vi "Text control 2 v6.3_pump-specific.vi"() -> ()   [LabVIEW 2016]
panel:
  in  "Tab Control":enum32{"Main", "Other parameters"}(tab)
  out "Line running":i32
  out "Total lines":i32
  out "Path":path=path "C:/users/rlp38/09Apr2009LTtesting/test2.txt"
  out "I vs Vg":cluster{"Y data in":dbl[], "X data in":dbl[]}[](graph)
  out "Is max":dbl format="%.2e"
  out "Id max":dbl format="%.2e"
  out "Ig max":dbl format="%.2e"
  out "Imax vs time":cluster{"Y data in":dbl[], "X data in":dbl[]}[](graph)
  out "Imin vs time":cluster{"Y data in":dbl[], "X data in":dbl[]}[](graph)
  out "I vs Vd":cluster{"Y data in":dbl[], "X data in":dbl[]}[](graph)
  in  "Script":string="#-------------------------------------------------------\n# SPM pump cleaning script\n#\n# Version 0.5\n# Author: Dimitrios Simatos\n# Last updated: 2018-01-05\n#-------------------------------------------------------\n# Description\n#\n# This script is designed to run the cleaning sequence of the SPM OEM pump.\n# This script needs to be run 4 times!\n#-------------------------------------------------------\n# Changes\n#\n# Placed initialization and hard stop commands in the beginning.\n#-------------------------------------------------------\n# Important points\n#\n# Never leave any liquid in the pump to dry after the experiments. If they dry, the residue may block the valve.\n# Always run the cleaning cycle after the experiments.\n# Use clockwise rotation when going up in valve port numbers and vice versa.\n#-------------------------------------------------------\n# Things to do before running the script\n#\n# Set time units to minutes.\n# Set filenames.\n# Replace the tubing, if necessary.\n#-------------------------------------------------------\n# Port connections\n#\n# Port 1: Waste\n# Port 2: Waste\n# Port 3: Various cleaning liquids\n# Port 4: Waste\n# Port 5: Waste\n# Port 6: Waste\n#\n# Between each of the 4 runs, the settings of Port 3 will change, according to the cleaning protocol.\n# The settings for Port 3 are:\n# 1st run: 1% v/v solution of sodium hypochlorite in ultrapure water\n# 2nd run: 0.1% w/v solution of sodium dodecyl sulfate in ultrapure water\n# 3rd run: Ultrapure water\n# 4th run: Waste (in air, not immersed in liquid)\n#-------------------------------------------------------\n# Cleaning protocol for the SPM OEM pump (from the manual)\n#\n# A cleaning procedure should be performed at the end of each day or in between two different experiments.\n# An effective cleaning can be performed in the following manner:\n# • Bleach solution to kill microorganisms\n# 1. Prepare a solution of 1% chlorine bleach and deionized water\n#    NOTE: Prepare a 1% v/v solution of sodium hypochlorite in deionized water\n# 2. Prepare a reservoir and place 1 tubing in the bleach solution and 5 tubings in a waste recipient\n# 3. Pick up the bleach solution through 1 port to entirely fill the syringe\n# 4. Sequentially output the syringe content through the remaining ports and throw it to the waste\n# 5. Repeat operation at least 2 times\n# • Detergent solution to remove debris\n# 1. Prepare a solution of 0.1% detergent and deionized water\n#    NOTE: Prepare a 0.1% w/v solution of sodium dodecyl sulfate in deionized water\n# 2. Move the tubing from the bleach solution reservoir and place it into a reservoir of detergent solution\n# 3. Pick up the detergent solution through 1 port to entirely fill the syringe\n# 4. Sequentially output the detergent solution through the remaining ports into the waste recipient\n# 5. Repeat operation at least 2 times\n# • Rinsing water to prepare the pump for your next experiment\n# 1. Move the tubing from the detergent solution reservoir and place it into a reservoir of deionized water\n# 2. Pick up the rinsing solution through 1 port to entirely fill the syringe\n# 3. Sequentially output the rinse water through the remaining ports into the waste recipient\n# 4. Repeat operation at least 2 times\n# • Replace the tubing, if necessary\n#-------------------------------------------------------\n# Pumping cycles and execution time\n#\n# Execution time for a single cycle: 6 x (1 min + 10 sec) = 7 minutes\n# Total execution time: 4 x 7 = 28 minutes\n# Since the script has to run 4 times, the cleaning lasts for: 4 x 28 = 112 minutes\n# Air must be the last to be pumped through the valve, to remove all liquids.\n# There are 4 pumping cycles. Each one draws a different liquid through port 3 and pumps it sequentially through ports 1,2,4,5,6.\n# During the sequential pumping, each port receives 200 ml of liquid (20% of the total syringe volume = 600 \"plunger units\")\n# The device must be disconnected from the port during the cleaning procedure.\n# All cycles are similar, except cycle 1 has the initialization command uncommented and the first report valve command commented.\n#-------------------------------------------------------\n# Volume of liquid needed\n#\n# Volume of liquid needed per cycle: 1 ml\n# Total volume of liquid needed per script run: 4 x 1 = 4 ml\n# Since the script has to run 4 times, the first 3 with different liquids, I need:\n# 4 ml of 1% v/v solution of sodium hypochlorite in ultrapure water\n# 4 ml of 0.1% w/v solution of sodium dodecyl sulfate in ultrapure water\n# 4 ml of ultrapure water\n#-------------------------------------------------------\n# Parameters\n#\n# Syringe size: 1 ml\n# Step resolution N = 0.01 mm\n# Drawing flow V = 300 pulses/second (6000 ul/min)\n# Pumping flow V = 300 pulses/second (6000 ul/min)\n#-------------------------------------------------------\n# Pump initialization\npump /1T #hard stop pump\npump /1ZR #initialize pump\n#-------------------------------------------------------\n# Cycle 1\n# Fill the syringe\npump /1Q #query pump\npump /1? #report absolute plunger position\n#pump /1?6 #report valve position\nwait-min 1 #wait 1 minute\npump /1N0R #set step resolution: 0.01 mm\npump /1Q #query pump\npump /1? #report absolute plunger position (the plunger should be at 0)\npump /1?6 #report valve position\nwait 1000 #wait 1 second\npump /1V300R #choose speed: 300 steps/s (6000 ul/min)\npump /1Q #query pump\nwait 1000 #wait 1 second\npump /1I3R #go to port 3, clockwise rotation\npump /1Q #query pump\npump /1?6 #report valve position\nwait 1000 #wait 1 second\npump /1A3000R #go to absolute position 3000 (= draw 1 ml)\nwait 30000 #wait 30 seconds\npump /1Q #query pump\npump /1? #report absolute plunger position (the plunger should have finished moving)\n#pump /1?6 #report valve position\n# The sequential pumping begins\n# Port 1\npump /1O1R #switch to port 1, counterclockwise rotation\npump /1Q #query pump\npump /1?6 #report valve position\npump /1A2400R #go to absolute position 2400 (= pump 200 ul)\npump /1Q #query pump\npump /1? #report absolute plunger position (the plunger should be moving to 0)\nwait-min 1 #wait 1 minute\npump /1? #report absolute plunger position (the plunger should have finished moving)\n# Port 2\npump /1I2R #switch to port 2, clockwise rotation\npump /1Q #query pump\npump /1?6 #report valve position\npump /1A1800R #go to absolute position 1800 (= pump 200 ul)\npump /1Q #query pump\npump /1? #report absolute plunger position (the plunger should be moving to 0)\nwait-min 1 #wait 1 minute\npump /1? #report absolute plunger position (the plunger should have finished moving)\n# Port 4\npump /1I4R #switch to port 4, clockwise rotation\npump /1Q #query pump\npump /1?6 #report valve position\npump /1A1200R #go to absolute position 1200 (= pump 200 ul)\npump /1Q #query pump\npump /1? #report absolute plunger position (the plunger should be moving to 0)\nwait-min 1 #wait 1 minute\npump /1? #report absolute plunger position (the plunger should have finished moving)\n# Port 5\npump /1I5R #switch to port 5, clockwise rotation\npump /1Q #query pump\npump /1?6 #report valve position\npump /1A600R #go to absolute position 600 (= pump 200 ul)\npump /1Q #query pump\npump /1? #report absolute plunger position (the plunger should be moving to 0)\nwait-min 1 #wait 1 minute\npump /1? #report absolute plunger position (the plunger should have finished moving)\n# Port 6\npump /1I6R #switch to port 6, clockwise rotation\npump /1Q #query pump\npump /1?6 #report valve position\npump /1A0R #go to absolute position 0 (= pump 200 ul)\npump /1Q #query pump\npump /1? #report absolute plunger position (the plunger should be moving to 0)\nwait-min 1 #wait 1 minute\npump /1? #report absolute plunger position (the plunger should have finished moving)\n#-------------------------------------------------------\n# Cycle 2\n# Fill the syringe\n#pump /1ZR #initialize pump\npump /1Q #query pump\npump /1? #report absolute plunger position\npump /1?6 #report valve position\nwait-min 1 #wait 1 minute\npump /1N0R #set step resolution: 0.01 mm\npump /1Q #query pump\npump /1? #report absolute plunger position (the plunger should be at 0)\npump /1?6 #report valve position\nwait 1000 #wait 1 second\npump /1V300R #choose speed: 300 steps/s (6000 ul/min)\npump /1Q #query pump\nwait 1000 #wait 1 second\npump /1O3R #go to port 3, counterclockwise rotation\npump /1Q #query pump\npump /1?6 #report valve position\nwait 1000 #wait 1 second\npump /1A3000R #go to absolute position 3000 (= draw 1 ml)\nwait 30000 #wait 30 seconds\npump /1Q #query pump\npump /1? #report absolute plunger position (the plunger should have finished moving)\n#pump /1?6 #report valve position\n# The sequential pumping begins\n# Port 1\npump /1O1R #switch to port 1, counterclockwise rotation\npump /1Q #query pump\npump /1?6 #report valve position\npump /1A2400R #go to absolute position 2400 (= pump 200 ul)\npump /1Q #query pump\npump /1? #report absolute plunger position (the plunger should be moving to 0)\nwait-min 1 #wait 1 minute\npump /1? #report absolute plunger position (the plunger should have finished moving)\n# Port 2\npump /1I2R #switch to port 2, clockwise rotation\npump /1Q #query pump\npump /1?6 #report valve position\npump /1A1800R #go to absolute position 1800 (= pump 200 ul)\npump /1Q #query pump\npump /1? #report absolute plunger position (the plunger should be moving to 0)\nwait-min 1 #wait 1 minute\npump /1? #report absolute plunger position (the plunger should have finished moving)\n# Port 4\npump /1I4R #switch to port 4, clockwise rotation\npump /1Q #query pump\npump /1?6 #report valve position\npump /1A1200R #go to absolute position 1200 (= pump 200 ul)\npump /1Q #query pump\npump /1? #report absolute plunger position (the plunger should be moving to 0)\nwait-min 1 #wait 1 minute\npump /1? #report absolute plunger position (the plunger should have finished moving)\n# Port 5\npump /1I5R #switch to port 5, clockwise rotation\npump /1Q #query pump\npump /1?6 #report valve position\npump /1A600R #go to absolute position 600 (= pump 200 ul)\npump /1Q #query pump\npump /1? #report absolute plunger position (the plunger should be moving to 0)\nwait-min 1 #wait 1 minute\npump /1? #report absolute plunger position (the plunger should have finished moving)\n# Port 6\npump /1I6R #switch to port 6, clockwise rotation\npump /1Q #query pump\npump /1?6 #report valve position\npump /1A0R #go to absolute position 0 (= pump 200 ul)\npump /1Q #query pump\npump /1? #report absolute plunger position (the plunger should be moving to 0)\nwait-min 1 #wait 1 minute\npump /1? #report absolute plunger position (the plunger should have finished moving)\n#-------------------------------------------------------\n# Cycle 3\n# Fill the syringe\n#pump /1ZR #initialize pump\npump /1Q #query pump\npump /1? #report absolute plunger position\npump /1?6 #report valve position\nwait-min 1 #wait 1 minute\npump /1N0R #set step resolution: 0.01 mm\npump /1Q #query pump\npump /1? #report absolute plunger position (the plunger should be at 0)\npump /1?6 #report valve position\nwait 1000 #wait 1 second\npump /1V300R #choose speed: 300 steps/s (6000 ul/min)\npump /1Q #query pump\nwait 1000 #wait 1 second\npump /1O3R #go to port 3, counterclockwise rotation\npump /1Q #query pump\npump /1?6 #report valve position\nwait 1000 #wait 1 second\npump /1A3000R #go to absolute position 3000 (= draw 1 ml)\nwait 30000 #wait 30 seconds\npump /1Q #query pump\npump /1? #report absolute plunger position (the plunger should have finished moving)\n#pump /1?6 #report valve position\n# The sequential pumping begins\n# Port 1\npump /1O1R #switch to port 1, counterclockwise rotation\npump /1Q #query pump\npump /1?6 #report valve position\npump /1A2400R #go to absolute position 2400 (= pump 200 ul)\npump /1Q #query pump\npump /1? #report absolute plunger position (the plunger should be moving to 0)\nwait-min 1 #wait 1 minute\npump /1? #report absolute plunger position (the plunger should have finished moving)\n# Port 2\npump /1I2R #switch to port 2, clockwise rotation\npump /1Q #query pump\npump /1?6 #report valve position\npump /1A1800R #go to absolute position 1800 (= pump 200 ul)\npump /1Q #query pump\npump /1? #report absolute plunger position (the plunger should be moving to 0)\nwait-min 1 #wait 1 minute\npump /1? #report absolute plunger position (the plunger should have finished moving)\n# Port 4\npump /1I4R #switch to port 4, clockwise rotation\npump /1Q #query pump\npump /1?6 #report valve position\npump /1A1200R #go to absolute position 1200 (= pump 200 ul)\npump /1Q #query pump\npump /1? #report absolute plunger position (the plunger should be moving to 0)\nwait-min 1 #wait 1 minute\npump /1? #report absolute plunger position (the plunger should have finished moving)\n# Port 5\npump /1I5R #switch to port 5, clockwise rotation\npump /1Q #query pump\npump /1?6 #report valve position\npump /1A600R #go to absolute position 600 (= pump 200 ul)\npump /1Q #query pump\npump /1? #report absolute plunger position (the plunger should be moving to 0)\nwait-min 1 #wait 1 minute\npump /1? #report absolute plunger position (the plunger should have finished moving)\n# Port 6\npump /1I6R #switch to port 6, clockwise rotation\npump /1Q #query pump\npump /1?6 #report valve position\npump /1A0R #go to absolute position 0 (= pump 200 ul)\npump /1Q #query pump\npump /1? #report absolute plunger position (the plunger should be moving to 0)\nwait-min 1 #wait 1 minute\npump /1? #report absolute plunger position (the plunger should have finished moving)\n#-------------------------------------------------------\n# Cycle 4\n# Fill the syringe\n#pump /1ZR #initialize pump\npump /1Q #query pump\npump /1? #report absolute plunger position\npump /1?6 #report valve position\nwait-min 1 #wait 1 minute\npump /1N0R #set step resolution: 0.01 mm\npump /1Q #query pump\npump /1? #report absolute plunger position (the plunger should be at 0)\npump /1?6 #report valve position\nwait 1000 #wait 1 second\npump /1V300R #choose speed: 300 steps/s (6000 ul/min)\npump /1Q #query pump\nwait 1000 #wait 1 second\npump /1O3R #go to port 3, counterclockwise rotation\npump /1Q #query pump\npump /1?6 #report valve position\nwait 1000 #wait 1 second\npump /1A3000R #go to absolute position 3000 (= draw 1 ml)\nwait 30000 #wait 30 seconds\npump /1Q #query pump\npump /1? #report absolute plunger position (the plunger should have finished moving)\n#pump /1?6 #report valve position\n# The sequential pumping begins\n# Port 1\npump /1O1R #switch to port 1, counterclockwise rotation\npump /1Q #query pump\npump /1?6 #report valve position\npump /1A2400R #go to absolute position 2400 (= pump 200 ul)\npump /1Q #query pump\npump /1? #report absolute plunger position (the plunger should be moving to 0)\nwait-min 1 #wait 1 minute\npump /1? #report absolute plunger position (the plunger should have finished moving)\n# Port 2\npump /1I2R #switch to port 2, clockwise rotation\npump /1Q #query pump\npump /1?6 #report valve position\npump /1A1800R #go to absolute position 1800 (= pump 200 ul)\npump /1Q #query pump\npump /1? #report absolute plunger position (the plunger should be moving to 0)\nwait-min 1 #wait 1 minute\npump /1? #report absolute plunger position (the plunger should have finished moving)\n# Port 4\npump /1I4R #switch to port 4, clockwise rotation\npump /1Q #query pump\npump /1?6 #report valve position\npump /1A1200R #go to absolute position 1200 (= pump 200 ul)\npump /1Q #query pump\npump /1? #report absolute plunger position (the plunger should be moving to 0)\nwait-min 1 #wait 1 minute\npump /1? #report absolute plunger position (the plunger should have finished moving)\n# Port 5\npump /1I5R #switch to port 5, clockwise rotation\npump /1Q #query pump\npump /1?6 #report valve position\npump /1A600R #go to absolute position 600 (= pump 200 ul)\npump /1Q #query pump\npump /1? #report absolute plunger position (the plunger should be moving to 0)\nwait-min 1 #wait 1 minute\npump /1? #report absolute plunger position (the plunger should have finished moving)\n# Port 6\npump /1I6R #switch to port 6, clockwise rotation\npump /1Q #query pump\npump /1?6 #report valve position\npump /1A0R #go to absolute position 0 (= pump 200 ul)\npump /1Q #query pump\npump /1? #report absolute plunger position (the plunger should be moving to 0)\nwait-min 1 #wait 1 minute\npump /1? #report absolute plunger position (the plunger should have finished moving)\n#-------------------------------------------------------"
  out "Command running:":string
  out "Serial port data":string
  out "Elapsed Time":dbl caption="Elapsed Time (s)"
  in  "Time Units":u16(ring)=1 items=["Seconds", "Minutes", "Hours"]
  in  "Time Offset":dbl caption="Set Start Time (s)"
  in  "Reset":bool
  in  "Auto Reset":bool
  in  "integration time":u32(slide) max=2 step=1 scale=0.0..2.0
  in  "Interrupt scan":bool
  out "Absolute plunger position vs time":cluster{"Y data in":dbl[], "X data in":dbl[]}[](graph)
  out "Valve position vs time":cluster{"Y data in":dbl[], "X data in":dbl[]}[](graph)
  out "Is on":dbl format="%.2e"
  out "Id on":dbl format="%.2e"
  out "Ig on":dbl format="%.2e"
  out "Ion vs time":cluster{"Y data in":dbl[], "X data in":dbl[]}[](graph)
  out "Ioff vs time":cluster{"Y data in":dbl[], "X data in":dbl[]}[](graph)
  out "Ig min":dbl format="%.2e"
  out "Id min":dbl format="%.2e"
  out "Is min":dbl format="%.2e"
  out "Is off":dbl format="%.2e"
  out "Id off":dbl format="%.2e"
  out "Ig off":dbl format="%.2e"
  in  "Integration time (long)":dbl=0.32 min=0.04 max=2.0 step=0.02 format="%.2f"
  in  "Integration time (short)":dbl=0.0019 min=8e-05 max=0.0019 step=8e-05 format="%^.0e"
  in  "Gate: Compliance":dbl=0.001 format="%.8f"
  in  "Drain: Compliance":dbl=0.001 format="%.8f"
  in  "Hard stop pump":bool
  in  "Halt pump":bool
  in  "Interrupt program":bool
  in  "Suffix (script)":string="step_1_up-H2O_initial_script.txt"
  in  "Filename (variable part)":string="step_1_up-H2O_initial_"
  in  "Gate Range\nmode":u16(ring) items=["Auto", "Limited", "Fixed"]
  in  "Gate Range":u8(slide)=6 max=11 scale=0.0..11.0
  in  "Source/Drain\nRange mode":u16(ring) items=["Auto", "Limited", "Fixed"]
  in  "Source/Drain Range":u8(slide)=6 max=11 scale=0.0..11.0
  in  "Panel Controls":T1={"Emergency Stop"=refnum, "TransGraph Max"=1e-05, "Text/Graph (text=false)"=TRUE} {"TransGraph Max" format="%.2e"}
  in  "Panel Controls 2":T2={"Emergency Stop"=refnum, "TransGraph Max"=1e-05, "Text/Graph (text=false)"=TRUE, "TransGraph Min"=1e-11} {"TransGraph Min" format="%.2e"; "TransGraph Max" format="%.2e"}
  in  "SMU4":cluster{"on/off":bool, "Voltage":dbl} {"Voltage" min=-100.0 max=100.0 format="%.2f"}
  in  "Full Reset":bool
  in  "Standby":T3
  out "error out":errorcluster
  in  "Delay before read (ms)":u32=1000
  in  "byte count":u32=64
  in  "Serial End Mode for Reads":u16(ring)=2 items=["None", "LastBit", "TermChar"]
  in  "Timeout (ms)":u32=10000
  in  "Enable Termination\nChar (T)":bool=TRUE
  in  "Termination char\n(0xA = '\\n' = LF)\n(0xD = '\\r' = CR)":u8=13 format="%.0x"
  in  "flow control":u16(ring) items=["None"=0, "XON/XOFF"=1, "RTS/CTS"=2, "DTR/DSR"=4]
  in  "stop bits":u16(ring)=10 items=["1.0"=10, "1.5"=15, "2.0"=20]
  in  "parity":u16(ring) items=["None", "Odd", "Even", "Mark", "Space"]
  in  "data bits":u16=8 min=5 max=8 step=1
  in  "VISA resource name":refnum<visa-resource-name>="COM6"
  in  "baud rate":u32=9600
  out "Timings Indicator":T4
  in  "Timings (overwritten by the Front Panel)":T5={"integration time"=0, "Short/Long integration time"=0.00064, "hold time (sec)"=0.0, "delay time (sec)"=0.0, "Step Time (0 disables)"=0.0, "sweep method"=0, "Pulse period"=0.005, "Base voltage"=0.0, "Pulse width"=0.0005} {"Pulse width" min=0.0005 max=0.1 step=0.0001 format="%.4f"; "Base voltage" format="%^.4e"; "Pulse period" min=0.005 max=1.0 step=0.0001 format="%.4f"; "sweep method" items=["Continuous", "Pulsed"]; "Step Time (0 disables)" format="%.2f"; "delay time (sec)" format="%.4f"; "hold time (sec)" format="%.4f"; "Short/Long integration time" format="%^.0e"; "integration time" scale=0.0..2.0}
  in  "Gate":T6={"Gate Start"=0.0, "Gate Stop"=2.0, "Gate Step (linear only)"=1.0, "Gate Compliance"=0.0001, "Gate PComp"=0.0, "Range mode"=0, "Range"=6} {"Range" max=11 scale=0.0..11.0; "Range mode" items=["Auto", "Limited", "Fixed"]; "Gate PComp" format="%^.2e"; "Gate Compliance" format="%^.2e"; "Gate Step (linear only)" format="%^.4e"; "Gate Stop" format="%^.4e"; "Gate Start" format="%^.4e"}
  in  "Drain 2":T7={"Drain Start"=0.0, "Drain Stop"=2.0, "Drain Compliance"=0.0001, "Drain Step"=1.0, "Drain PComp"=0.0, "Range mode"=0, "Range"=6} {"Range" max=11 scale=0.0..11.0; "Range mode" items=["Auto", "Limited", "Fixed"]; "Drain PComp" format="%^.2e"; "Drain Step" format="%^.4e"; "Drain Compliance" format="%^.2e"; "Drain Stop" format="%^.4e"; "Drain Start" format="%^.4e"}
  # "Syntax:\nitime [s|m|l] time(sec): [s|m|l] determines the integration time setting (small|medium|long) and time sets the value.\nNOTE: The value of the integration time has to be within the range allowed by its category (s|m|l), otherwise, the closest value will be used. (e.g. if the category is set to short but the time value is very long, the actual value used will be the maximum short integration time.\nIntegration times:\n    Short: Default: 640 us. Range: 8E-5 - 1.92E-3 seconds.\n    Medium: Fixed at 1 NPL cycle (0.02 seconds).\n    Long: Default: 16 NPL cycles (0.32 seconds). Range: 2-100 NPL cycles (0.04 seconds - 2 seconds).\ngaterangemode [a|l|f]\ndrainrangemode [a|l|f]\npulsed [on|off] PulsePeriod(sec) PulseBaseVoltage PulseONWidth(sec)\nstandby [on l off]\nwait NumMilliseconds\nwait-min NumMinutes\n# texthere = comment\ntransfer [s|d] VgStart VgStop VgStep VdStart VdStop VdStep\noutput [s|d] VgStart VgStop VgStep VdStart VdStop VdStep\nsample Vg Vd NumSamples Time(s) SampleInterval(s)\nsamplei Idg NumSamples Time(s) SampleInterval(s) VDGcompliance\n100 samples is approximately 13 seconds with medium integration\n# if in doubt use SampleInterval(s) = 0.004\nstressV VG VD IGcompliance IDcompliance Duration(sec)\nstressI IDG VDGcompliance Duration(sec)\nvsu2pulse Bias Duration(s)\npulsedstressV [s|d] VEstop VgON VgOFF Period(s) PulseONwidth(s) Vd\nsample-fpp Vg Vd NumSamples Time\nresample-fpp Vg Vd\ntransfer-fpp [s|d] VgStart VgStop VgStep VdStart VdStop VdStep\noutput-fpp [s|d] VgStart VgStop VgStep VdStart VdStop VdStep\nserial SerialPortCommand\npump SerialPortCommand for the SPM pump\n\nSPM Pump Syntax (<x>: pump number, use 1 if only one pump):\nif the command syntax contains [R], then append the letter R to the command\n/<x>Q: query (a query command should follow each command)\n/<x>Z[R] or /<x>Y[R]: initialize pump\n/<x>N<n>[R] (<n>=0,1): <0> (<1>) microstep 0.01 mm (0.00125 mm) resolution\n/<x>I<n> (<n>=0-6): turn to port number n (clockwise)\n/<x>O<n> (<n>=0-6): turn to port number n (counterclockwise)\n/<x>X: Re-execute last command string\n/<x>G<n>[R] (<n>=0-60000): repeat command sequence (default: 0, 0=loop forever)\n/<x>g: Mark the start of a repeat sequence (max = 10)\n/<x>M<n>[R] (<n>=0-86400000): delay command execution by n milliseconds\n/<x>H: Halt; Pause the sequence after finishing the current move\n/<x>T: Hardstop; Interrupt the current move and suppress it from the sequence\n/<x>A<n>[R] (<n>=0-3000 with N=0, 0-24000 with N=1): absolute position\n/<x>P<n>[R] (<n>=0-3000 with N=0, 0-24000 with N=1): relative pickup\n/<x>D<n>[R] (<n>=0-3000 with N=0, 0-24000 with N=1): relative dispense\n/<x>V<n>[R] (<n>=1-1600 default: 150): set peak speed (pulses/sec)\nNOTE: The lowest speed limit is 1 pulse/sec, not 5, as the manual states.\n/<x>S<n>[R] (<n>=10-40 default: 22): set speed (NOT in pulses/sec, look in manual)\nNOTE: When controlled with absolute position, one does not need to pay special attention to the syringe that is mounted on the pump.\nWithdraw from lower stage (ports 3, 5), dispense from higher stage (ports 2, 4, 6).\nConnect Port 1 to waste."
  # "Time"
  # "1\n2\n3\n4\n5\n6\n7\n8\n9\n10\n11\n12\n13\n14\n15\n16\n17\n18\n19\n20"
  # "Serial port settings"
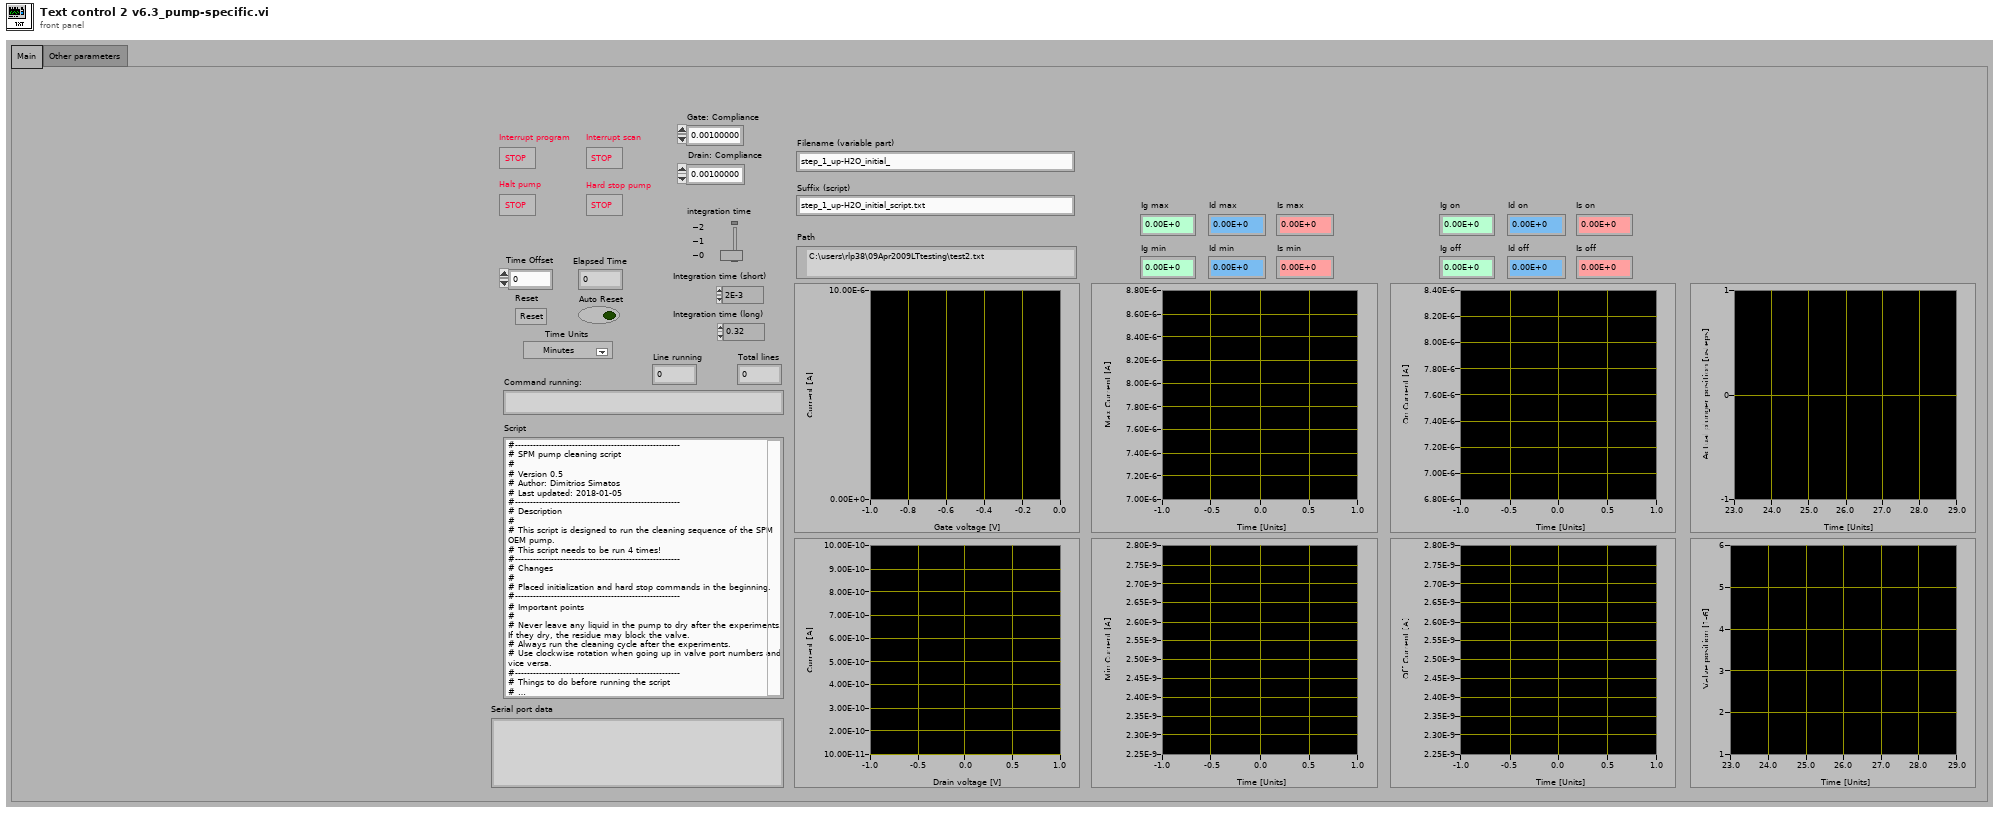
[diagram p1: front panel]
types:
  T1 = cluster{"Emergency Stop":refnum<vi>, "TransGraph Max":dbl, "Text/Graph (text=false)":bool}
  T2 = cluster{"Emergency Stop":refnum<vi>, "TransGraph Max":dbl, "Text/Graph (text=false)":bool, "TransGraph Min":dbl}
  T3 = cluster{"Gate Standby":bool, "Drain Standby":bool}
  T4 = cluster{"integration time (0:s, 1:m, 2:l)":u32, "Short/Long integration time":dbl, "hold time (sec)":dbl, "delay time (sec)":dbl, "Step Time (0 disables)":dbl, "sweep method":u16, "Pulse period":dbl, "Base voltage":dbl, "Pulse width":dbl}
  T5 = cluster{"integration time":u32, "Short/Long integration time":dbl, "hold time (sec)":dbl, "delay time (sec)":dbl, "Step Time (0 disables)":dbl, "sweep method":u16, "Pulse period":dbl, "Base voltage":dbl, "Pulse width":dbl}
  T6 = cluster{"Gate Start":dbl, "Gate Stop":dbl, "Gate Step (linear only)":dbl, "Gate Compliance":dbl, "Gate PComp":dbl, "Range mode":u16, "Range":u8}
  T7 = cluster{"Drain Start":dbl, "Drain Stop":dbl, "Drain Compliance":dbl, "Drain Step":dbl, "Drain PComp":dbl, "Range mode":u16, "Range":u8}
  T8 = enum16{"open", "replace", "create", "open or create", "replace or create", "replace or create with confirmation"}
  T9 = cluster{"V2 Start":dbl, "V2 Step":dbl, "Number of points":i32}
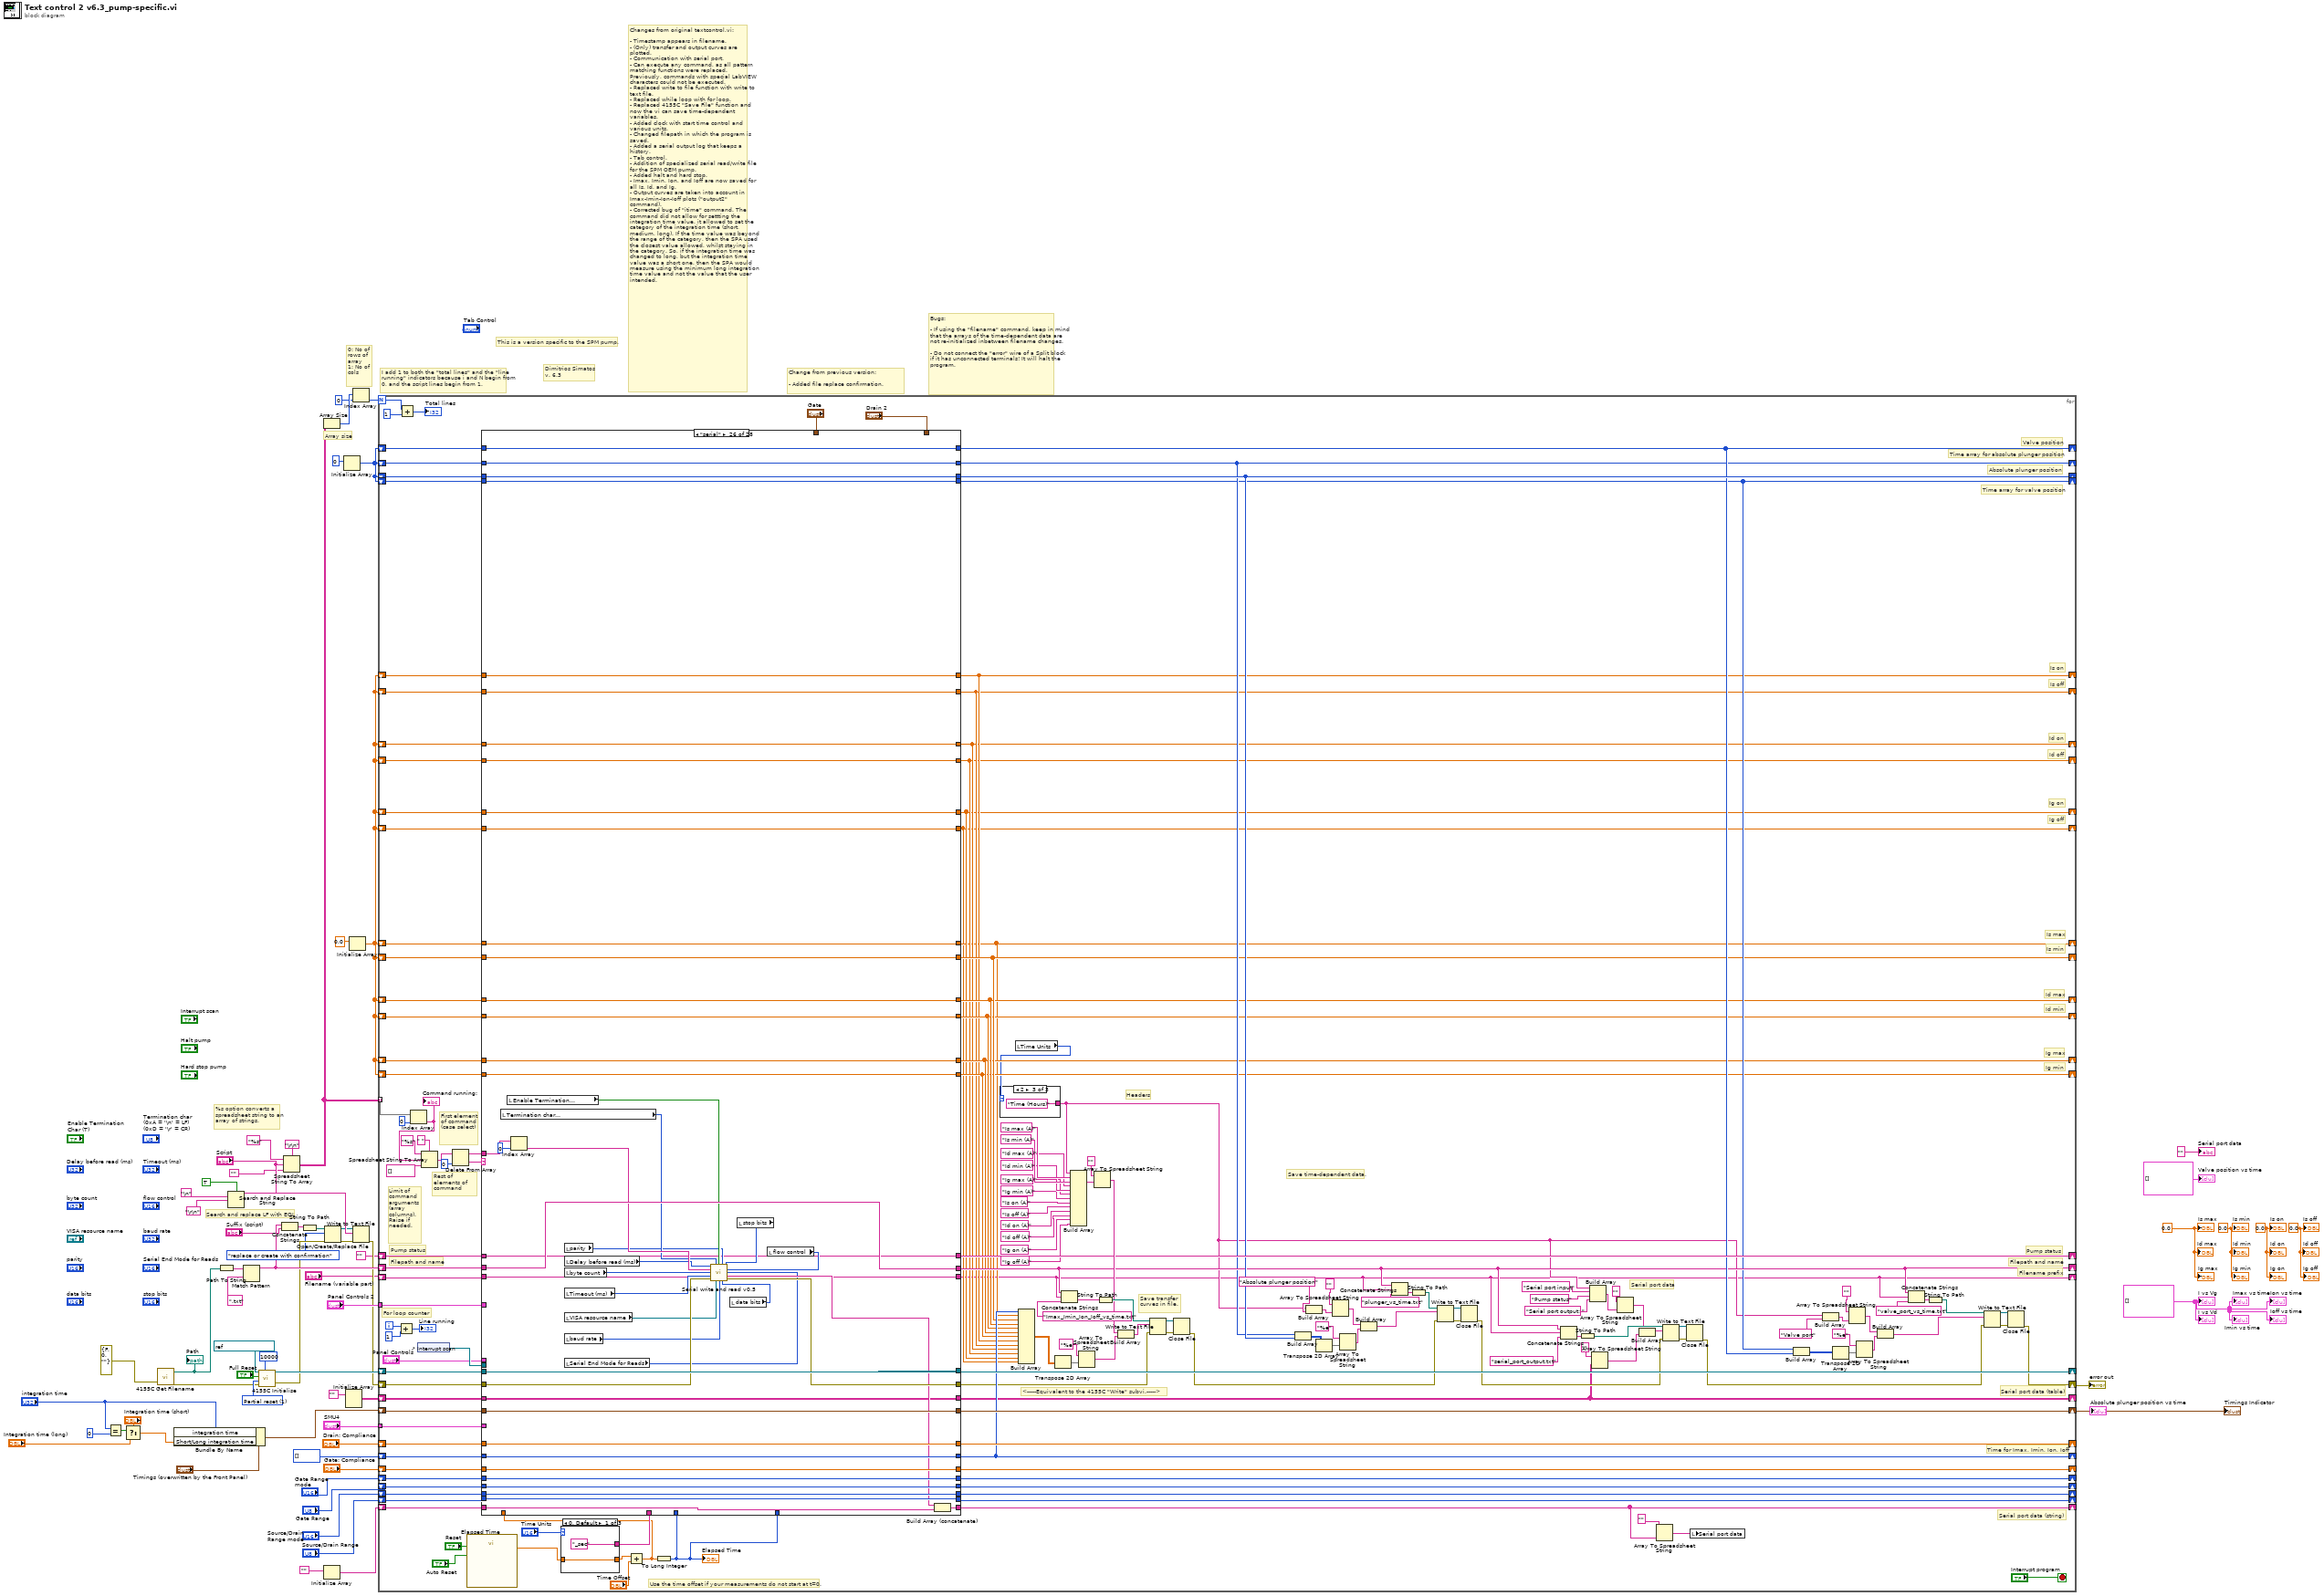
[diagram p0: block diagram]
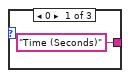
[diagram p2: hidden frame]
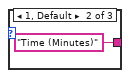
[diagram p3: hidden frame]
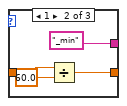
[diagram p4: hidden frame]
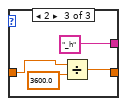
[diagram p5: hidden frame]
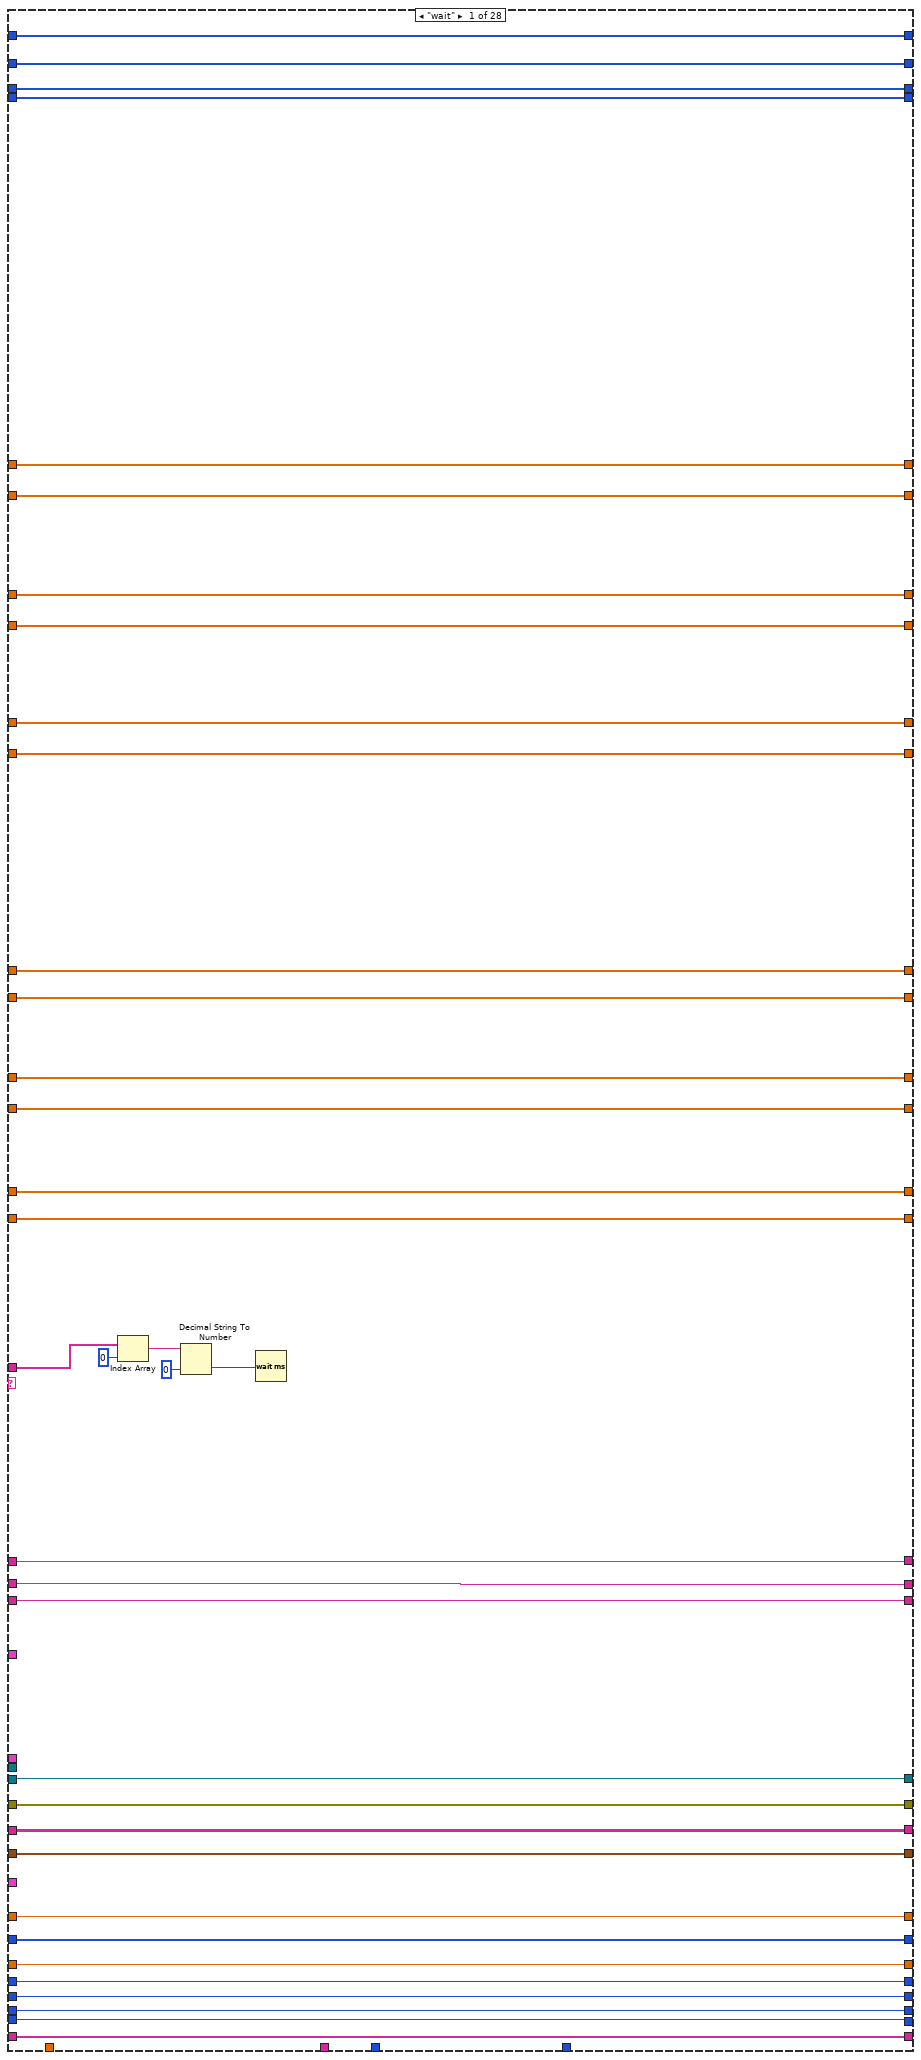
[diagram p6: hidden frame]
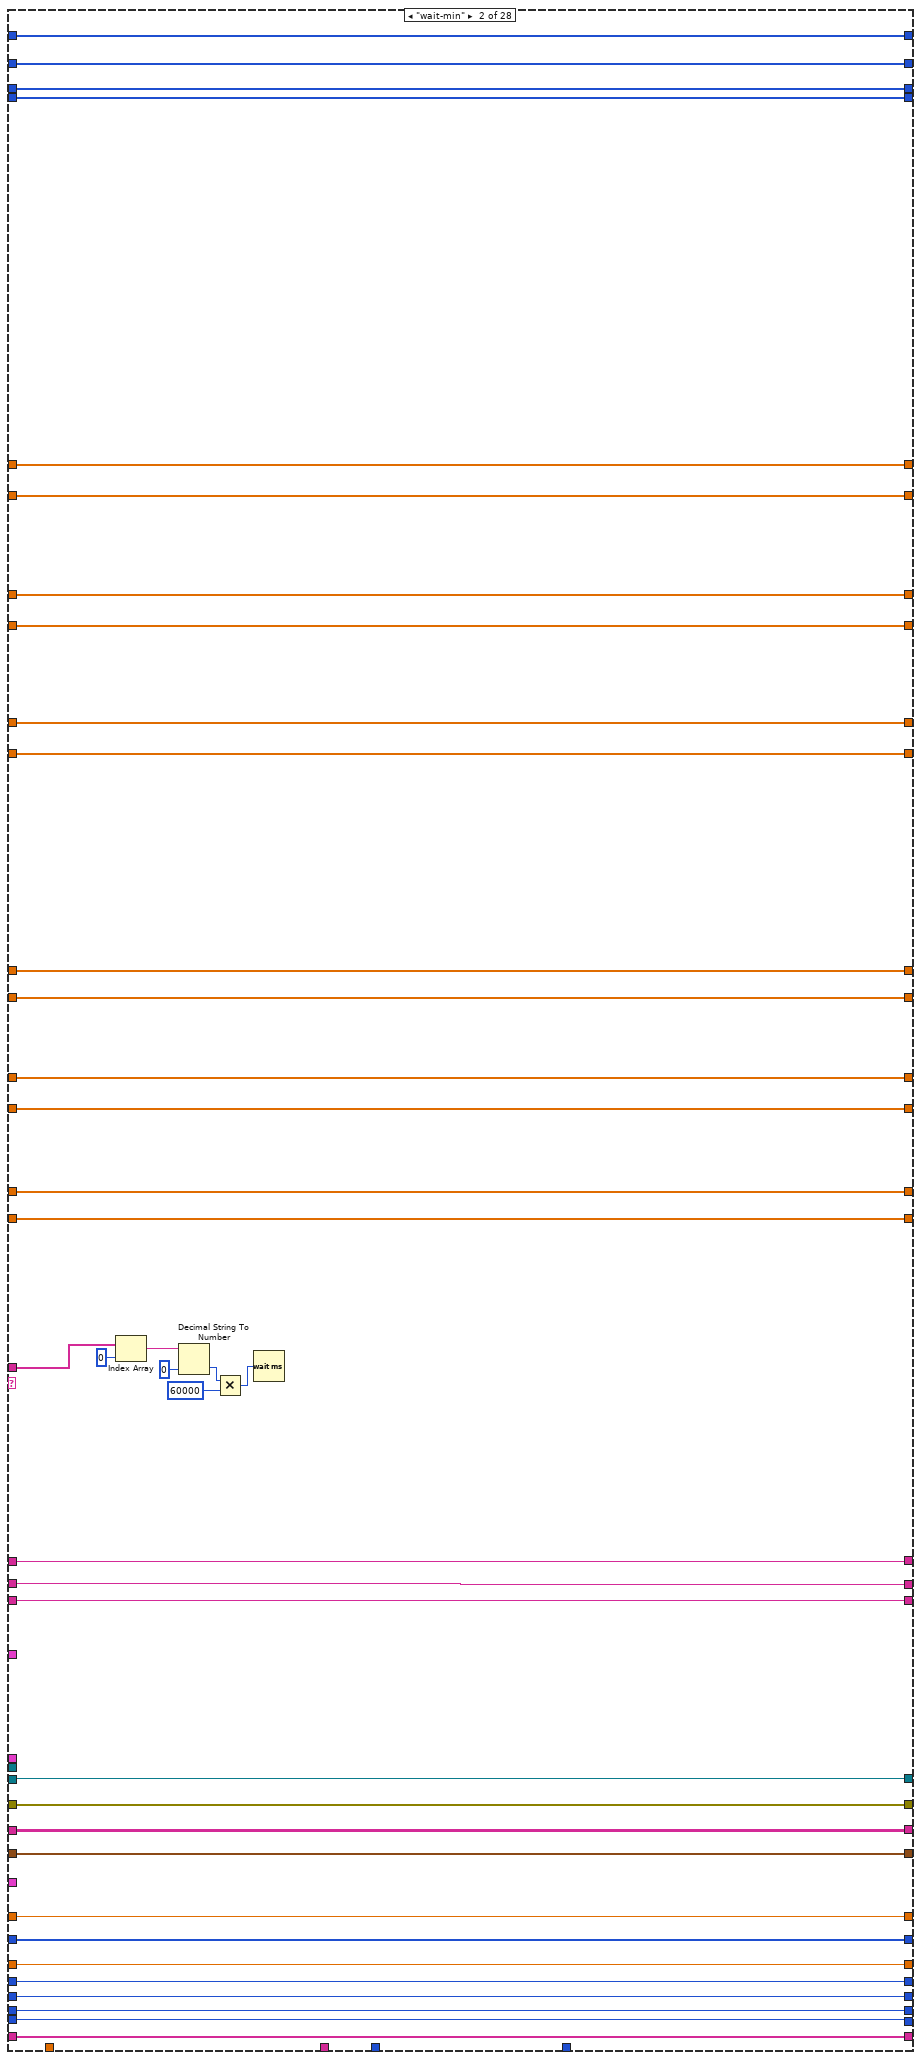
[diagram p7: hidden frame]
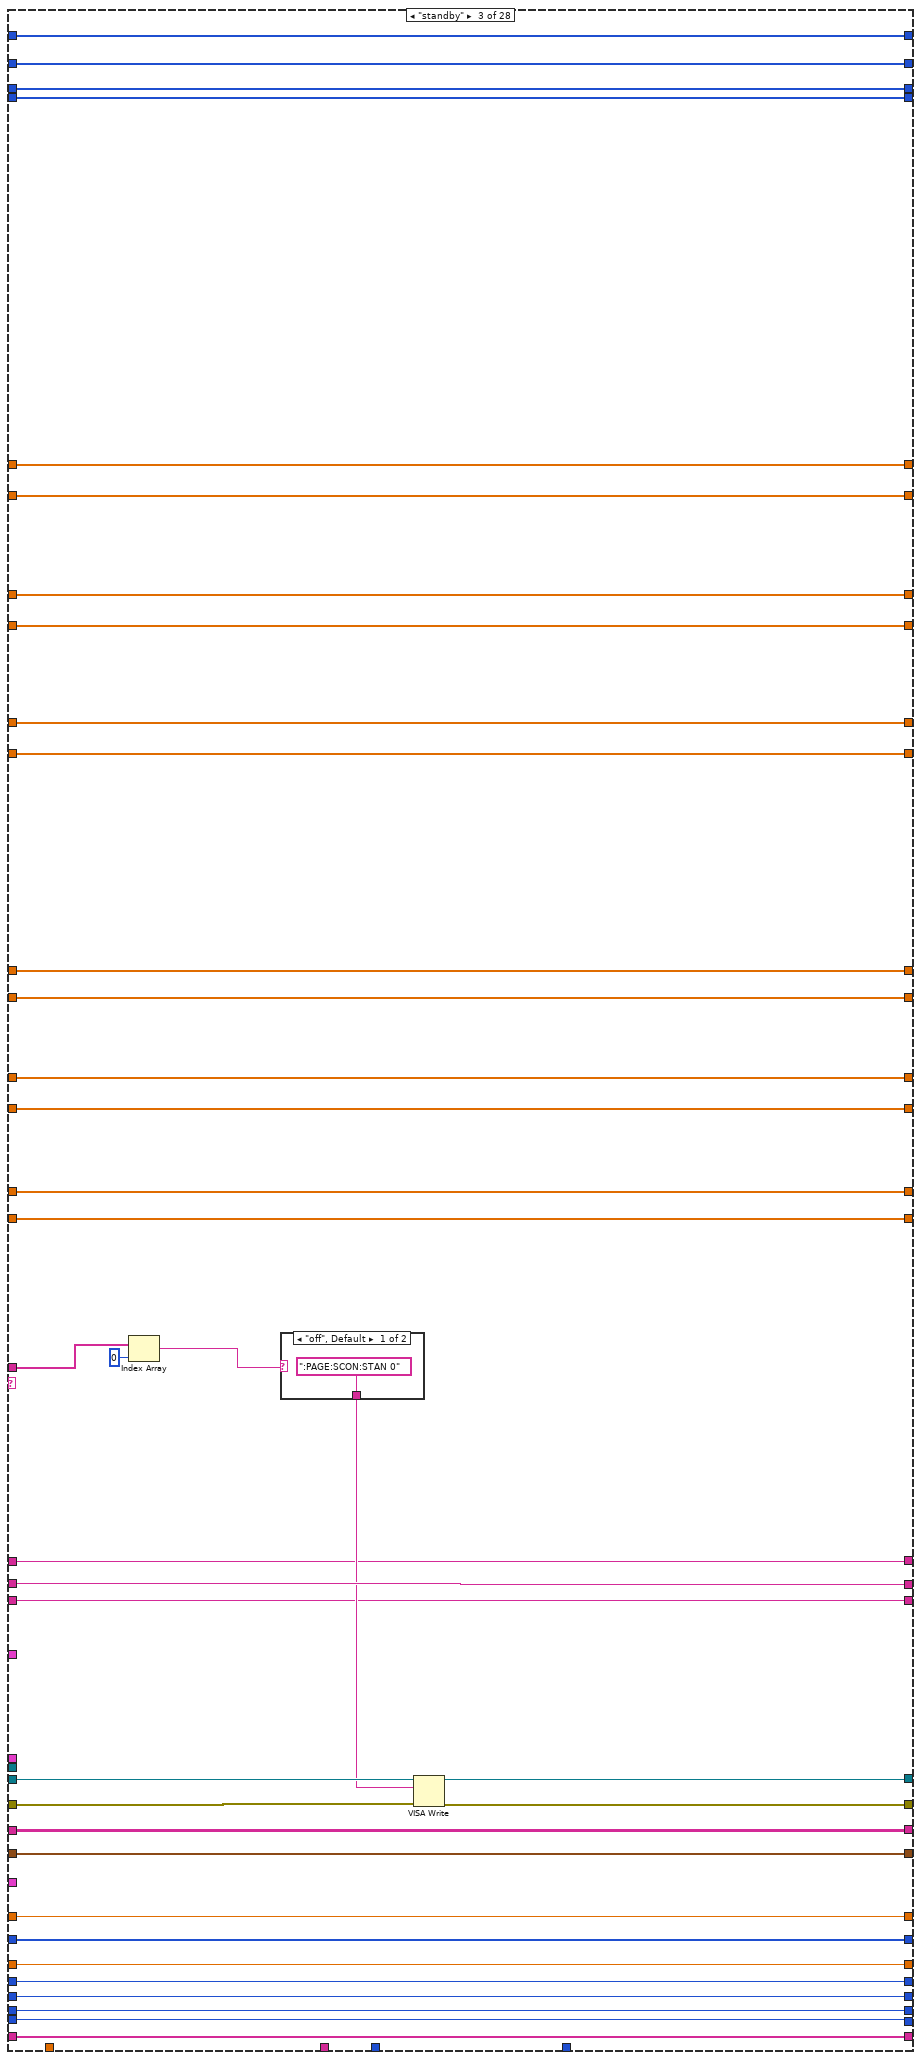
[diagram p8: hidden frame]
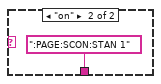
[diagram p9: hidden frame]
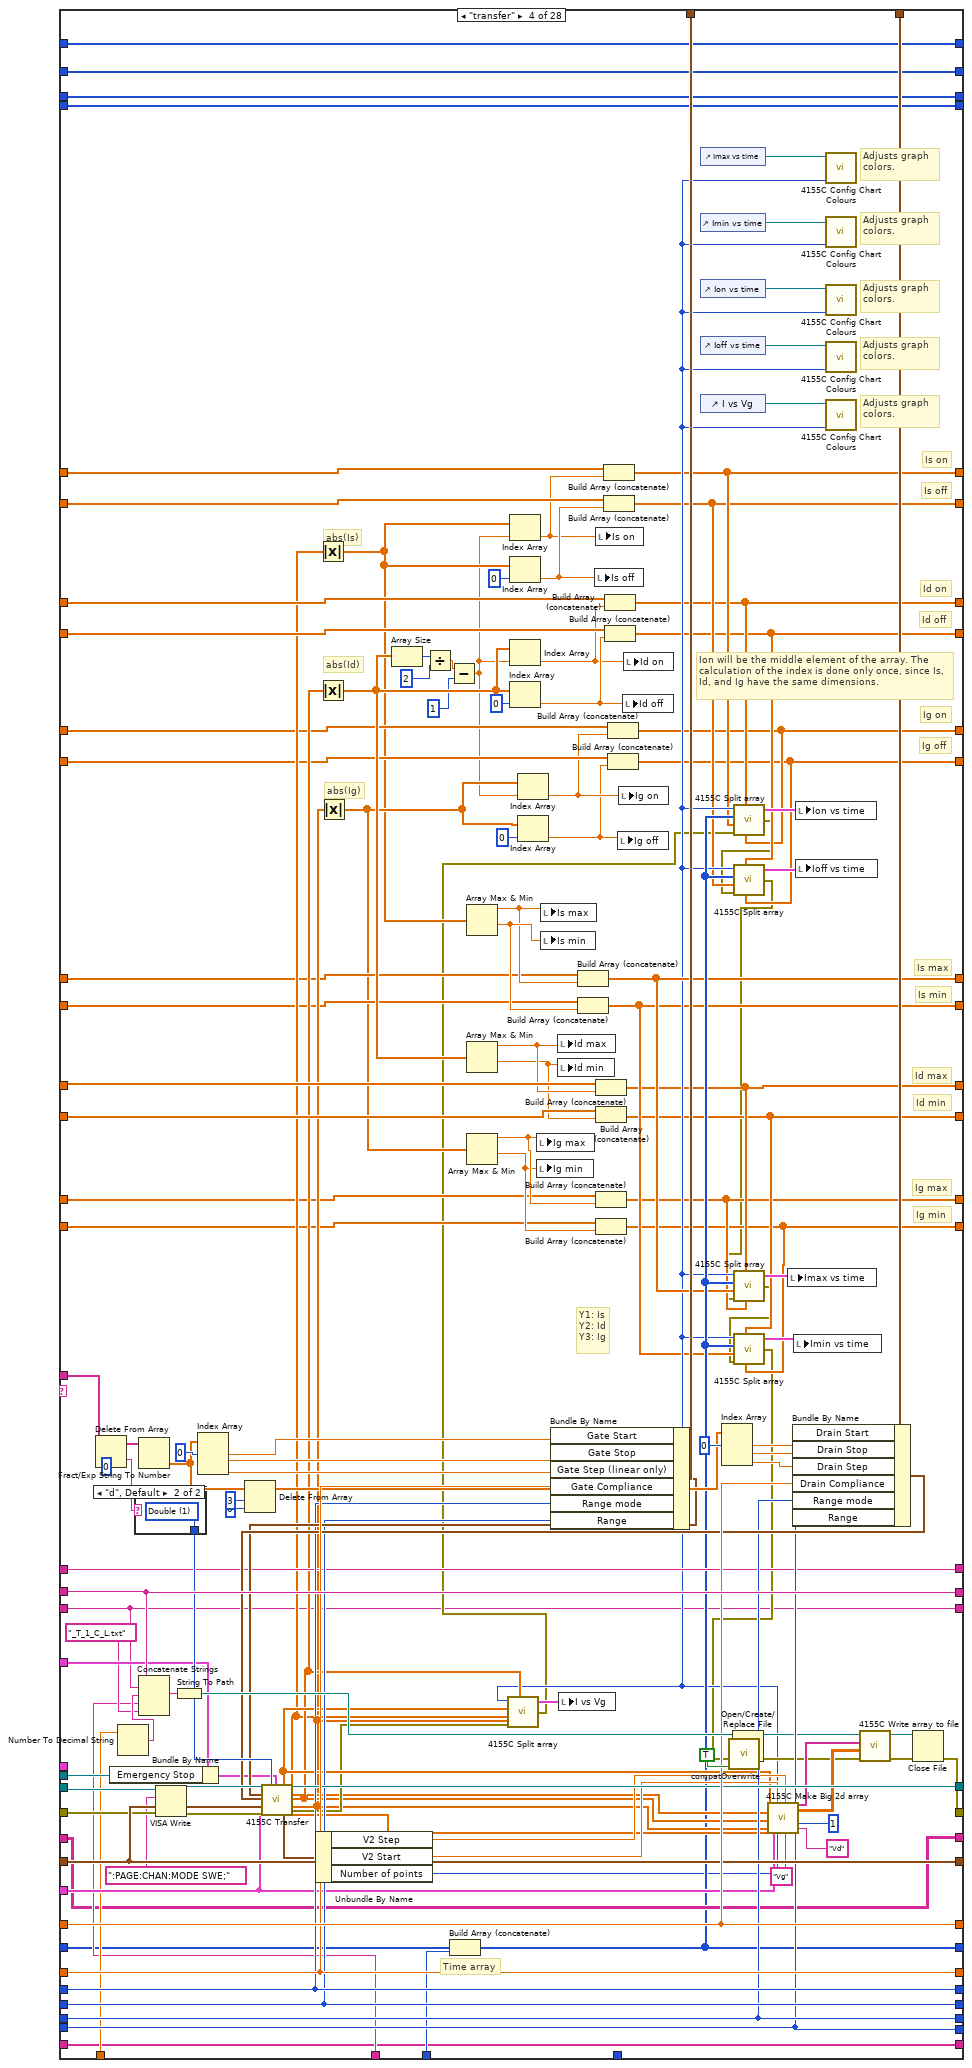
[diagram p10: hidden frame]
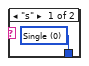
[diagram p11: hidden frame]
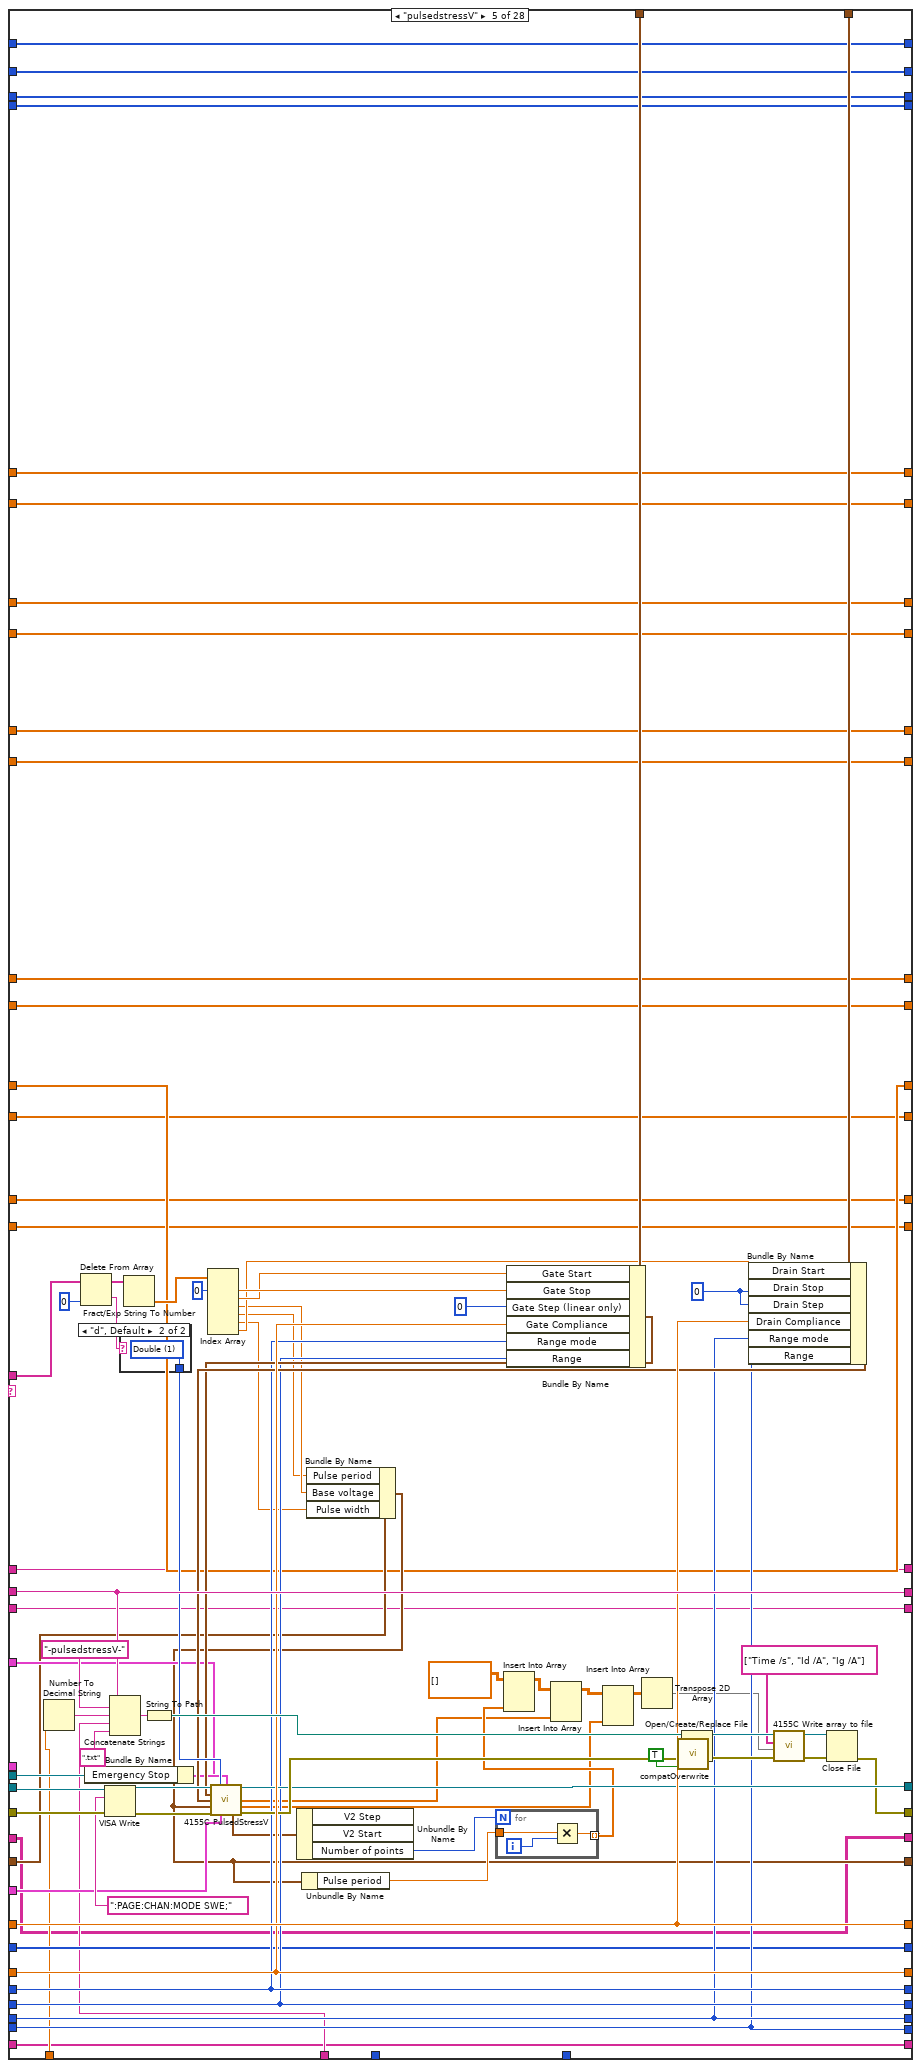
[diagram p12: hidden frame]
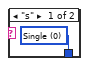
[diagram p13: hidden frame]
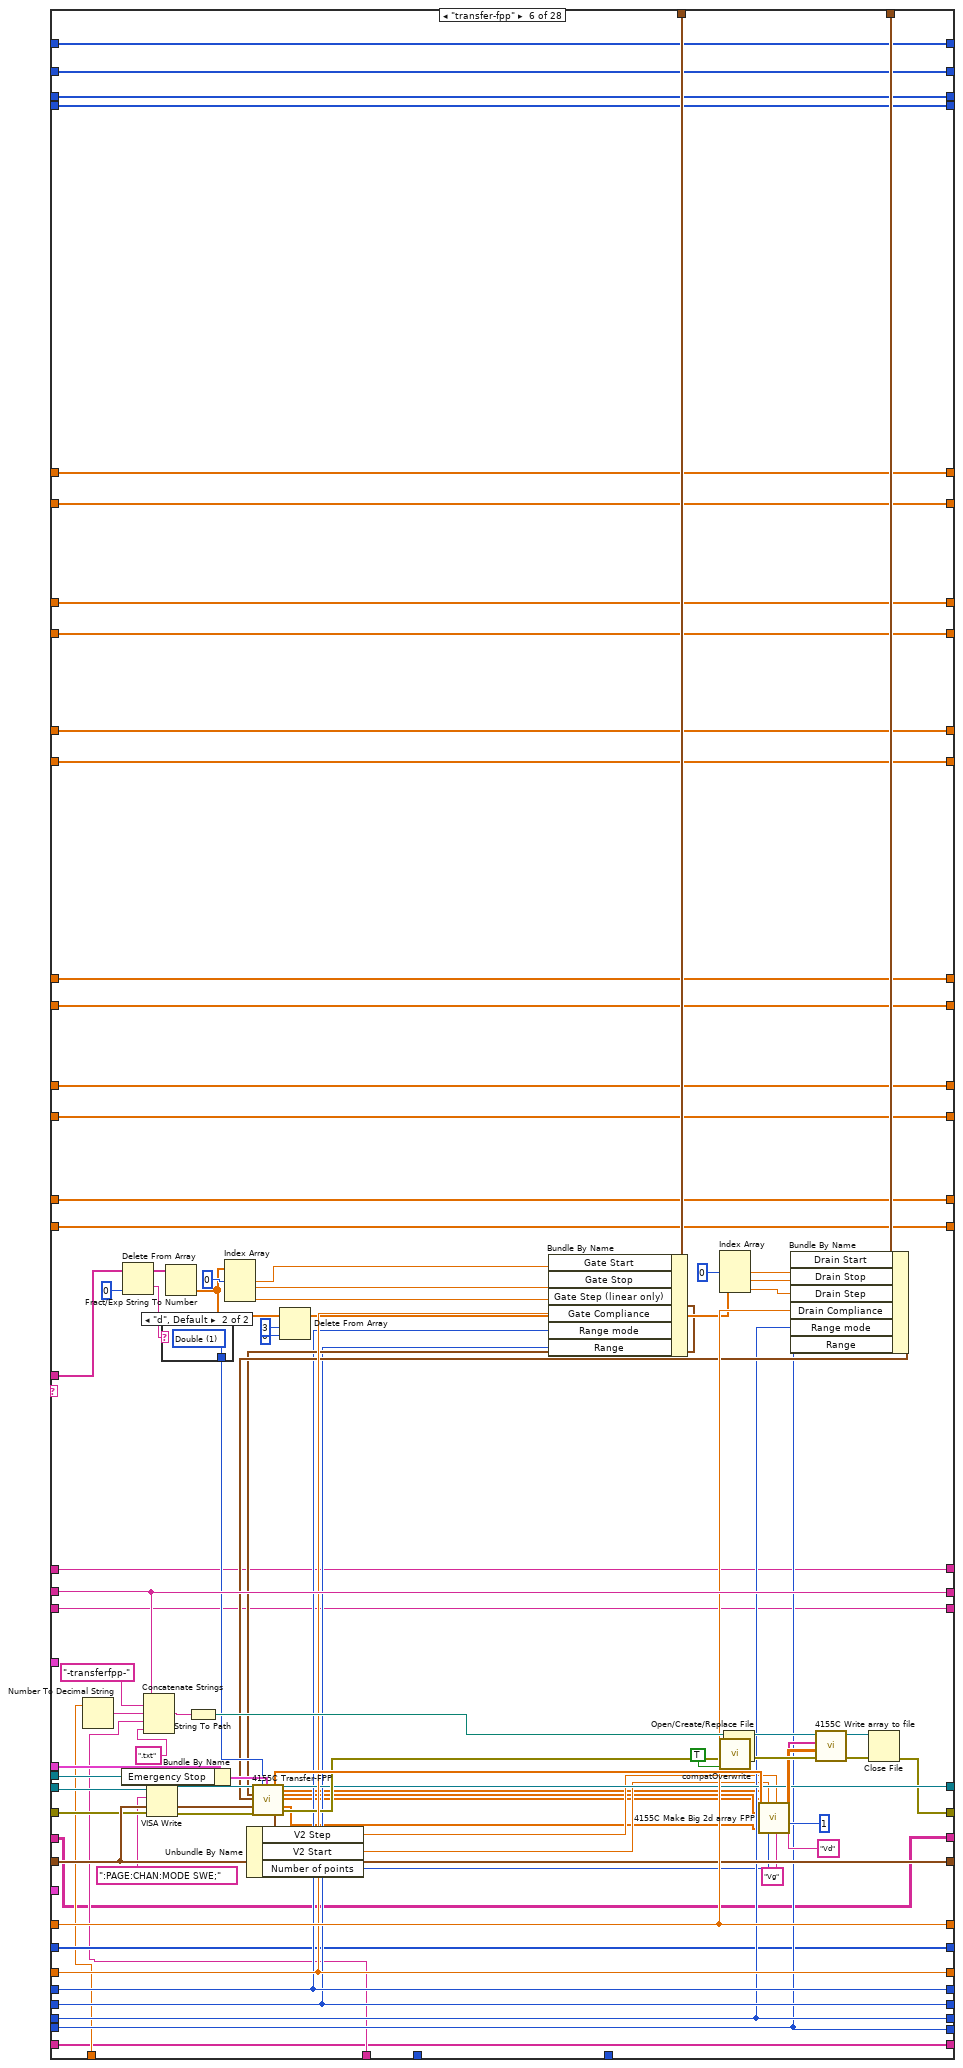
[diagram p14: hidden frame]
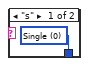
[diagram p15: hidden frame]
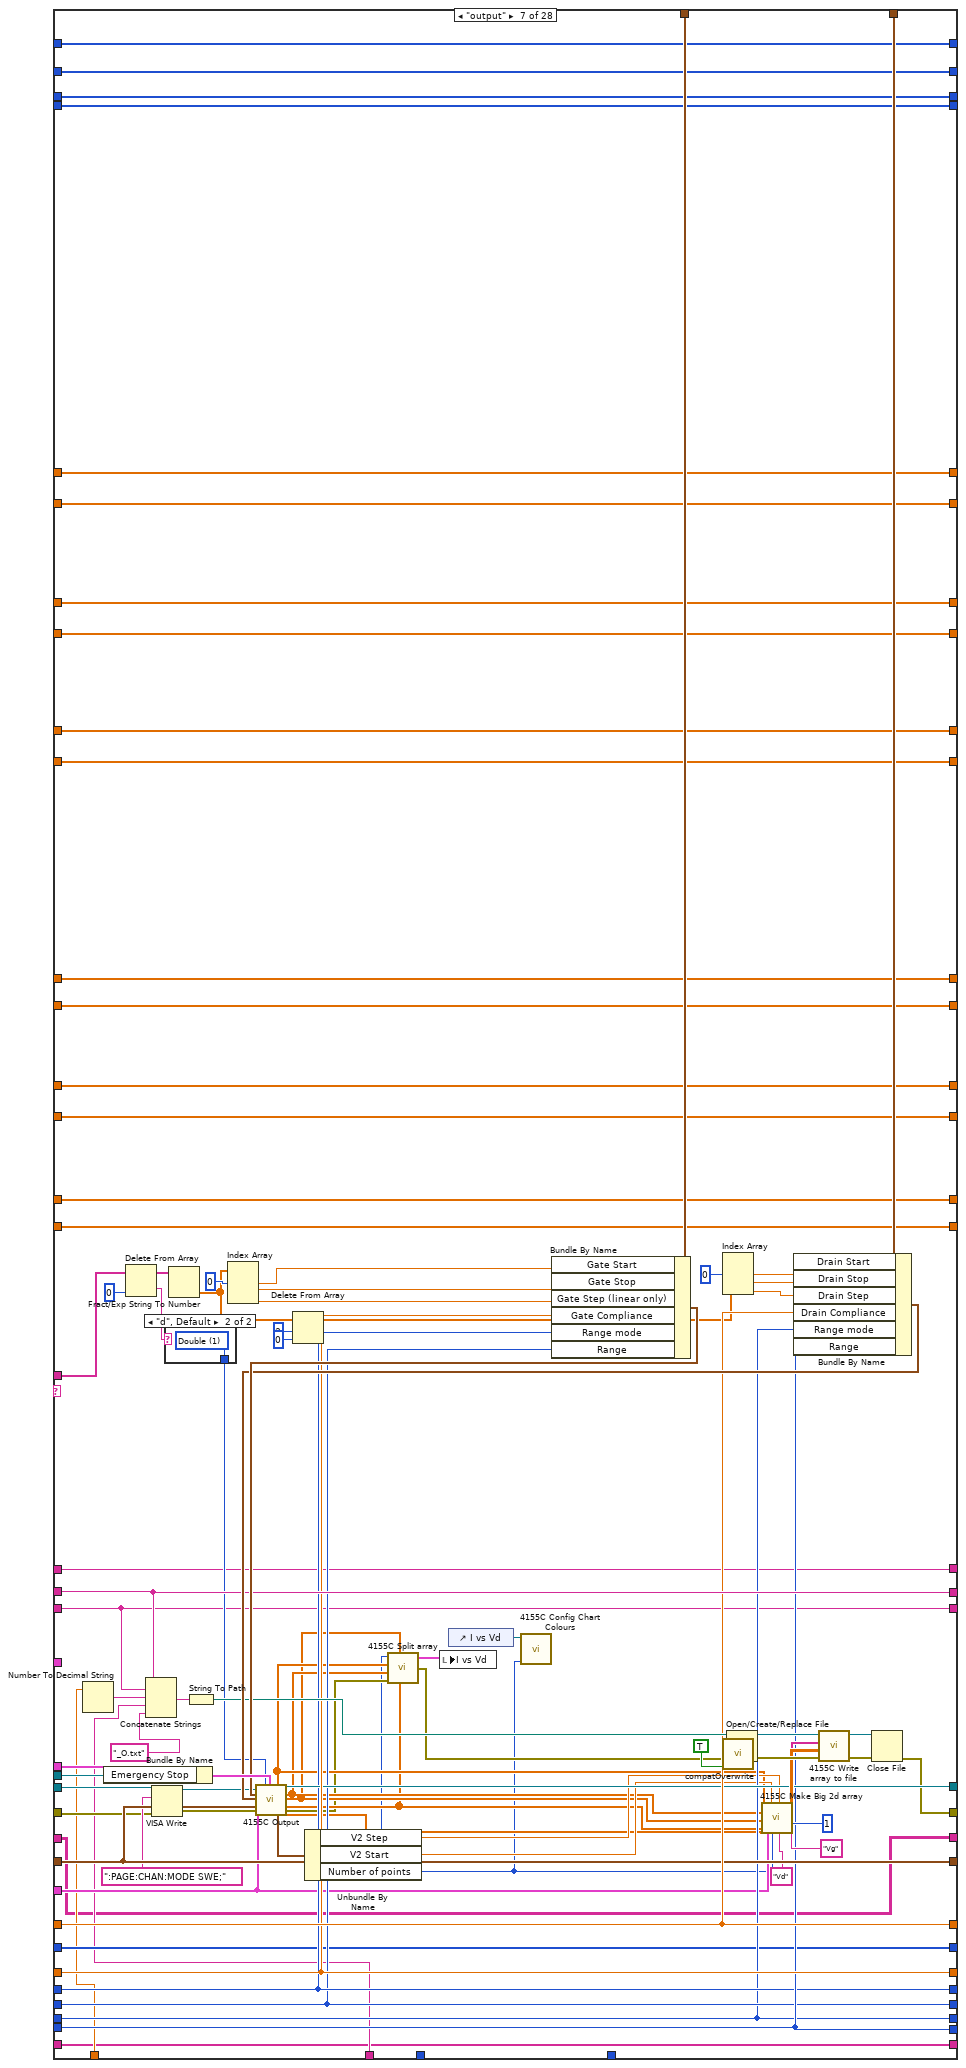
[diagram p16: hidden frame]
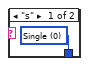
[diagram p17: hidden frame]
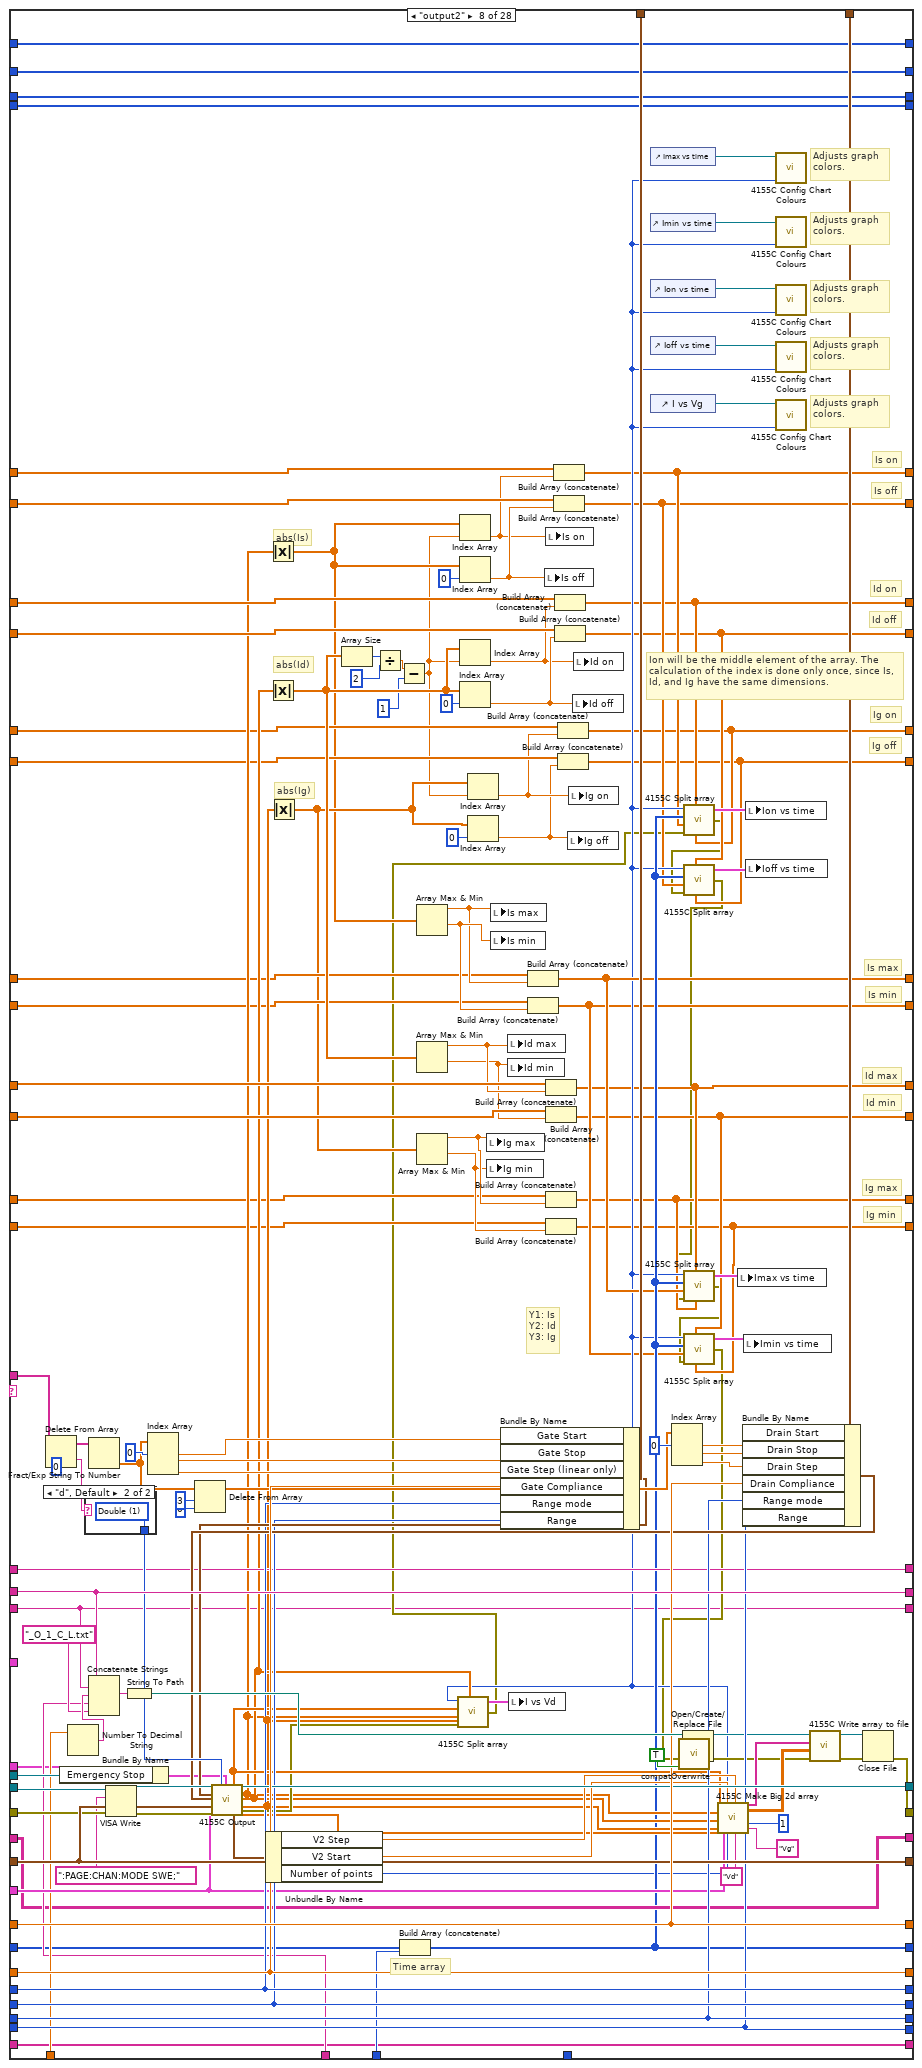
[diagram p18: hidden frame]
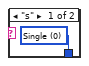
[diagram p19: hidden frame]
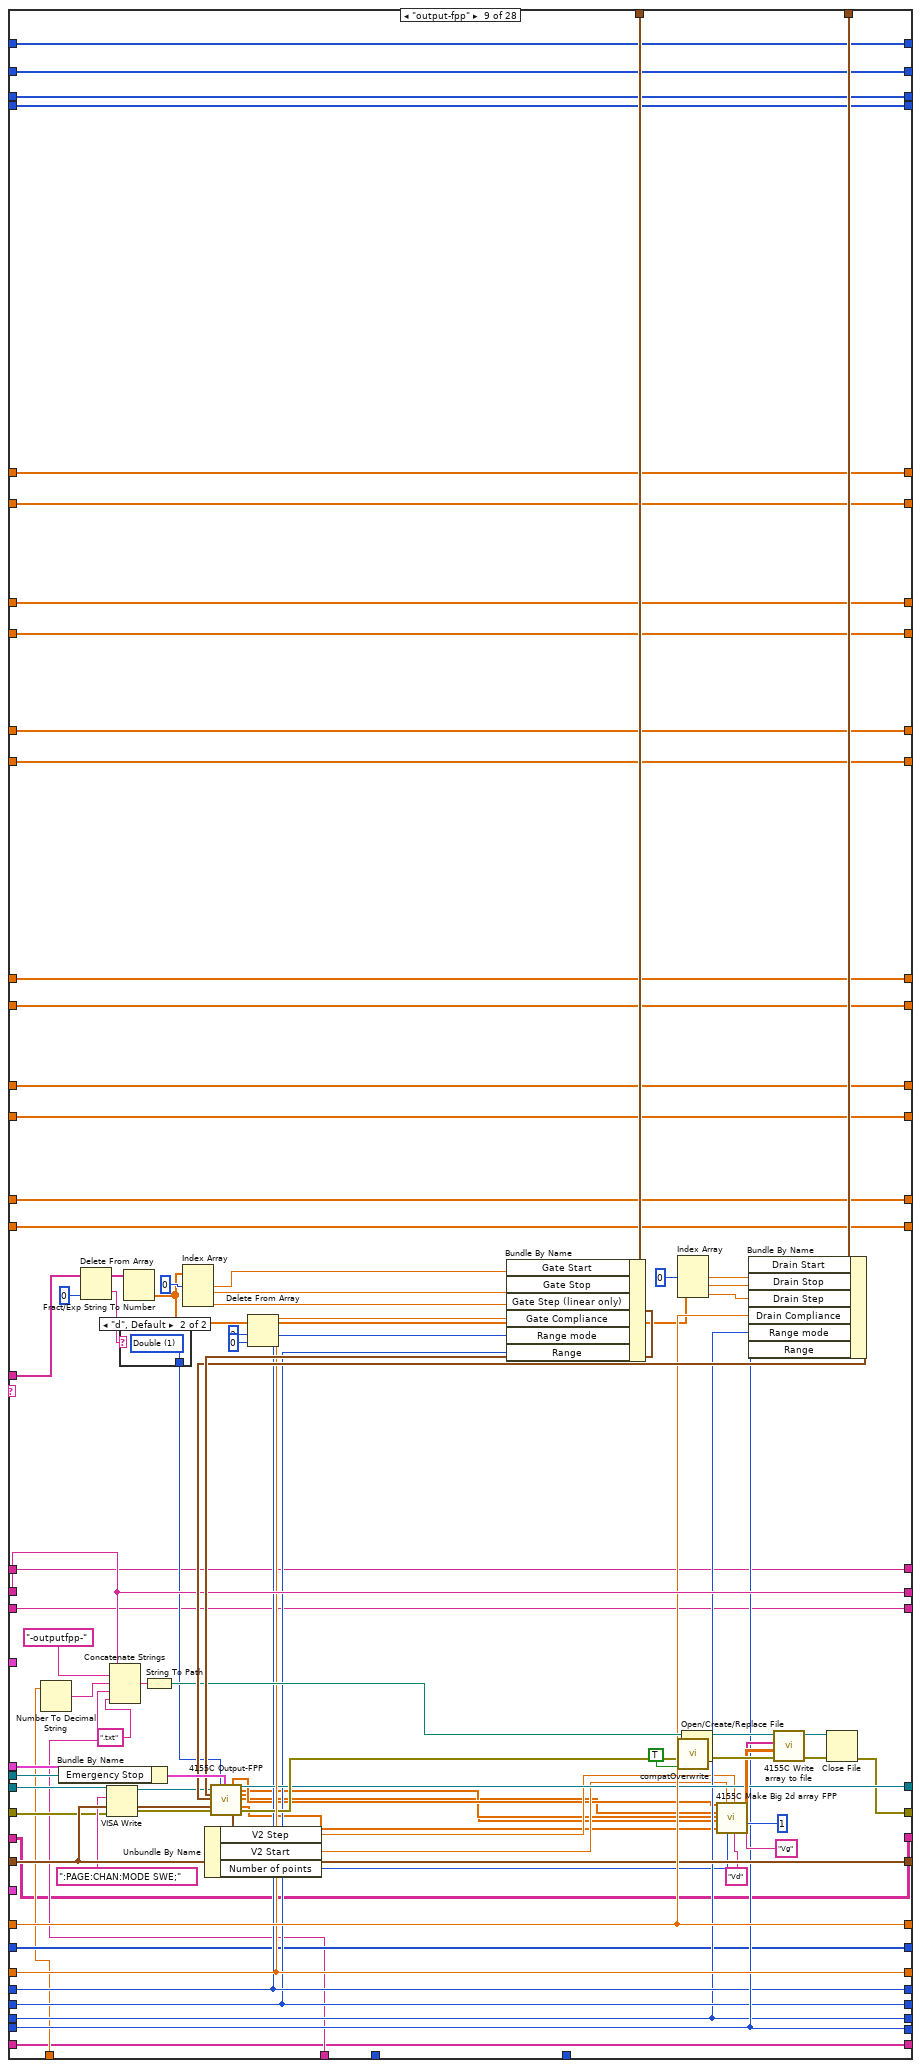
[diagram p20: hidden frame]
diagram:
  w9 = cluster{"Y data in":dbl[], "X data in":dbl[]}[] [] ("I vs Vg")
  w10 = 0.0 ("Is off")
  w11 = 0.0 ("Is on")
  w12 = 0.0 ("Is min")
  w13 = 0.0 ("Is max")
  w62 = u16 1 items=["Reset All", "Partial reset"] ("Type of reset")
  # "Change from previous version:\n\n- Added file replace confirmation."
  # "This is a version specific to the SPM pump."
  # "I add 1 to both the \"total lines\" and the \"line running\" indicators because i and N begin from 0, and the script lines begin from 1."
  # "Bugs:\n\n- If using the \"filename\" command, keep in mind that the arrays of the time-dependent data are not re-initialized inbetween filename changes. \n\n- Do not connect the \"error\" wire of a Split block if it has unconnected terminals! It will halt the program."
  # "Array size"
  # "%s option converts a spreadsheet string to an array of strings."
  # "0: No of rows of array\n1: No of cols"
  # "Dimitrios Simatos\nv. 6.3"
  # "Changes from original textcontrol.vi:\n\n- Timestamp appears in filename.\n- (Only) transfer and output curves are plotted.\n- Communication with serial port.\n- Can execute any command, as all pattern matching functions were replaced. Previously, commands with special LabVIEW characters could not be executed.\n- Replaced write to file function with write to text file.\n- Replaced while loop with for loop.\n- Replaced 4155C \"Save File\" function and now the vi can save time-dependent variables.\n- Added clock with start time control and various units.\n- Changed filepath in which the program is saved.\n- Added a serial output log that keeps a history.\n- Tab control.\n- Addition of specialized serial read/write file for the SPM OEM pump.\n- Added halt and hard stop.\n- Imax, Imin, Ion, and Ioff are now saved for all Is, Id, and Ig.\n- Output curves are taken into account in Imax-Imin-Ion-Ioff plots (\"output2\" command).\n- Corrected bug of \"itime\" command. The command did not allow for settting the integration time value, it allowed to set the category of the integration time (short, medium, long). If the time value was beyond the range of the category, then the SPA used the closest value allowed, whilst staying in the category. So, if the integration time was changed to long, but the integration time value was a short one, then the SPA would measure using the minimum long integration time value and not the value that the user intended."
  # "Search and replace LF with EOL"
  n1 = Equal?(x="integration time", y=u32 0) -> (x = y?=w63:bool)
  n2 = Select(t="Integration time (short)", s=w63, f="Integration time (long)") -> (s? t:f=w14:dbl)
  n3 = call "4155C Get Filename.vi"("error in (no error)"=errorcluster {"status"=FALSE, "code"=0, "source"=""}) -> ("error out"=w57:errorcluster, "path"=w32:path)  [unwired: 2 in, 1 out]
  "Path" <- w32
  n4 = Bundle By Name(cluster="Timings (overwritten by the Front Panel)", "integration time"="integration time", "Short/Long integration time"=w14) -> (w55:T5)
  n5 = Path To String(path=w32) -> (string=w33:string)
  n6 = Search and Replace String(replace all?=TRUE ("replace all? (F)"), input string="Script", search string="\n", replace string="\r\n") -> (result string=w45:string)  [unwired: 4 in, 3 out]
  n7 = Match Pattern(string=w33, regular expression=".txt") -> (before substring=w28:string)  [unwired: 1 in, 3 out]
  n8 = call "4155C Initialise.vi"("VISA resource name in"=refnum<visa-resource-name> "GPIB0::14::INSTR", "Reset"="Full Reset", "Type of reset"=w62, "error in (no error)"=w57, "VISA Timeout Value"=u32 10000) -> ("VISA Resource Name out"=w56:refnum<visa-resource-name>, "error out"=w2:errorcluster)
  n9 = Concatenate Strings(w28, "Suffix (script)") -> (w27:string)
  n10 = Spreadsheet String To Array(delimiter (Tab)="\r\n", format string="%s", spreadsheet string="Script", array type (2D Dbl)="") -> (array=w36:string[][])
  n11 = String To Path(string=w27) -> (path=w5:path)
  n12 = Array Size(array=w36) -> (size(s)=w40:i32[])
  n13 = Initialize Array("") -> (w19:string[])  [unwired: 1 in]
  n14 = Open/Create/Replace File(file path (use dialog)=w5, error in=w2, operation (0:open)=T8."replace or create with confirmation") -> (refnum out=w4:refnum<file>, error out=w3:errorcluster)  [unwired: 3 in, 1 out]
  n15 = Initialize Array(0 ("element")) -> (w21:i32[])  [unwired: 1 in]
  n16 = Initialize Array("") -> (w17:string[][])  [unwired: 2 in]
  n17 = Initialize Array(0.0 ("element")) -> (w23:dbl[])  [unwired: 1 in]
  n18 = Index Array(array=w40, index=0) -> (element=w38:i32)
  n19 = Write to Text File(file (use dialog)=w4, text=w45, error in=w3) -> (error out=w26:errorcluster)  [unwired: 1 in, 2 out]
  n20 = for {
    N: w38 -> [w178]
    tunnel: "SMU4" -> [w214]
    shift-left: "Source/Drain Range" -> [w219]
    shift-right: [w215] -> _
    shift-left: "Source/Drain\nRange mode" -> [w220]
    shift-right: [w216] -> _
    shift-left: "Gate Range" -> [w221]
    shift-right: [w217] -> _
    shift-left: "Gate Range\nmode" -> [w222]
    shift-right: [w218] -> _
    shift-left: "Gate: Compliance" -> [w231]
    shift-right: [w227] -> _
    shift-left: "Drain: Compliance" -> [w232]
    shift-right: [w228] -> _
    shift-left: w55 -> [w233]
    shift-right: [w229] -> w15
    shift-left: w26 -> [w234]
    shift-right: [w124] -> w31
    shift-left: w56 -> [w235]
    shift-right: [w230] -> _
    shift-left: w28 -> [w236]
    shift-right: [w128] -> _
    tunnel: "Panel Controls 2" -> [w213]
    shift-right: [w86] -> _
    shift-left: w23 -> [w212]
    shift-right: [w148] -> _
    shift-left: i32[] [] -> [w208]
    tunnel: w36 -> [w207] mode=indexing
    shift-right: [w85] -> _
    shift-left: w23 -> [w184]
    shift-right: [w118] -> _
    shift-left: w19 -> [w170]
    shift-right: [w149] -> _
    shift-left: w21 -> [w165]
    shift-right: [w130] -> _
    shift-left: w21 -> [w164]
    shift-right: [w163] -> _
    shift-left: "" -> [w162]
    shift-right: [w123] -> _
    shift-left: w21 -> [w145]
    shift-right: [w122] -> _
    shift-left: w21 -> [w129]
    shift-right: [w119] -> _
    shift-left: w17 -> [w121]
    shift-right: [w79] -> _
    shift-left: w23 -> [w107]
    shift-right: [w80] -> _
    shift-left: w23 -> [w106]
    shift-right: [w84] -> _
    shift-left: w23 -> [w95]
    shift-right: [w83] -> _
    shift-left: w23 -> [w94]
    shift-right: [w77] -> _
    shift-left: w23 -> [w93]
    shift-right: [w87] -> _
    shift-left: w23 -> [w92]
    shift-right: [w78] -> _
    shift-left: w23 -> [w91]
    shift-right: [w76] -> _
    shift-left: w23 -> [w90]
    shift-right: [w82] -> _
    shift-left: w23 -> [w89]
    shift-right: [w81] -> _
    shift-left: w23 -> [w88]
    shift-right: [w71] -> _
    shift-left: "Filename (variable part)" -> [w70]
    i -> [w173]
    stop <- "Interrupt program" stop-if-true
    # "Filename prefix"
    # "Is off"
    # "Is on"
    # "Ig off"
    # "Ig on"
    # "Is min"
    # "Is max"
    # "Ig min"
    # "Ig max"
    # "Id min"
    # "Id max"
    # "Id off"
    # "Id on"
    # "Pump status"
    # "Filepath and name"
    # "Pump status"
    # "Limit of command arguments (array columns). Raise if needed."
    # "Serial port data (string)"
    # "Serial port data (table)"
    # "Time array for valve position"
    # "Time array for absolute plunger position"
    # "Valve position"
    # "Absolute plunger position"
    # "Serial port data"
    # "For loop counter"
    # "<-----Equivalent to the 4155C \"Write\" subvi.----->"
    # "Headers"
    # "Save transfer curves in file."
    # "Filepath and name"
    # "Save time-dependent data."
    # "Use the time offset if your measurements do not start at t=0."
    # "Time for Imax, Imin, Ion, Ioff"
    # "Rest of elements of command"
    # "First element of command\n(case select)"
    n21 = Add(x=w173, y=1) -> (x+y=→"Line running":i32)
    n22 = Add(x=w178, y=1) -> (x+y=→"Total lines":i32)
    n23 = Index Array(array=w207, index=0 ("line index")) -> (element=w202:string)
    "Command running:" <- w202
    n24 = control-ref of="Interrupt scan"() -> (w226:refnum<vi>)
    n25 = Spreadsheet String To Array(delimiter (Tab)=" ", format string="%s", spreadsheet string=w202, array type (2D Dbl)=string[] []) -> (array=w200:string[])
    n26 = Delete From Array(array=w200, index=0) -> (deleted portion=w108:string, array with subset deleted=w199:string[])  [unwired: 1 in]
    n27 = call "Elapsed Time"("Reset"="Reset", "Auto Reset"="Auto Reset") -> ("Elapsed Time (s)"=w209:dbl)  [unwired: 10 in, 7 out]
    n28 = case shown="0, Default" "Time Units" {
      tunnel: ["_sec" "_min" "_h"] -> w210
      tunnel: [w240 w244 w247] -> w180
      tunnel: w209 -> [w240 w243 w248]
      frame 0, Default {
      }
      frame 1 {
        n29 = Divide(x=w243, y=60.0) -> (x/y=w244:dbl)
      }
      frame 2 {
        n30 = Divide(x=w248, y=3600.0) -> (x/y=w247:dbl)
      }
    }
    n31 = Add(x=w180, y="Time Offset") -> (x+y=w179:dbl)
    n32 = To Long Integer(number=w179) -> (32bit integer=w146:i32)
    "Elapsed Time" <- w146
    n33 = case shown="\"serial\"" w108 {
      tunnel: w199 -> [w285 w323 w360 w492 w516 w662 w756 w908 w986 w1013 w1093 w1139 w1183 w1223 w1256 _ _ w1417 w1497 _ w1600 w1663 w1724 w1813 w1894 w1933 w2003 w2057]
      tunnel: w236 -> [w280 w319 w358 w499 w581 w670 w763 w915 w994 w1036 w1082 w1131 w1176 w1217 w1249 w1287 w1348 w1395 w1479 w1529 w1587 w1650 w1712 w1807 w1890 w1935 w2005 w2059]
      tunnel: w235 -> [w279 w318 w349 w470 w566 w639 w732 w886 w962 w1037 w1083 w1132 w1177 w1218 w1250 w1292 w1350 w1423 w1503 w1533 w1606 w1669 w1730 w1819 w1848 w1939 w2009 w2061]
      tunnel: w234 -> [w278 w317 w348 w469 w565 w638 w729 w885 w959 w1038 w1084 w1133 w1178 w1219 w1251 w1291 w1321 w1422 w1502 w1532 w1605 w1668 w1729 w1818 w1847 w1938 w2008 w2062]
      tunnel: w233 -> [w277 w316 w357 w495 w541 w666 w759 w911 w990 w1046 w1092 w1130 w1175 w1216 w1248 w1290 w1345 w1386 w1471 w1538 w1580 w1643 w1705 w1806 w1889 w1940 w2010 w2064]
      tunnel: w232 -> [w276 w315 w356 w497 w579 w668 w761 w913 w992 w1045 w1091 w1138 w1182 w1222 w1255 w1289 w1330 w1421 w1501 w1541 w1604 w1667 w1728 w1817 w1898 w1941 w2011 w2065]
      tunnel: w231 -> [w275 w314 w355 w496 w578 w667 w760 w912 w991 w1044 w1090 w1137 w1181 w1221 w1254 w1288 w1331 w1396 w1480 w1540 w1588 w1651 w1713 w1808 w1891 w1943 w2012 w2067]
      tunnel: [w279 w318 w347 w494 w576 w664 w758 w910 w988 w1037 w1083 w1132 w1177 w1218 w1250 w1292 w1350 w1387 w1453 w1531 w1581 w1644 w1706 w1759 w1850 w1939 w2009 w2061] -> w230
      tunnel: [w278 w317 w346 w493 w575 w663 w757 w909 w987 w1038 w1084 w1133 w1178 w1219 w1251 w1291 w1320 w1397 w1454 w1530 w1589 w1652 w1714 w1758 w1849 w1937 w2007 w2062] -> w144
      tunnel: [w277 w316 w357 w495 w537 w666 w759 w911 w990 w1039 w1085 w1130 w1175 w1216 w1248 w1290 w1345 w1386 w1471 w1538 w1580 w1643 w1705 w1806 w1889 w1940 w2010 w2064] -> w229
      tunnel: [w276 w315 w356 w497 w579 w668 w761 w913 w992 w1045 w1091 w1138 w1182 w1222 w1255 w1289 w1330 w1421 w1501 w1541 w1604 w1667 w1728 w1817 w1898 w1941 w2011 w2065] -> w228
      tunnel: [w275 w314 w355 w496 w578 w667 w760 w912 w991 w1044 w1090 w1137 w1181 w1221 w1254 w1288 w1331 w1396 w1480 w1540 w1588 w1651 w1713 w1808 w1891 w1943 w2012 w2067] -> w227
      tunnel: [w280 w319 w358 w499 w581 w670 w763 w915 w994 w1036 w1082 w1131 w1176 w1217 w1249 w1287 w1348 w1395 w1479 w1529 w1587 w1650 w1712 w1807 w1890 w1935 w2005 w2059] -> w128
      tunnel: w226 -> [_ _ _ w501 w585 w675 w766 w917 w998 _ _ _ _ _ _ _ _ w1392 w1476 _ w1586 w1649 w1711 w1779 w1866 _ _ _]
      tunnel: "Gate" -> [_ _ _ w479 w569 w649 w743 w895 w973 _ _ _ _ _ _ _ _ _ _ _ _ _ _ _ _ _ _ _]
      tunnel: "Drain 2" -> [_ _ _ w478 w568 w648 w742 w894 w972 _ _ _ _ _ _ _ _ _ _ _ _ _ _ _ _ _ _ _]
      tunnel: "Panel Controls" -> [_ _ _ _ _ w647 w741 w779 w971 _ _ _ _ _ _ _ _ _ _ _ _ _ _ _ _ _ _ _]
      tunnel: w222 -> [w274 w313 w354 w463 w559 w632 w727 w879 w957 w1043 w1089 _ w1174 w1215 w1247 w1286 w1332 w1382 w1467 w1534 w1576 w1639 w1701 w1802 w1885 w1944 w2013 w2068]
      tunnel: w221 -> [w273 w312 w353 w462 w558 w631 w726 w878 w956 w1042 w1088 w1136 _ w1206 w1253 w1285 w1333 w1383 w1468 w1535 w1577 w1640 w1702 w1803 w1886 w1945 w2014 w2069]
      tunnel: w220 -> [w272 w311 w352 w461 w557 w630 w725 w877 w955 w1041 w1087 w1135 w1180 w1220 _ w1284 w1334 w1384 w1469 w1536 w1578 w1641 w1703 w1804 w1887 w1946 w2015 w2070]
      tunnel: w219 -> [w271 w310 w351 w460 w556 w629 w728 w876 w958 w1040 w1086 w1134 w1179 _ w1252 w1283 w1335 w1385 w1470 w1537 w1579 w1642 w1704 w1805 w1888 w1947 w2016 w2071]
      tunnel: [w274 w313 w354 w463 w559 w632 w727 w879 w957 w1043 w1089 w1129 w1174 w1215 w1247 w1286 w1332 w1382 w1467 w1534 w1576 w1639 w1701 w1802 w1885 w1944 w2013 w2068] -> w218
      tunnel: [w273 w312 w353 w462 w558 w631 w726 w878 w956 w1042 w1088 w1136 w1166 w1206 w1253 w1285 w1333 w1383 w1468 w1535 w1577 w1640 w1702 w1803 w1886 w1945 w2014 w2069] -> w217
      tunnel: [w272 w311 w352 w461 w557 w630 w725 w877 w955 w1041 w1087 w1135 w1180 w1220 w1246 w1284 w1334 w1384 w1469 w1536 w1578 w1641 w1703 w1804 w1887 w1946 w2015 w2070] -> w216
      tunnel: [w271 w310 w351 w460 w556 w629 w728 w876 w958 w1040 w1086 w1134 w1179 w1207 w1252 w1283 w1335 w1385 w1470 w1537 w1579 w1642 w1704 w1805 w1888 w1947 w2016 w2071] -> w215
      tunnel: w214 -> [_ _ _ w455 w553 _ w721 w871 _ _ _ _ _ _ _ _ _ _ _ _ _ _ _ _ _ _ _ _]
      tunnel: w213 -> [_ _ _ w453 w552 _ _ _ _ _ _ _ _ _ _ _ _ _ _ _ _ _ _ _ _ _ _ _]
      tunnel: [w270 w306 w344 w381 w529 w619 w718 w798 w944 w1035 w1080 w1128 w1165 w1205 w1245 w1282 w1316 w1374 w1432 w1528 w1565 w1632 w1695 w1756 w1843 w1936 w2006 w2076] -> w86
      tunnel: w212 -> [w270 w306 w344 w450 w529 w619 w718 w867 w944 w1035 w1080 w1128 w1165 w1205 w1245 w1282 w1316 w1374 w1432 w1528 w1565 w1632 w1695 w1756 w1843 w1936 w2006 w2076]
      tunnel: w179 -> [_ _ _ w447 w526 w617 w715 w864 w941 _ _ _ _ _ _ _ w1314 w1372 w1449 _ w1562 w1629 w1692 w1753 w1839 _ _ _]
      tunnel: w210 -> [_ _ _ w444 w525 w615 w714 w861 w940 _ _ _ _ _ _ _ w1312 w1370 w1448 _ w1561 w1628 w1691 w1752 w1840 _ w1974 _]
      tunnel: w146 -> [_ _ _ w439 _ _ _ w856 _ _ _ _ _ _ _ _ _ _ _ _ _ _ _ _ _ _ w1977 _]
      tunnel: [w269 w305 w343 w389 w528 w618 w717 w806 w943 w1034 w1079 w1127 w1164 w1204 w1244 w1281 w1315 w1373 w1451 w1527 w1564 w1631 w1694 w1755 w1842 w1942 w1986 w2066] -> w148
      tunnel: w208 -> [w269 w305 w343 w443 w528 w618 w717 w860 w943 w1034 w1079 w1127 w1164 w1204 w1244 w1281 w1315 w1373 w1451 w1527 w1564 w1631 w1694 w1755 w1842 w1942 w1986 w2066]
      tunnel: [w268 w304 w342 w380 w524 w614 w713 w797 w939 w1033 w1078 w1126 w1163 w1203 w1243 w1280 w1311 w1369 w1431 w1526 w1560 w1627 w1690 w1751 w1838 w1931 w2002 w2075] -> w85
      tunnel: w184 -> [w268 w304 w342 w437 w524 w614 w713 w854 w939 w1033 w1078 w1126 w1163 w1203 w1243 w1280 w1311 w1369 w1431 w1526 w1560 w1627 w1690 w1751 w1838 w1931 w2002 w2075]
      tunnel: [w267 w303 w341 w430 w523 w613 w703 w847 w938 w1032 w1077 w1125 w1162 w1202 w1242 w1279 w1310 w1368 w1447 w1525 w1559 w1626 w1689 w1750 w1837 w1930 w2001 w2072] -> w118
      tunnel: w170 -> [w267 w303 w341 w430 w523 w613 w703 w847 w938 w1032 w1077 w1125 w1162 w1202 w1242 w1279 w1310 w1368 w1447 w1525 w1559 w1626 w1689 w1750 w1837 w1929 w1975 w2072]
      tunnel: [w266 w302 w340 w429 w522 w612 w702 w846 w937 w1031 w1076 w1124 w1161 w1201 w1241 w1278 w1309 w1367 w1446 w1524 w1558 w1625 w1688 w1749 w1836 w1915 w1988 w2086] -> w149
      tunnel: w165 -> [w266 w302 w340 w429 w522 w612 w702 w846 w937 w1031 w1076 w1124 w1161 w1201 w1241 w1278 w1309 w1367 w1446 w1524 w1558 w1625 w1688 w1749 w1836 w1915 w1987 w2086]
      tunnel: [w265 w301 w339 w428 w521 w611 w701 w845 w936 w1030 w1075 w1123 w1160 w1200 w1240 w1277 w1308 w1366 w1445 w1523 w1557 w1624 w1687 w1748 w1835 w1914 w1970 w2088] -> w130
      tunnel: w164 -> [w265 w301 w339 w428 w521 w611 w701 w845 w936 w1030 w1075 w1123 w1160 w1200 w1240 w1277 w1308 w1366 w1445 w1523 w1557 w1624 w1687 w1748 w1835 w1914 w1968 w2088]
      tunnel: [w264 w300 w338 w427 w520 w610 w700 w844 w935 w1029 w1074 w1122 w1159 w1199 w1239 w1276 w1307 w1365 w1444 w1522 w1556 w1623 w1686 w1747 w1834 w1913 w1967 w2060] -> w163
      tunnel: w162 -> [w264 w300 w338 w427 w520 w610 w700 w844 w935 w1029 w1074 w1122 w1159 w1199 w1239 w1276 w1307 w1365 w1444 w1522 w1556 w1623 w1686 w1747 w1834 w1913 w1978 w2060]
      tunnel: w146 -> [_ _ _ _ _ _ _ _ _ _ _ _ _ _ _ _ _ _ _ _ _ _ _ _ _ _ w1966 _]
      tunnel: w145 -> [w263 w299 w337 w426 w519 w609 w699 w843 w934 w1028 w1073 w1121 w1158 w1198 w1238 w1275 w1306 w1364 w1443 w1521 w1555 w1622 w1685 w1746 w1833 w1912 w1965 w2087]
      tunnel: [w263 w299 w337 w426 w519 w609 w699 w843 w934 w1028 w1073 w1121 w1158 w1198 w1238 w1275 w1306 w1364 w1443 w1521 w1555 w1622 w1685 w1746 w1833 w1912 w1964 w2087] -> w123
      tunnel: [w262 w298 w336 w425 w518 w608 w698 w842 w933 w1027 w1072 w1120 w1157 w1197 w1237 w1274 w1305 w1363 w1442 w1520 w1554 w1621 w1684 w1745 w1832 w1911 w1963 w2085] -> w122
      tunnel: w129 -> [w262 w298 w336 w425 w518 w608 w698 w842 w933 w1027 w1072 w1120 w1157 w1197 w1237 w1274 w1305 w1363 w1442 w1520 w1554 w1621 w1684 w1745 w1832 w1911 w1962 w2085]
      tunnel: [w261 w297 w335 w424 w517 w607 w697 w841 w932 w1026 w1071 w1119 w1156 w1196 w1236 w1273 w1304 w1362 w1441 w1519 w1553 w1620 w1683 w1744 w1831 w1910 w1960 w2063] -> w119
      tunnel: w121 -> [w261 w297 w335 w424 w517 w607 w697 w841 w932 w1026 w1071 w1119 w1156 w1196 w1236 w1273 w1304 w1362 w1441 w1519 w1553 w1620 w1683 w1744 w1831 w1910 w1959 w2063]
      tunnel: [w259 w295 w333 w374 w514 w605 w695 w791 w930 w1024 w1070 w1118 w1154 w1194 w1234 w1271 w1302 w1361 w1440 w1518 w1552 w1619 w1681 w1743 w1830 w1909 w1958 w2081] -> w79
      tunnel: w107 -> [w259 w295 w333 w420 w514 w605 w695 w837 w930 w1024 w1070 w1118 w1154 w1194 w1234 w1271 w1302 w1361 w1440 w1518 w1552 w1619 w1681 w1743 w1830 w1909 w1958 w2081]
      tunnel: [w260 w296 w334 w375 w515 w606 w696 w792 w931 w1025 w1069 w1117 w1155 w1195 w1235 w1272 w1303 w1360 w1439 w1517 w1551 w1618 w1682 w1742 w1829 w1908 w1957 w2082] -> w80
      tunnel: w106 -> [w260 w296 w334 w419 w515 w606 w696 w836 w931 w1025 w1069 w1117 w1155 w1195 w1235 w1272 w1303 w1360 w1439 w1517 w1551 w1618 w1682 w1742 w1829 w1908 w1957 w2082]
      tunnel: [w252 w288 w326 w379 w511 w603 w693 w796 w928 w1017 w1067 w1115 w1152 w1192 w1232 w1269 w1295 w1353 w1430 w1516 w1544 w1611 w1674 w1735 w1824 w1901 w1956 w2074] -> w84
      tunnel: w95 -> [w252 w288 w326 w409 w511 w603 w693 w826 w928 w1017 w1067 w1115 w1152 w1192 w1232 w1269 w1295 w1353 w1430 w1516 w1544 w1611 w1674 w1735 w1824 w1901 w1956 w2074]
      tunnel: [w251 w287 w325 w378 w512 w604 w694 w795 w929 w1016 w1068 w1116 w1153 w1193 w1233 w1270 w1294 w1352 w1429 w1515 w1543 w1610 w1673 w1734 w1823 w1900 w1955 w2073] -> w83
      tunnel: w94 -> [w251 w287 w325 w408 w512 w604 w694 w825 w929 w1016 w1068 w1116 w1153 w1193 w1233 w1270 w1294 w1352 w1429 w1515 w1543 w1610 w1673 w1734 w1823 w1900 w1955 w2073]
      tunnel: [w254 w290 w328 w384 w510 w601 w691 w801 w926 w1022 w1065 w1113 w1150 w1190 w1230 w1267 w1297 w1355 w1434 w1510 w1546 w1613 w1676 w1737 w1822 w1905 w1953 w2078] -> w77
      tunnel: w93 -> [w254 w290 w328 w405 w510 w601 w691 w822 w926 w1022 w1065 w1113 w1150 w1190 w1230 w1267 w1297 w1355 w1434 w1510 w1546 w1613 w1676 w1737 w1822 w1905 w1953 w2078]
      tunnel: [w253 w289 w327 w382 w513 w602 w692 w799 w927 w1023 w1066 w1114 w1151 w1191 w1231 w1268 w1296 w1354 w1433 w1509 w1545 w1612 w1675 w1736 w1821 w1904 w1954 w2077] -> w87
      tunnel: w92 -> [w253 w289 w327 w404 w513 w602 w692 w821 w927 w1023 w1066 w1114 w1151 w1191 w1231 w1268 w1296 w1354 w1433 w1509 w1545 w1612 w1675 w1736 w1821 w1904 w1954 w2077]
      tunnel: [w256 w292 w330 w373 w509 w599 w689 w790 w924 w1020 w1063 w1111 w1148 w1188 w1228 w1265 w1299 w1357 w1436 w1512 w1548 w1615 w1678 w1739 w1826 w1907 w1951 w2080] -> w78
      tunnel: w91 -> [w256 w292 w330 w401 w509 w599 w689 w818 w924 w1020 w1063 w1111 w1148 w1188 w1228 w1265 w1299 w1357 w1436 w1512 w1548 w1615 w1678 w1739 w1826 w1907 w1951 w2080]
      tunnel: [w255 w291 w329 w372 w508 w600 w690 w789 w925 w1021 w1064 w1112 w1149 w1189 w1229 w1266 w1298 w1356 w1435 w1511 w1547 w1614 w1677 w1738 w1825 w1906 w1952 w2079] -> w76
      tunnel: w90 -> [w255 w291 w329 w400 w508 w600 w690 w817 w925 w1021 w1064 w1112 w1149 w1189 w1229 w1266 w1298 w1356 w1435 w1511 w1547 w1614 w1677 w1738 w1825 w1906 w1952 w2079]
      tunnel: [w258 w294 w332 w377 w507 w597 w687 w794 w922 w1018 w1061 w1109 w1146 w1186 w1226 w1263 w1301 w1359 w1438 w1514 w1550 w1617 w1680 w1741 w1828 w1903 w1949 w2084] -> w82
      tunnel: w89 -> [w258 w294 w332 w397 w507 w597 w687 w814 w922 w1018 w1061 w1109 w1146 w1186 w1226 w1263 w1301 w1359 w1438 w1514 w1550 w1617 w1680 w1741 w1828 w1903 w1949 w2084]
      tunnel: [w257 w293 w331 w376 w506 w598 w688 w793 w923 w1019 w1062 w1110 w1147 w1187 w1227 w1264 w1300 w1358 w1437 w1513 w1549 w1616 w1679 w1740 w1827 w1902 w1950 w2083] -> w81
      tunnel: w88 -> [w257 w293 w331 w396 w506 w598 w688 w813 w923 w1019 w1062 w1110 w1147 w1187 w1227 w1264 w1300 w1358 w1437 w1513 w1549 w1616 w1679 w1740 w1827 w1902 w1950 w2083]
      tunnel: w70 -> [w250 w286 w324 w363 w505 w596 w686 w780 w921 w1015 w1060 w1108 w1145 w1185 w1225 w1262 w1293 w1351 w1428 w1508 w1542 w1609 w1672 w1733 w1820 w1899 w1948 _]
      tunnel: [w250 w286 w324 w363 w505 w596 w686 w780 w921 w1015 w1060 w1108 w1145 w1185 w1225 w1262 w1293 w1351 w1428 w1508 w1542 w1609 w1672 w1733 w1820 w1899 w1948 w2056] -> w71
      frame "wait" {
        n34 = Index Array(array=w285, index=0 ("Index")) -> (element=w283:string)
        n35 = Decimal String To Number(string=w283, default (0L)=u32 0) -> (number=w282:u32)  [unwired: 1 in, 1 out]
        n36 = Wait (ms)(milliseconds to wait=w282) -> ()  [unwired: 1 out]
      }
      frame "wait-min" {
        n37 = Index Array(array=w323, index=0 ("Index")) -> (element=w321:string)
        n38 = Decimal String To Number(string=w321, default (0L)=u32 0) -> (number=w309:u32)  [unwired: 1 in, 1 out]
        n39 = Multiply(x=w309, y=u32 60000) -> (x*y=w308:u32)
        n40 = Wait (ms)(milliseconds to wait=w308) -> ()  [unwired: 1 out]
      }
      frame "standby" {
        n41 = Index Array(array=w360, index=0 ("Index")) -> (element=w350:string)
        n42 = case shown="\"off\", Default" w350 {
          tunnel: [":PAGE:SCON:STAN 0" ":PAGE:SCON:STAN 1"] -> w345
          frame "off", Default {
          }
          frame "on" {
          }
        }
        n43 = VISA Write(VISA resource name=w349, write buffer=w345, error in (no error)=w348) -> (VISA resource name out=w347:refnum<visa-resource-name>, error out=w346:errorcluster)  [unwired: 1 out]
      }
      frame "transfer" {
        # "Adjusts graph colors."
        # "Adjusts graph colors."
        # "Is off"
        # "Is on"
        # "Ion will be the middle element of the array. The calculation of the index is done only once, since Is, Id, and Ig have the same dimensions."
        # "Ig off"
        # "Ig on"
        # "Is min"
        # "Is max"
        # "Ig min"
        # "Ig max"
        # "abs(Ig)"
        # "abs(Is)"
        # "Id min"
        # "Id max"
        # "Y1: Is\nY2: Id\nY3: Ig"
        # "abs(Id)"
        # "Adjusts graph colors."
        # "Adjusts graph colors."
        # "Id off"
        # "Id on"
        # "Adjusts graph colors."
        # "Time array"
        n44 = Delete From Array(array=w492, index=0 ("Index")) -> (deleted portion=w490:string, array with subset deleted=w489:string[])  [unwired: 1 in]
        n45 = Bundle By Name(cluster=w453, "Emergency Stop"=w501) -> (w454:T2)
        n46 = Number To Decimal String(number=w447) -> (decimal integer string=w446:string)  [unwired: 1 in]
        n47 = case shown="\"d\", Default" w490 {
          tunnel: [w503 w504] -> w488
          frame "s" {
            w503 = u16 0 items=["Single", "Double"] ("sweep mode")
          }
          frame "d", Default {
            w504 = u16 1 items=["Single", "Double"] ("sweep mode")
          }
        }
        n48 = Fract/Exp String To Number(string=w489) -> (number=w474:dbl[])  [unwired: 3 in, 1 out]
        n49 = Concatenate Strings(w499, w363, w446, w444, "_T_1_C_L.txt" ("Suffix (transfer)")) -> (w500:string)
        n50 = VISA Write(VISA resource name=w470, write buffer=":PAGE:CHAN:MODE SWE;" ("write buffer (\"\")"), error in (no error)=w469) -> (VISA resource name out=w467:refnum<visa-resource-name>, error out=w468:errorcluster)  [unwired: 1 out]
        n51 = String To Path(string=w500) -> (path=w498:path)
        n52 = Index Array(array=w474, index #1=0 ("Index")) -> (element #1=w487:dbl, element #2=w486:dbl, element #3=w485:dbl)  [unwired: 2 in]
        n53 = Delete From Array(array=w474, length=3 ("Length"), index=0 ("Index")) -> (array with subset deleted=w472:dbl[])  [unwired: 1 out]
        n54 = Build Array (concatenate)(w443, w439) -> (w389:i32[])
        n55 = Bundle By Name(cluster=w479, "Gate Start"=w487, "Gate Stop"=w486, "Gate Step (linear only)"=w485, "Gate Compliance"=w496, "Range mode"=w463, "Range"=w462) -> (w464:T6)
        n56 = control-ref of="Imax vs time"() -> (w418:refnum<vi>)
        n57 = control-ref of="Imin vs time"() -> (w417:refnum<vi>)
        n58 = control-ref of="Ion vs time"() -> (w386:refnum<vi>)
        n59 = control-ref of="Ioff vs time"() -> (w385:refnum<vi>)
        n60 = control-ref of="I vs Vg"() -> (w448:refnum<vi>)
        n61 = Index Array(array=w472, index #1=0 ("Index")) -> (element #1=w482:dbl, element #2=w481:dbl, element #3=w480:dbl)  [unwired: 2 in]
        n62 = call <vilib>:"compatOverwrite.vi"("overwrite (F)"=TRUE) -> ("overwrite?"=w452:T8)
        n63 = Bundle By Name(cluster=w478, "Drain Start"=w482, "Drain Stop"=w481, "Drain Step"=w480, "Drain Compliance"=w497, "Range mode"=w461, "Range"=w460) -> (w465:T7)
        n64 = call "4155C Transfer.vi"("VISA resource name in"=w467, "Gate"=w464, "Drain"=w465, "Timings"=w495, "error in (no error)"=w468, "SMU4"=w455, "sweep mode"=w488, "Panel Controls"=w454) -> ("VG"=w451:dbl[], "Outparams"=w459:T9, "VISA Resource Name out"=w494:refnum<visa-resource-name>, "IS"=w414:dbl[], "ID"=w416:dbl[], "IG"=w413:dbl[], "error out"=w440:errorcluster, "SMU4"=w456:dbl[])  [unwired: 12 in]
        n65 = Unbundle By Name(w459) -> ("V2 Step"=w458:dbl, "V2 Start"=w457:dbl, "Number of points"=w383:i32)
        n66 = Absolute Value(x=w414) -> (abs(x)=w399:dbl[])
        n67 = Absolute Value(x=w416) -> (abs(x)=w415:dbl[])
        n68 = Absolute Value(x=w413) -> (abs(x)=w402:dbl[])
        n69 = Array Size(array=w415) -> (size(s)=w423:i32)
        n70 = Divide(x=w423, y=2) -> (x/y=w366:dbl)
        n71 = Subtract(x=w366, y=1) -> (x-y=w365:dbl)
        n72 = Array Max & Min(array=w399) -> (max value=w406:dbl, min value=w407:dbl)  [unwired: 2 out]
        n73 = Array Max & Min(array=w415) -> (max value=w449:dbl, min value=w412:dbl)  [unwired: 2 out]
        n74 = Array Max & Min(array=w402) -> (max value=w411:dbl, min value=w410:dbl)  [unwired: 2 out]
        n75 = call "4155C Split array.vi"("Number of VAR2 steps"=w383, "Y2 data in"=w416, "X data in"=w451, "Y1 data in"=w414, "Y3 data in"=w413, "error in (no error)"=w440) -> ("Array of clusters"=w442:cluster{"Y data in":dbl[], "X data in":dbl[]}[], "error out"=w371:errorcluster)  [unwired: 1 in]
        n76 = Index Array(array=w399, index=w365) -> (element=w390:dbl)
        n77 = Index Array(array=w399, index=0) -> (element=w391:dbl)
        n78 = Index Array(array=w415, index=w365) -> (element=w392:dbl)
        n79 = Index Array(array=w415, index=0) -> (element=w393:dbl)
        n80 = Index Array(array=w402, index=w365) -> (element=w395:dbl)
        n81 = Index Array(array=w402, index=0) -> (element=w394:dbl)
        n82 = local write "Ig max"(w411) -> ()
        n83 = local write "Ig min"(w410) -> ()
        n84 = local write "Is max"(w406) -> ()
        n85 = local write "Is min"(w407) -> ()
        n86 = local write "Id max"(w449) -> ()
        n87 = local write "Id min"(w412) -> ()
        n88 = local write "I vs Vg"(w442) -> ()
        n89 = Build Array (concatenate)(w405, w406) -> (w384:dbl[])
        n90 = Build Array (concatenate)(w404, w407) -> (w382:dbl[])
        n91 = local write "Is off"(w391) -> ()
        n92 = local write "Is on"(w390) -> ()
        n93 = Build Array (concatenate)(w450, w449) -> (w381:dbl[])
        n94 = Build Array (concatenate)(w437, w412) -> (w380:dbl[])
        n95 = Build Array (concatenate)(w409, w411) -> (w379:dbl[])
        n96 = Build Array (concatenate)(w408, w410) -> (w378:dbl[])
        n97 = Build Array (concatenate)(w397, w390) -> (w377:dbl[])
        n98 = Build Array (concatenate)(w396, w391) -> (w376:dbl[])
        n99 = Build Array (concatenate)(w419, w392) -> (w375:dbl[])
        n100 = Build Array (concatenate)(w420, w393) -> (w374:dbl[])
        n101 = Build Array (concatenate)(w401, w395) -> (w373:dbl[])
        n102 = Build Array (concatenate)(w400, w394) -> (w372:dbl[])
        n103 = local write "Ig off"(w394) -> ()
        n104 = local write "Ig on"(w395) -> ()
        n105 = local write "Id off"(w393) -> ()
        n106 = local write "Id on"(w392) -> ()
        n107 = call "4155C Split array.vi"("Number of VAR2 steps"=w383, "Y2 data in"=w375, "X data in"=w389, "Y1 data in"=w377, "Y3 data in"=w373, "error in (no error)"=w371) -> ("Array of clusters"=w387:cluster{"Y data in":dbl[], "X data in":dbl[]}[], "error out"=w370:errorcluster)  [unwired: 1 in]
        n108 = call "4155C Split array.vi"("Number of VAR2 steps"=w383, "Y2 data in"=w374, "X data in"=w389, "Y1 data in"=w376, "Y3 data in"=w372, "error in (no error)"=w370) -> ("Array of clusters"=w388:cluster{"Y data in":dbl[], "X data in":dbl[]}[], "error out"=w369:errorcluster)  [unwired: 1 in]
        n109 = call "4155C Split array.vi"("Number of VAR2 steps"=w383, "Y2 data in"=w381, "X data in"=w389, "Y1 data in"=w384, "Y3 data in"=w379, "error in (no error)"=w369) -> ("Array of clusters"=w441:cluster{"Y data in":dbl[], "X data in":dbl[]}[], "error out"=w368:errorcluster)  [unwired: 1 in]
        n110 = call "4155C Split array.vi"("Number of VAR2 steps"=w383, "Y2 data in"=w380, "X data in"=w389, "Y1 data in"=w382, "Y3 data in"=w378, "error in (no error)"=w368) -> ("Array of clusters"=w438:cluster{"Y data in":dbl[], "X data in":dbl[]}[], "error out"=w367:errorcluster)  [unwired: 1 in]
        n111 = Open/Create/Replace File(file path (use dialog)=w498, error in=w367, operation (0:open)=w452) -> (refnum out=w435:refnum<file>, error out=w433:errorcluster)  [unwired: 3 in, 1 out]
        n112 = call "4155C Make Big 2d array.vi"("1D Var1"=w451, "1d IS"=w414, "1d ID"=w416, "1d IG"=w413, "1d SMU4"=w456, "SMU4"=w455, "VAR2 START"=w457, "Number of VAR2 steps"=w383, "VAR2 STEP"=w458, "VAR1 Name"="Vg", "Decimal places in header"=i8 1, "VAR2 Name"="Vd") -> ("Header array"=w436:string[], "Data array"=w434:dbl[][])  [unwired: 14 in]
        n113 = local write "Imax vs time"(w441) -> ()
        n114 = local write "Imin vs time"(w438) -> ()
        n115 = local write "Ion vs time"(w387) -> ()
        n116 = local write "Ioff vs time"(w388) -> ()
        n117 = call "4155C Config Chart Colours.vi"("Numeric"=w383, "XY Graph 2"=w418) -> ()  [unwired: 6 in]
        n118 = call "4155C Config Chart Colours.vi"("Numeric"=w383, "XY Graph 2"=w417) -> ()  [unwired: 6 in]
        n119 = call "4155C Config Chart Colours.vi"("Numeric"=w383, "XY Graph 2"=w386) -> ()  [unwired: 6 in]
        n120 = call "4155C Config Chart Colours.vi"("Numeric"=w383, "XY Graph 2"=w385) -> ()  [unwired: 6 in]
        n121 = call "4155C Config Chart Colours.vi"("Numeric"=w383, "XY Graph 2"=w448) -> ()  [unwired: 6 in]
        n122 = call "4155C Write array to file.vi"("Byte Stream File Refnum"=w435, "Header"=w436, "Data Array"=w434, "error in (no error)"=w433) -> ("dup refnum"=w432:refnum<file>, "error out"=w431:errorcluster)  [unwired: 1 in]
        n123 = Close File(refnum=w432, error in=w431) -> (error out=w493:errorcluster)  [unwired: 1 out]
      }
      frame "pulsedstressV" {
        w535 = 0
        n124 = Number To Decimal String(number=w526) -> (decimal integer string=w582:string)  [unwired: 1 in]
        n125 = Delete From Array(array=w516, index=0 ("Index")) -> (deleted portion=w573:string, array with subset deleted=w572:string[])  [unwired: 1 in]
        n126 = Bundle By Name(cluster=w552, "Emergency Stop"=w585) -> (w554:T2)
        n127 = VISA Write(VISA resource name=w566, write buffer=":PAGE:CHAN:MODE SWE;" ("write buffer (\"\")"), error in (no error)=w565) -> (VISA resource name out=w563:refnum<visa-resource-name>, error out=w564:errorcluster)  [unwired: 1 out]
        n128 = Concatenate Strings(w581, "-pulsedstressV-" ("Substring"), w582, w525, ".txt" ("Substring")) -> (w584:string)
        n129 = case shown="\"d\", Default" w573 {
          tunnel: [w594 w595] -> w571
          frame "s" {
            w594 = u16 0 items=["Single", "Double"] ("sweep mode")
          }
          frame "d", Default {
            w595 = u16 1 items=["Single", "Double"] ("sweep mode")
          }
        }
        n130 = Fract/Exp String To Number(string=w572) -> (number=w567:dbl[])  [unwired: 3 in, 1 out]
        n131 = String To Path(string=w584) -> (path=w580:path)
        n132 = Index Array(array=w567, index #1=0 ("Index")) -> (element #1=w544:dbl, element #2=w543:dbl, element #3=w540:dbl, element #4=w539:dbl, element #5=w538:dbl, element #6=w542:dbl)  [unwired: 5 in]
        n133 = Bundle By Name(cluster=w541, "Pulse period"=w539, "Base voltage"=w540, "Pulse width"=w538) -> (w537:T5)
        n134 = Unbundle By Name(w537) -> ("Pulse period"=w545:dbl)
        n135 = Bundle By Name(cluster=w569, "Gate Start"=w543, "Gate Stop"=w544, "Gate Step (linear only)"=0, "Gate Compliance"=w578, "Range mode"=w559, "Range"=w558) -> (w560:T6)
        n136 = call <vilib>:"compatOverwrite.vi"("overwrite (F)"=TRUE) -> ("overwrite?"=w530:T8)
        n137 = Bundle By Name(cluster=w568, "Drain Start"=w542, "Drain Stop"=w535, "Drain Step"=w535, "Drain Compliance"=w579, "Range mode"=w557, "Range"=w556) -> (w561:T7)
        n138 = call "4155C PulsedStressV.vi"("VISA resource name in"=w563, "sweep mode"=w571, "Panel Controls"=w554, "Gate"=w560, "Drain"=w561, "Timings"=w537, "error in (no error)"=w564, "SMU4"=w553) -> ("VISA Resource Name out"=w576:refnum<visa-resource-name>, "ID"=w533:dbl[], "IG"=w531:dbl[], "Outparams"=w555:T9, "error out"=w577:errorcluster)  [unwired: 3 in]
        n139 = Unbundle By Name(w555) -> ("Number of points"=w532:i32)  [unwired: 2 out]
        n140 = for {
          N: w532 -> [_]
          tunnel: [w591] -> w534 mode=indexing
          tunnel: w545 -> [w593]
          i -> [w592]
          n141 = Multiply(x=w593, y=w592) -> (x*y=w591:dbl)
        }
        n142 = Insert Into Array(array=dbl[][] [] ("Input Array"), new element=w534) -> (w546:dbl[][])  [unwired: 2 in]
        n143 = Insert Into Array(array=w546, new element=w533) -> (w551:dbl[][])  [unwired: 2 in]
        n144 = Insert Into Array(array=w551, new element=w531) -> (w550:dbl[][])  [unwired: 2 in]
        n145 = Transpose 2D Array(2D array=w550) -> (transposed array=w549:dbl[][])
        n146 = Open/Create/Replace File(file path (use dialog)=w580, error in=w577, operation (0:open)=w530) -> (refnum out=w588:refnum<file>, error out=w589:errorcluster)  [unwired: 3 in, 1 out]
        n147 = call "4155C Write array to file.vi"("Byte Stream File Refnum"=w588, "Header"=string[] ["Time /s", "Id /A", "Ig /A"], "Data Array"=w549, "error in (no error)"=w589) -> ("dup refnum"=w586:refnum<file>, "error out"=w587:errorcluster)  [unwired: 1 in]
        n148 = Close File(refnum=w586, error in=w587) -> (error out=w575:errorcluster)  [unwired: 1 out]
      }
      frame "transfer-fpp" {
        n149 = Number To Decimal String(number=w617) -> (decimal integer string=w671:string)  [unwired: 1 in]
        n150 = Bundle By Name(cluster=w647, "Emergency Stop"=w675) -> (w683:T1)
        n151 = Delete From Array(array=w662, index=0 ("Index")) -> (deleted portion=w660:string, array with subset deleted=w659:string[])  [unwired: 1 in]
        n152 = Concatenate Strings(w670, "-transferfpp-" ("Substring"), w671, w615, ".txt" ("Substring")) -> (w673:string)
        n153 = VISA Write(VISA resource name=w639, write buffer=":PAGE:CHAN:MODE SWE;" ("write buffer (\"\")"), error in (no error)=w638) -> (VISA resource name out=w636:refnum<visa-resource-name>, error out=w637:errorcluster)  [unwired: 1 out]
        n154 = case shown="\"d\", Default" w660 {
          tunnel: [w684 w685] -> w658
          frame "s" {
            w684 = u16 0 items=["Single", "Double"] ("sweep mode")
          }
          frame "d", Default {
            w685 = u16 1 items=["Single", "Double"] ("sweep mode")
          }
        }
        n155 = Fract/Exp String To Number(string=w659) -> (number=w643:dbl[])  [unwired: 3 in, 1 out]
        n156 = String To Path(string=w673) -> (path=w669:path)
        n157 = Index Array(array=w643, index #1=0 ("Index")) -> (element #1=w657:dbl, element #2=w656:dbl, element #3=w655:dbl)  [unwired: 2 in]
        n158 = Delete From Array(array=w643, length=3 ("Length"), index=0 ("Index")) -> (array with subset deleted=w641:dbl[])  [unwired: 1 out]
        n159 = Bundle By Name(cluster=w649, "Gate Start"=w657, "Gate Stop"=w656, "Gate Step (linear only)"=w655, "Gate Compliance"=w667, "Range mode"=w632, "Range"=w631) -> (w633:T6)
        n160 = Index Array(array=w641, index #1=0 ("Index")) -> (element #1=w652:dbl, element #2=w651:dbl, element #3=w650:dbl)  [unwired: 2 in]
        n161 = call <vilib>:"compatOverwrite.vi"("overwrite (F)"=TRUE) -> ("overwrite?"=w620:T8)
        n162 = Bundle By Name(cluster=w648, "Drain Start"=w652, "Drain Stop"=w651, "Drain Step"=w650, "Drain Compliance"=w668, "Range mode"=w630, "Range"=w629) -> (w634:T7)
        n163 = call "4155C Transfer-FPP.vi"("VISA resource name in"=w636, "Gate"=w633, "Drain"=w634, "Timings"=w666, "error in (no error)"=w637, "sweep mode"=w658, "Panel Controls"=w683) -> ("VG"=w674:dbl[], "Outparams"=w628:T9, "VISA Resource Name out"=w664:refnum<visa-resource-name>, "Vprobe2"=w624:dbl[], "ID"=w623:dbl[], "IG"=w622:dbl[], "Vprobe1"=w621:dbl[], "error out"=w665:errorcluster)  [unwired: 13 in]
        n164 = Unbundle By Name(w628) -> ("V2 Step"=w627:dbl, "V2 Start"=w626:dbl, "Number of points"=w625:i32)
        n165 = Open/Create/Replace File(file path (use dialog)=w669, error in=w665, operation (0:open)=w620) -> (refnum out=w680:refnum<file>, error out=w681:errorcluster)  [unwired: 3 in, 1 out]
        n166 = call "4155C Make Big 2d array FPP.vi"("1D Var1"=w674, "1d ID"=w623, "1d Vp2"=w624, "1d IG"=w622, "1d Vp1"=w621, "VAR2 START"=w626, "Number of VAR2 steps"=w625, "VAR2 STEP"=w627, "VAR1 Name"="Vg", "Decimal places in header"=i8 1, "VAR2 Name"="Vd") -> ("Header array"=w676:string[], "Data array"=w677:dbl[][])  [unwired: 15 in]
        n167 = call "4155C Write array to file.vi"("Byte Stream File Refnum"=w680, "Header"=w676, "Data Array"=w677, "error in (no error)"=w681) -> ("dup refnum"=w678:refnum<file>, "error out"=w679:errorcluster)  [unwired: 1 in]
        n168 = Close File(refnum=w678, error in=w679) -> (error out=w663:errorcluster)  [unwired: 1 out]
      }
      frame "output" {
        n169 = Number To Decimal String(number=w715) -> (decimal integer string=w764:string)  [unwired: 1 in]
        n170 = Bundle By Name(cluster=w741, "Emergency Stop"=w766) -> (w776:T1)
        n171 = Delete From Array(array=w756, index=0 ("Index")) -> (deleted portion=w754:string, array with subset deleted=w753:string[])  [unwired: 1 in]
        n172 = Concatenate Strings(w763, w686, w764, w714, "_O.txt" ("Suffix (output)")) -> (w765:string)
        n173 = VISA Write(VISA resource name=w732, write buffer=":PAGE:CHAN:MODE SWE;" ("write buffer (\"\")"), error in (no error)=w729) -> (VISA resource name out=w731:refnum<visa-resource-name>, error out=w730:errorcluster)  [unwired: 1 out]
        n174 = case shown="\"d\", Default" w754 {
          tunnel: [w777 w778] -> w752
          frame "s" {
            w777 = u16 0 items=["Single", "Double"] ("sweep mode")
          }
          frame "d", Default {
            w778 = u16 1 items=["Single", "Double"] ("sweep mode")
          }
        }
        n175 = Fract/Exp String To Number(string=w753) -> (number=w735:dbl[])  [unwired: 3 in, 1 out]
        n176 = String To Path(string=w765) -> (path=w762:path)
        n177 = Index Array(array=w735, index #1=0 ("Index")) -> (element #1=w751:dbl, element #2=w750:dbl, element #3=w749:dbl)  [unwired: 2 in]
        n178 = Delete From Array(array=w735, length=3 ("Length"), index=0 ("Index")) -> (array with subset deleted=w734:dbl[])  [unwired: 1 out]
        n179 = control-ref of="I vs Vd"() -> (w705:refnum<vi>)
        n180 = Bundle By Name(cluster=w743, "Gate Start"=w751, "Gate Stop"=w750, "Gate Step (linear only)"=w749, "Gate Compliance"=w760, "Range mode"=w727, "Range"=w726) -> (w775:T6)
        n181 = Index Array(array=w734, index #1=0 ("Index")) -> (element #1=w746:dbl, element #2=w745:dbl, element #3=w744:dbl)  [unwired: 2 in]
        n182 = call <vilib>:"compatOverwrite.vi"("overwrite (F)"=TRUE) -> ("overwrite?"=w719:T8)
        n183 = Bundle By Name(cluster=w742, "Drain Start"=w746, "Drain Stop"=w745, "Drain Step"=w744, "Drain Compliance"=w761, "Range mode"=w725, "Range"=w728) -> (w774:T7)
        n184 = call "4155C Output.vi"("VISA resource name in"=w731, "Gate"=w775, "Drain"=w774, "Timings"=w759, "error in (no error)"=w730, "SMU4"=w721, "sweep mode"=w752, "Panel controls"=w776) -> ("VD"=w712:dbl[], "Outparams"=w723:T9, "VISA Resource Name out"=w758:refnum<visa-resource-name>, "IS"=w711:dbl[], "ID"=w710:dbl[], "IG"=w709:dbl[], "error out"=w707:errorcluster, "SMU4"=w720:dbl[])  [unwired: 12 in]
        n185 = Unbundle By Name(w723) -> ("V2 Step"=w724:dbl, "V2 Start"=w722:dbl, "Number of points"=w704:i32)
        n186 = call "4155C Split array.vi"("Number of VAR2 steps"=w704, "Y2 data in"=w710, "X data in"=w712, "Y1 data in"=w711, "Y3 data in"=w709, "error in (no error)"=w707) -> ("Array of clusters"=w708:cluster{"Y data in":dbl[], "X data in":dbl[]}[], "error out"=w706:errorcluster)  [unwired: 1 in]
        n187 = local write "I vs Vd"(w708) -> ()
        n188 = call "4155C Config Chart Colours.vi"("Numeric"=w704, "XY Graph 2"=w705) -> ()  [unwired: 6 in]
        n189 = Open/Create/Replace File(file path (use dialog)=w762, error in=w706, operation (0:open)=w719) -> (refnum out=w771:refnum<file>, error out=w772:errorcluster)  [unwired: 3 in, 1 out]
        n190 = call "4155C Make Big 2d array.vi"("1D Var1"=w712, "1d IS"=w711, "1d ID"=w710, "1d IG"=w709, "1d SMU4"=w720, "SMU4"=w721, "VAR2 START"=w722, "Number of VAR2 steps"=w704, "VAR2 STEP"=w724, "VAR1 Name"="Vd", "Decimal places in header"=i8 1, "VAR2 Name"="Vg") -> ("Header array"=w767:string[], "Data array"=w768:dbl[][])  [unwired: 14 in]
        n191 = call "4155C Write array to file.vi"("Byte Stream File Refnum"=w771, "Header"=w767, "Data Array"=w768, "error in (no error)"=w772) -> ("dup refnum"=w769:refnum<file>, "error out"=w770:errorcluster)  [unwired: 1 in]
        n192 = Close File(refnum=w769, error in=w770) -> (error out=w757:errorcluster)  [unwired: 1 out]
      }
      frame "output2" {
        # "Adjusts graph colors."
        # "Adjusts graph colors."
        # "Is off"
        # "Is on"
        # "Ion will be the middle element of the array. The calculation of the index is done only once, since Is, Id, and Ig have the same dimensions."
        # "Ig off"
        # "Ig on"
        # "Is min"
        # "Is max"
        # "Ig min"
        # "Ig max"
        # "abs(Ig)"
        # "abs(Is)"
        # "Id min"
        # "Id max"
        # "Y1: Is\nY2: Id\nY3: Ig"
        # "abs(Id)"
        # "Adjusts graph colors."
        # "Adjusts graph colors."
        # "Id off"
        # "Id on"
        # "Adjusts graph colors."
        # "Time array"
        n193 = Delete From Array(array=w908, index=0 ("Index")) -> (deleted portion=w906:string, array with subset deleted=w905:string[])  [unwired: 1 in]
        n194 = Bundle By Name(cluster=w779, "Emergency Stop"=w917) -> (w870:T1)
        n195 = Number To Decimal String(number=w864) -> (decimal integer string=w863:string)  [unwired: 1 in]
        n196 = case shown="\"d\", Default" w906 {
          tunnel: [w919 w920] -> w904
          frame "s" {
            w919 = u16 0 items=["Single", "Double"] ("sweep mode")
          }
          frame "d", Default {
            w920 = u16 1 items=["Single", "Double"] ("sweep mode")
          }
        }
        n197 = Fract/Exp String To Number(string=w905) -> (number=w890:dbl[])  [unwired: 3 in, 1 out]
        n198 = Concatenate Strings(w915, w780, w863, w861, "_O_1_C_L.txt" ("Suffix (transfer)")) -> (w916:string)
        n199 = VISA Write(VISA resource name=w886, write buffer=":PAGE:CHAN:MODE SWE;" ("write buffer (\"\")"), error in (no error)=w885) -> (VISA resource name out=w883:refnum<visa-resource-name>, error out=w884:errorcluster)  [unwired: 1 out]
        n200 = String To Path(string=w916) -> (path=w914:path)
        n201 = Index Array(array=w890, index #1=0 ("Index")) -> (element #1=w903:dbl, element #2=w902:dbl, element #3=w901:dbl)  [unwired: 2 in]
        n202 = Delete From Array(array=w890, length=3 ("Length"), index=0 ("Index")) -> (array with subset deleted=w888:dbl[])  [unwired: 1 out]
        n203 = Build Array (concatenate)(w860, w856) -> (w806:i32[])
        n204 = Bundle By Name(cluster=w895, "Gate Start"=w903, "Gate Stop"=w902, "Gate Step (linear only)"=w901, "Gate Compliance"=w912, "Range mode"=w879, "Range"=w878) -> (w880:T6)
        n205 = control-ref of="Imax vs time"() -> (w835:refnum<vi>)
        n206 = control-ref of="Imin vs time"() -> (w834:refnum<vi>)
        n207 = control-ref of="Ion vs time"() -> (w803:refnum<vi>)
        n208 = control-ref of="Ioff vs time"() -> (w802:refnum<vi>)
        n209 = control-ref of="I vs Vg"() -> (w865:refnum<vi>)
        n210 = Index Array(array=w888, index #1=0 ("Index")) -> (element #1=w898:dbl, element #2=w897:dbl, element #3=w896:dbl)  [unwired: 2 in]
        n211 = call <vilib>:"compatOverwrite.vi"("overwrite (F)"=TRUE) -> ("overwrite?"=w869:T8)
        n212 = Bundle By Name(cluster=w894, "Drain Start"=w898, "Drain Stop"=w897, "Drain Step"=w896, "Drain Compliance"=w913, "Range mode"=w877, "Range"=w876) -> (w881:T7)
        n213 = call "4155C Output.vi"("VISA resource name in"=w883, "Gate"=w880, "Drain"=w881, "Timings"=w911, "error in (no error)"=w884, "SMU4"=w871, "sweep mode"=w904, "Panel controls"=w870) -> ("VD"=w868:dbl[], "Outparams"=w875:T9, "VISA Resource Name out"=w910:refnum<visa-resource-name>, "IS"=w831:dbl[], "ID"=w833:dbl[], "IG"=w830:dbl[], "error out"=w857:errorcluster, "SMU4"=w872:dbl[])  [unwired: 12 in]
        n214 = Unbundle By Name(w875) -> ("V2 Step"=w874:dbl, "V2 Start"=w873:dbl, "Number of points"=w800:i32)
        n215 = Absolute Value(x=w831) -> (abs(x)=w816:dbl[])
        n216 = Absolute Value(x=w833) -> (abs(x)=w832:dbl[])
        n217 = Absolute Value(x=w830) -> (abs(x)=w819:dbl[])
        n218 = Array Size(array=w832) -> (size(s)=w840:i32)
        n219 = Divide(x=w840, y=2) -> (x/y=w783:dbl)
        n220 = Subtract(x=w783, y=1) -> (x-y=w782:dbl)
        n221 = Array Max & Min(array=w816) -> (max value=w823:dbl, min value=w824:dbl)  [unwired: 2 out]
        n222 = Array Max & Min(array=w832) -> (max value=w866:dbl, min value=w829:dbl)  [unwired: 2 out]
        n223 = Array Max & Min(array=w819) -> (max value=w828:dbl, min value=w827:dbl)  [unwired: 2 out]
        n224 = call "4155C Split array.vi"("Number of VAR2 steps"=w800, "Y2 data in"=w833, "X data in"=w868, "Y1 data in"=w831, "Y3 data in"=w830, "error in (no error)"=w857) -> ("Array of clusters"=w859:cluster{"Y data in":dbl[], "X data in":dbl[]}[], "error out"=w788:errorcluster)  [unwired: 1 in]
        n225 = Index Array(array=w816, index=w782) -> (element=w807:dbl)
        n226 = Index Array(array=w816, index=0) -> (element=w808:dbl)
        n227 = Index Array(array=w832, index=w782) -> (element=w809:dbl)
        n228 = Index Array(array=w832, index=0) -> (element=w810:dbl)
        n229 = Index Array(array=w819, index=w782) -> (element=w812:dbl)
        n230 = Index Array(array=w819, index=0) -> (element=w811:dbl)
        n231 = local write "Ig max"(w828) -> ()
        n232 = local write "Ig min"(w827) -> ()
        n233 = local write "Is max"(w823) -> ()
        n234 = local write "Is min"(w824) -> ()
        n235 = local write "Id max"(w866) -> ()
        n236 = local write "Id min"(w829) -> ()
        n237 = local write "I vs Vd"(w859) -> ()
        n238 = Build Array (concatenate)(w822, w823) -> (w801:dbl[])
        n239 = Build Array (concatenate)(w821, w824) -> (w799:dbl[])
        n240 = local write "Is off"(w808) -> ()
        n241 = local write "Is on"(w807) -> ()
        n242 = Build Array (concatenate)(w867, w866) -> (w798:dbl[])
        n243 = Build Array (concatenate)(w854, w829) -> (w797:dbl[])
        n244 = Build Array (concatenate)(w826, w828) -> (w796:dbl[])
        n245 = Build Array (concatenate)(w825, w827) -> (w795:dbl[])
        n246 = Build Array (concatenate)(w814, w807) -> (w794:dbl[])
        n247 = Build Array (concatenate)(w813, w808) -> (w793:dbl[])
        n248 = Build Array (concatenate)(w836, w809) -> (w792:dbl[])
        n249 = Build Array (concatenate)(w837, w810) -> (w791:dbl[])
        n250 = Build Array (concatenate)(w818, w812) -> (w790:dbl[])
        n251 = Build Array (concatenate)(w817, w811) -> (w789:dbl[])
        n252 = local write "Ig off"(w811) -> ()
        n253 = local write "Ig on"(w812) -> ()
        n254 = local write "Id off"(w810) -> ()
        n255 = local write "Id on"(w809) -> ()
        n256 = call "4155C Split array.vi"("Number of VAR2 steps"=w800, "Y2 data in"=w792, "X data in"=w806, "Y1 data in"=w794, "Y3 data in"=w790, "error in (no error)"=w788) -> ("Array of clusters"=w804:cluster{"Y data in":dbl[], "X data in":dbl[]}[], "error out"=w787:errorcluster)  [unwired: 1 in]
        n257 = call "4155C Split array.vi"("Number of VAR2 steps"=w800, "Y2 data in"=w791, "X data in"=w806, "Y1 data in"=w793, "Y3 data in"=w789, "error in (no error)"=w787) -> ("Array of clusters"=w805:cluster{"Y data in":dbl[], "X data in":dbl[]}[], "error out"=w786:errorcluster)  [unwired: 1 in]
        n258 = call "4155C Split array.vi"("Number of VAR2 steps"=w800, "Y2 data in"=w798, "X data in"=w806, "Y1 data in"=w801, "Y3 data in"=w796, "error in (no error)"=w786) -> ("Array of clusters"=w858:cluster{"Y data in":dbl[], "X data in":dbl[]}[], "error out"=w785:errorcluster)  [unwired: 1 in]
        n259 = call "4155C Split array.vi"("Number of VAR2 steps"=w800, "Y2 data in"=w797, "X data in"=w806, "Y1 data in"=w799, "Y3 data in"=w795, "error in (no error)"=w785) -> ("Array of clusters"=w855:cluster{"Y data in":dbl[], "X data in":dbl[]}[], "error out"=w784:errorcluster)  [unwired: 1 in]
        n260 = Open/Create/Replace File(file path (use dialog)=w914, error in=w784, operation (0:open)=w869) -> (refnum out=w852:refnum<file>, error out=w850:errorcluster)  [unwired: 3 in, 1 out]
        n261 = call "4155C Make Big 2d array.vi"("1D Var1"=w868, "1d IS"=w831, "1d ID"=w833, "1d IG"=w830, "1d SMU4"=w872, "SMU4"=w871, "VAR2 START"=w873, "Number of VAR2 steps"=w800, "VAR2 STEP"=w874, "VAR1 Name"="Vd", "Decimal places in header"=i8 1, "VAR2 Name"="Vg") -> ("Header array"=w853:string[], "Data array"=w851:dbl[][])  [unwired: 14 in]
        n262 = local write "Imax vs time"(w858) -> ()
        n263 = local write "Imin vs time"(w855) -> ()
        n264 = local write "Ion vs time"(w804) -> ()
        n265 = local write "Ioff vs time"(w805) -> ()
        n266 = call "4155C Config Chart Colours.vi"("Numeric"=w800, "XY Graph 2"=w835) -> ()  [unwired: 6 in]
        n267 = call "4155C Config Chart Colours.vi"("Numeric"=w800, "XY Graph 2"=w834) -> ()  [unwired: 6 in]
        n268 = call "4155C Config Chart Colours.vi"("Numeric"=w800, "XY Graph 2"=w803) -> ()  [unwired: 6 in]
        n269 = call "4155C Config Chart Colours.vi"("Numeric"=w800, "XY Graph 2"=w802) -> ()  [unwired: 6 in]
        n270 = call "4155C Config Chart Colours.vi"("Numeric"=w800, "XY Graph 2"=w865) -> ()  [unwired: 6 in]
        n271 = call "4155C Write array to file.vi"("Byte Stream File Refnum"=w852, "Header"=w853, "Data Array"=w851, "error in (no error)"=w850) -> ("dup refnum"=w849:refnum<file>, "error out"=w848:errorcluster)  [unwired: 1 in]
        n272 = Close File(refnum=w849, error in=w848) -> (error out=w909:errorcluster)  [unwired: 1 out]
      }
      frame "output-fpp" {
        n273 = Number To Decimal String(number=w941) -> (decimal integer string=w995:string)  [unwired: 1 in]
        n274 = Bundle By Name(cluster=w971, "Emergency Stop"=w998) -> (w1008:T1)
        n275 = Delete From Array(array=w986, index=0 ("Index")) -> (deleted portion=w984:string, array with subset deleted=w983:string[])  [unwired: 1 in]
        n276 = VISA Write(VISA resource name=w962, write buffer=":PAGE:CHAN:MODE SWE;" ("write buffer (\"\")"), error in (no error)=w959) -> (VISA resource name out=w961:refnum<visa-resource-name>, error out=w960:errorcluster)  [unwired: 1 out]
        n277 = Concatenate Strings(w994, "-outputfpp-" ("Substring"), w995, w940, ".txt" ("Substring")) -> (w997:string)
        n278 = case shown="\"d\", Default" w984 {
          tunnel: [w1009 w1010] -> w982
          frame "s" {
            w1009 = u16 0 items=["Single", "Double"] ("sweep mode")
          }
          frame "d", Default {
            w1010 = u16 1 items=["Single", "Double"] ("sweep mode")
          }
        }
        n279 = Fract/Exp String To Number(string=w983) -> (number=w965:dbl[])  [unwired: 3 in, 1 out]
        n280 = String To Path(string=w997) -> (path=w993:path)
        n281 = Index Array(array=w965, index #1=0 ("Index")) -> (element #1=w981:dbl, element #2=w980:dbl, element #3=w979:dbl)  [unwired: 2 in]
        n282 = Delete From Array(array=w965, length=3 ("Length"), index=0 ("Index")) -> (array with subset deleted=w964:dbl[])  [unwired: 1 out]
        n283 = Bundle By Name(cluster=w973, "Gate Start"=w981, "Gate Stop"=w980, "Gate Step (linear only)"=w979, "Gate Compliance"=w991, "Range mode"=w957, "Range"=w956) -> (w1007:T6)
        n284 = Index Array(array=w964, index #1=0 ("Index")) -> (element #1=w976:dbl, element #2=w975:dbl, element #3=w974:dbl)  [unwired: 2 in]
        n285 = call <vilib>:"compatOverwrite.vi"("overwrite (F)"=TRUE) -> ("overwrite?"=w945:T8)
        n286 = Bundle By Name(cluster=w972, "Drain Start"=w976, "Drain Stop"=w975, "Drain Step"=w974, "Drain Compliance"=w992, "Range mode"=w955, "Range"=w958) -> (w1006:T7)
        n287 = call "4155C Output-FPP.vi"("VISA resource name in"=w961, "Gate"=w1007, "Drain"=w1006, "Timings"=w990, "error in (no error)"=w960, "sweep mode"=w982, "Panel controls"=w1008) -> ("VD"=w950:dbl[], "Outparams"=w953:T9, "VISA Resource Name out"=w988:refnum<visa-resource-name>, "Vprobe2"=w949:dbl[], "ID"=w948:dbl[], "IG"=w947:dbl[], "Vprobe1"=w946:dbl[], "error out"=w989:errorcluster)  [unwired: 13 in]
        n288 = Unbundle By Name(w953) -> ("V2 Step"=w954:dbl, "V2 Start"=w952:dbl, "Number of points"=w951:i32)
        n289 = Open/Create/Replace File(file path (use dialog)=w993, error in=w989, operation (0:open)=w945) -> (refnum out=w1003:refnum<file>, error out=w1004:errorcluster)  [unwired: 3 in, 1 out]
        n290 = call "4155C Make Big 2d array FPP.vi"("1D Var1"=w950, "1d ID"=w948, "1d Vp2"=w949, "1d IG"=w947, "1d Vp1"=w946, "VAR2 START"=w952, "Number of VAR2 steps"=w951, "VAR2 STEP"=w954, "VAR1 Name"="Vd", "Decimal places in header"=i8 1, "VAR2 Name"="Vg") -> ("Header array"=w999:string[], "Data array"=w1000:dbl[][])  [unwired: 15 in]
        n291 = call "4155C Write array to file.vi"("Byte Stream File Refnum"=w1003, "Header"=w999, "Data Array"=w1000, "error in (no error)"=w1004) -> ("dup refnum"=w1001:refnum<file>, "error out"=w1002:errorcluster)  [unwired: 1 in]
        n292 = Close File(refnum=w1001, error in=w1002) -> (error out=w987:errorcluster)  [unwired: 1 out]
      }
      frame "itime" {
        n293 = Delete From Array(array=w1013, index=1) -> (deleted portion=w1012:string)  [unwired: 1 in, 1 out]
        n294 = Delete From Array(array=w1013, index=0 ("Index")) -> (deleted portion=w1047:string)  [unwired: 1 in, 1 out]
        n295 = Fract/Exp String To Number(string=w1012) -> (number=w1011:dbl)  [unwired: 3 in, 1 out]
        n296 = case shown="\"l\"" w1047 {
          tunnel: w1046 -> [w1052 w1054 w1058]
          tunnel: [w1051 w1053 w1057] -> w1039
          tunnel: w1011 -> [w1049 _ w1056]
          frame "s" {
            w1050 = u32 0 items=["short  ", "medium  ", "long  "] ("integration time 2")
            n297 = Bundle By Name(cluster=w1052, "integration time"=w1050, "Short/Long integration time"=w1049) -> (w1051:T5)
          }
          frame "m", Default {
            w1055 = u32 1 items=["short  ", "medium  ", "long  "] ("integration time 2")
            n298 = Bundle By Name(cluster=w1054, "integration time"=w1055) -> (w1053:T5)
          }
          frame "l" {
            w1059 = u32 2 items=["short  ", "medium  ", "long  "] ("integration time 2")
            n299 = Bundle By Name(cluster=w1058, "integration time"=w1059, "Short/Long integration time"=w1056) -> (w1057:T5)
          }
        }
      }
      frame "pulsed" {
        n300 = Delete From Array(array=w1093, index=0 ("Index")) -> (deleted portion=w1094:string, array with subset deleted=w1081:string[])  [unwired: 1 in]
        n301 = case shown="\"on\", Default" w1094 {
          tunnel: w1092 -> [w1104 w1107]
          tunnel: [w1103 w1106] -> w1085
          tunnel: w1081 -> [w1101 _]
          frame "on", Default {
            w1102 = u16 1 items=["Continuous", "Pulsed"] ("sweep method")
            n302 = Fract/Exp String To Number(string=w1101) -> (number=w1099:dbl[])  [unwired: 3 in, 1 out]
            n303 = Index Array(array=w1099, index #1=0 ("Index")) -> (element #1=w1098:dbl, element #2=w1097:dbl, element #3=w1096:dbl)  [unwired: 2 in]
            n304 = Bundle By Name(cluster=w1104, "sweep method"=w1102, "Pulse period"=w1098, "Base voltage"=w1097, "Pulse width"=w1096) -> (w1103:T5)
          }
          frame "off" {
            w1105 = u16 0 items=["Continuous", "Pulsed"] ("sweep method")
            n305 = Bundle By Name(cluster=w1107, "sweep method"=w1105) -> (w1106:T5)
          }
        }
      }
      frame "gaterangemode" {
        n306 = Delete From Array(array=w1139, index=0 ("Index")) -> (deleted portion=w1140:string)  [unwired: 1 in, 1 out]
        n307 = case shown="\"f\"" w1140 {
          tunnel: [w1142 w1143 w1144] -> w1129
          frame "a", Default {
            w1142 = u16 0 items=["Auto", "Limited", "Fixed"] ("Gate Range\nmode 2")
          }
          frame "f" {
            w1143 = u16 2 items=["Auto", "Limited", "Fixed"] ("Gate Range\nmode 2")
          }
          frame "l" {
            w1144 = u16 1 items=["Auto", "Limited", "Fixed"] ("Gate Range\nmode 2")
          }
        }
      }
      frame "gaterange" {
        (unwired) u8 11 items=["10fA  ", "100fA  ", "1nA  ", "10nA", "100nA", "1uA", "10uA", "100uA", "1mA", "10mA", "100mA", "1A"] ("Gate Range 2")
        n308 = Delete From Array(array=w1183, index=0 ("Index")) -> (deleted portion=w1173:string)  [unwired: 1 in, 1 out]
        n309 = Scan Value(string=w1173, format string="") -> (value=w1171:dbl)  [unwired: 1 in, 1 out]
        n310 = Logarithm Base 10(1:w1171) -> (0:w1170:dbl)
        n311 = Round To Nearest(number=w1170) -> (nearest integer value=w1169:dbl)
        n312 = Add(x=w1169, y=11.0) -> (x+y=w1167:dbl)
        n313 = To Unsigned Byte Integer(number=w1167) -> (unsigned 8bit integer=w1166:u8)
      }
      frame "drainrange" {
        (unwired) u8 11 items=["10fA  ", "100fA  ", "1nA  ", "10nA", "100nA", "1uA", "10uA", "100uA", "1mA", "10mA", "100mA", "1A"] ("Gate Range 2")
        n314 = Delete From Array(array=w1223, index=0 ("Index")) -> (deleted portion=w1214:string)  [unwired: 1 in, 1 out]
        n315 = Scan Value(string=w1214, format string="") -> (value=w1212:dbl)  [unwired: 1 in, 1 out]
        n316 = Logarithm Base 10(1:w1212) -> (0:w1211:dbl)
        n317 = Round To Nearest(number=w1211) -> (nearest integer value=w1210:dbl)
        n318 = Add(x=w1210, y=11.0) -> (x+y=w1208:dbl)
        n319 = To Unsigned Byte Integer(number=w1208) -> (unsigned 8bit integer=w1207:u8)
      }
      frame "drainrangemode" {
        n320 = Delete From Array(array=w1256, index=0 ("Index")) -> (deleted portion=w1257:string)  [unwired: 1 in, 1 out]
        n321 = case shown="\"f\"" w1257 {
          tunnel: [w1259 w1260 w1261] -> w1246
          frame "a", Default {
            w1259 = u16 0 items=["Auto", "Limited", "Fixed"] ("Gate Range\nmode 2")
          }
          frame "f" {
            w1260 = u16 2 items=["Auto", "Limited", "Fixed"] ("Gate Range\nmode 2")
          }
          frame "l" {
            w1261 = u16 1 items=["Auto", "Limited", "Fixed"] ("Gate Range\nmode 2")
          }
        }
      }
      frame "Error", Default {
      }
      frame "logfile" {
        n322 = Number To Decimal String(number=w1314) -> (decimal integer string=w1349:string)  [unwired: 1 in]
        n323 = Concatenate Strings(w1348, "logfile" ("Substring"), w1349, w1312, ".txt" ("Substring")) -> (w1346:string)
        n324 = String To Path(string=w1346) -> (path=w1319:path)
        n325 = Unbundle(w1345) -> ("integration time"=w1344:u32, "Short/Long integration time"=w1343:dbl, "hold time (sec)"=w1342:dbl, "delay time (sec)"=w1341:dbl, "Step Time (0 disables)"=w1340:dbl, "sweep method"=w1339:u16, "Pulse period"=w1338:dbl, "Base voltage"=w1337:dbl, "Pulse width"=w1336:dbl)
        n326 = Build Array(w1344, w1343, w1342, w1341, w1340, w1339, w1338, w1337, w1336, w1330, w1331, w1332, w1333, w1334, w1335) -> (w1323:dbl[])
        n327 = Insert Into Array(array=dbl[][] [] ("Input Array"), new element=w1323) -> (w1322:dbl[][])  [unwired: 2 in]
        n328 = call <vilib>:"compatOverwrite.vi"("overwrite (F)"=TRUE) -> ("overwrite?"=w1317:T8)
        n329 = Open/Create/Replace File(file path (use dialog)=w1319, error in=w1321, operation (0:open)=w1317) -> (refnum out=w1327:refnum<file>, error out=w1326:errorcluster)  [unwired: 3 in, 1 out]
        n330 = call "4155C Write array to file.vi"("Byte Stream File Refnum"=w1327, "Header"=string[] ["Int Time", "Short/Long Itime", "Hold time", "Delay time", "Step time", "Sweep method", "Pulse period", "Base Voltage", "Pulse width", "Drain compliance", "Gate compliance", "Gate range mode", "Gate range", "S/D range mode", "S/D range"], "Data Array"=w1322, "error in (no error)"=w1326) -> ("dup refnum"=w1329:refnum<file>, "error out"=w1328:errorcluster)  [unwired: 1 in]
        n331 = Close File(refnum=w1329, error in=w1328) -> (error out=w1320:errorcluster)  [unwired: 1 out]
      }
      frame "sample" {
        n332 = Number To Decimal String(number=w1372) -> (decimal integer string=w1420:string)  [unwired: 1 in]
        n333 = Fract/Exp String To Number(string=w1417) -> (number=w1378:dbl[])  [unwired: 3 in, 1 out]
        n334 = Concatenate Strings(w1395, "-sample-" ("Substring"), w1420, w1370, ".txt" ("Substring")) -> (w1418:string)
        n335 = Index Array(array=w1378, index=0 ("Index")) -> (element=w1415:dbl)
        n336 = String To Path(string=w1418) -> (path=w1399:path)
        n337 = Index Array(array=w1378, index=2 ("Index")) -> (element=w1411:dbl)
        n338 = Index Array(array=w1378, index=3 ("Index")) -> (element=w1380:dbl)
        n339 = Index Array(array=w1378, index=4 ("Index")) -> (element=w1377:dbl)
        n340 = call "4155C Config Sampling Measurements.vi"("Sampling interval"=w1377, "Sample time"=w1380, "Display on/off"=TRUE, "Timings"=w1386, "Num Points"=w1411, "error in (no error)"=w1422, "Drain Compliance"=w1421, "Gate Compliance"=w1396, "VISA session"=w1423) -> ("error out"=w1424:errorcluster, "dup VISA resource name"=w1425:refnum<visa-resource-name>)  [unwired: 1 in]
        n341 = Index Array(array=w1378, index=1 ("Index")) -> (element=w1412:dbl)
        n342 = call "4155C Take Sample.vi"("Emergency Stop"=w1392, "error in (no error)"=w1424, "Vd"=w1412, "Vg"=w1415, "VISA resource name in"=w1425) -> ("error out"=w1390:errorcluster, "Id"=w1427:dbl[], "Ig"=w1401:dbl[], "VISA Resource Name out"=w1388:refnum<visa-resource-name>, "Is"=w1426:dbl[], "Time"=w1405:dbl[])  [unwired: 1 in]
        n343 = Insert Into Array(array=dbl[][] [] ("Input Array"), new element=w1405) -> (w1404:dbl[][])  [unwired: 2 in]
        n344 = Insert Into Array(array=w1404, new element=w1401) -> (w1403:dbl[][])  [unwired: 2 in]
        n345 = Insert Into Array(array=w1403, new element=w1427) -> (w1402:dbl[][])  [unwired: 2 in]
        n346 = VISA Write(VISA resource name=w1388, write buffer=":DISP ON" ("write buffer (\"\")"), error in (no error)=w1390) -> (VISA resource name out=w1387:refnum<visa-resource-name>, error out=w1389:errorcluster)  [unwired: 1 out]
        n347 = Insert Into Array(array=w1402, new element=w1426) -> (w1394:dbl[][])  [unwired: 2 in]
        n348 = Transpose 2D Array(2D array=w1394) -> (transposed array=w1393:dbl[][])
        n349 = call <vilib>:"compatOverwrite.vi"("overwrite (F)"=TRUE) -> ("overwrite?"=w1375:T8)
        n350 = Open/Create/Replace File(file path (use dialog)=w1399, error in=w1389, operation (0:open)=w1375) -> (refnum out=w1408:refnum<file>, error out=w1407:errorcluster)  [unwired: 3 in, 1 out]
        n351 = call "4155C Write array to file.vi"("Byte Stream File Refnum"=w1408, "Header"=string[] ["Time /s", "Ig /A", "Id /A", "Is /A"], "Data Array"=w1393, "error in (no error)"=w1407) -> ("dup refnum"=w1410:refnum<file>, "error out"=w1409:errorcluster)  [unwired: 1 in]
        n352 = Close File(refnum=w1410, error in=w1409) -> (error out=w1397:errorcluster)  [unwired: 1 out]
      }
      frame "samplei" {
        n353 = Number To Decimal String(number=w1449) -> (decimal integer string=w1500:string)  [unwired: 1 in]
        n354 = Concatenate Strings(w1479, "-samplei-" ("Substring"), w1500, w1448, ".txt" ("Substring")) -> (w1498:string)
        n355 = Fract/Exp String To Number(string=w1497) -> (number=w1464:dbl[])  [unwired: 3 in, 1 out]
        n356 = String To Path(string=w1498) -> (path=w1482:path)
        n357 = Index Array(array=w1464, index=4 ("Index")) -> (element=w1458:dbl)
        n358 = Index Array(array=w1464, index=3 ("Index")) -> (element=w1459:dbl)
        n359 = Index Array(array=w1464, index=1 ("Index")) -> (element=w1461:dbl)
        n360 = Index Array(array=w1464, index=0 ("Index")) -> (element=w1462:dbl)
        n361 = Index Array(array=w1464, index=2 ("Index")) -> (element=w1460:dbl)
        n362 = call "4155C Config SamplingI Measurements.vi"("Sample time"=w1460, "Display on/off"=TRUE, "Timings"=w1471, "Num Points"=w1461, "error in (no error)"=w1502, "Sampling interval"=w1459, "VISA session"=w1503) -> ("error out"=w1504:errorcluster, "dup VISA resource name"=w1505:refnum<visa-resource-name>)  [unwired: 3 in]
        n363 = call "4155C Take SampleI.vi"("Emergency Stop"=w1476, "error in (no error)"=w1504, "Idg 2"=w1462, "Vdg compliance 2"=w1458, "VISA resource name in"=w1505) -> ("error out"=w1474:errorcluster, "Idg"=w1507:dbl[], "Vdg"=w1484:dbl[], "VISA Resource Name out"=w1472:refnum<visa-resource-name>, "Is"=w1506:dbl[], "Time"=w1488:dbl[])  [unwired: 1 in]
        n364 = Insert Into Array(array=dbl[][] [] ("Input Array"), new element=w1488) -> (w1487:dbl[][])  [unwired: 2 in]
        n365 = Insert Into Array(array=w1487, new element=w1484) -> (w1486:dbl[][])  [unwired: 2 in]
        n366 = Insert Into Array(array=w1486, new element=w1507) -> (w1485:dbl[][])  [unwired: 2 in]
        n367 = VISA Write(VISA resource name=w1472, write buffer=":DISP ON" ("write buffer (\"\")"), error in (no error)=w1474) -> (VISA resource name out=w1457:refnum<visa-resource-name>, error out=w1473:errorcluster)  [unwired: 1 out]
        n368 = Insert Into Array(array=w1485, new element=w1506) -> (w1478:dbl[][])  [unwired: 2 in]
        n369 = call <vilib>:"compatOverwrite.vi"("overwrite (F)"=TRUE) -> ("overwrite?"=w1452:T8)
        n370 = Open/Create/Replace File(file path (use dialog)=w1482, error in=w1473, operation (0:open)=w1452) -> (refnum out=w1491:refnum<file>, error out=w1490:errorcluster)  [unwired: 3 in, 1 out]
        n371 = Transpose 2D Array(2D array=w1478) -> (transposed array=w1477:dbl[][])
        n372 = call "4155C Write array to file.vi"("Byte Stream File Refnum"=w1491, "Header"=string[] ["Time /s", "Vdg /V", "Idg /A", "Is /A"], "Data Array"=w1477, "error in (no error)"=w1490) -> ("dup refnum"=w1493:refnum<file>, "error out"=w1492:errorcluster)  [unwired: 1 in]
        n373 = Close File(refnum=w1493, error in=w1492) -> (error out=w1455:errorcluster)  [unwired: 1 out]
        n374 = VISA Write(VISA resource name=w1457, write buffer=";:PAGE:SCON:STAN OFF;:PAGE:CHAN:VSU2:DIS;" ("write buffer (\"\")"), error in (no error)=w1455) -> (VISA resource name out=w1453:refnum<visa-resource-name>, error out=w1454:errorcluster)  [unwired: 1 out]
      }
      frame "#" {
        n375 = VISA Write(VISA resource name=w1533, write buffer=":DISP ON" ("write buffer (\"\")"), error in (no error)=w1532) -> (VISA resource name out=w1531:refnum<visa-resource-name>, error out=w1530:errorcluster)  [unwired: 1 out]
      }
      frame "stressV" {
        n376 = Number To Decimal String(number=w1562) -> (decimal integer string=w1603:string)  [unwired: 1 in]
        n377 = Concatenate Strings(w1587, "-stressV-" ("Substring"), w1603, w1561, ".txt" ("Substring")) -> (w1601:string)
        n378 = Fract/Exp String To Number(string=w1600) -> (number=w1573:dbl[])  [unwired: 3 in, 1 out]
        n379 = String To Path(string=w1601) -> (path=w1591:path)
        n380 = Index Array(array=w1573, index=3 ("Index")) -> (element=w1570:dbl)
        n381 = Index Array(array=w1573, index=1 ("Index")) -> (element=w1568:dbl)
        n382 = Index Array(array=w1573, index=0 ("Index")) -> (element=w1567:dbl)
        n383 = Index Array(array=w1573, index=4 ("Index")) -> (element=w1572:dbl)
        n384 = Index Array(array=w1573, index=2 ("Index")) -> (element=w1569:dbl)
        n385 = call "4155C Config V Stress.vi"("VISA session"=w1606, "ID compliance"=w1570, "VD"=w1568, "VG"=w1567, "IG compliance"=w1569, "error in (no error)"=w1605, "Display on/off"=TRUE) -> ("dup VISA resource name"=w1608:refnum<visa-resource-name>, "error out"=w1607:errorcluster)
        n386 = call "4155C Apply Stress.vi"("error in (no error)"=w1607, "Duration"=w1572, "Emergency Stop"=w1586, "VISA resource name in"=w1608) -> ("error out"=w1584:errorcluster, "VISA Resource Name out"=w1582:refnum<visa-resource-name>)
        n387 = VISA Write(VISA resource name=w1582, write buffer=":DISP ON" ("write buffer (\"\")"), error in (no error)=w1584) -> (VISA resource name out=w1581:refnum<visa-resource-name>, error out=w1583:errorcluster)  [unwired: 1 out]
        n388 = call <vilib>:"compatOverwrite.vi"("overwrite (F)"=TRUE) -> ("overwrite?"=w1566:T8)
        n389 = Open/Create/Replace File(file path (use dialog)=w1591, error in=w1583, operation (0:open)=w1566) -> (refnum out=w1594:refnum<file>, error out=w1593:errorcluster)  [unwired: 3 in, 1 out]
        n390 = call "4155C Write array to file.vi"("Byte Stream File Refnum"=w1594, "Header"=string[] ["V stress completed successfully", ""], "error in (no error)"=w1593) -> ("dup refnum"=w1596:refnum<file>, "error out"=w1595:errorcluster)  [unwired: 2 in]
        n391 = Close File(refnum=w1596, error in=w1595) -> (error out=w1589:errorcluster)  [unwired: 1 out]
      }
      frame "stressI" {
        n392 = Number To Decimal String(number=w1629) -> (decimal integer string=w1666:string)  [unwired: 1 in]
        n393 = Concatenate Strings(w1650, "-stressI-" ("Substring"), w1666, w1628, ".txt" ("Substring")) -> (w1664:string)
        n394 = Fract/Exp String To Number(string=w1663) -> (number=w1638:dbl[])  [unwired: 3 in, 1 out]
        n395 = Index Array(array=w1638, index=1 ("Index")) -> (element=w1634:dbl)
        n396 = Index Array(array=w1638, index=0 ("Index")) -> (element=w1635:dbl)
        n397 = call "4155C Config I Stress.vi"("VISA session"=w1669, "IDG"=w1635, "VDG compliance"=w1634, "error in (no error)"=w1668, "Display on/off"=TRUE) -> ("dup VISA resource name"=w1671:refnum<visa-resource-name>, "error out"=w1670:errorcluster)
        n398 = Index Array(array=w1638, index=2 ("Index")) -> (element=w1636:dbl)
        n399 = String To Path(string=w1664) -> (path=w1654:path)
        n400 = call "4155C Apply Stress.vi"("error in (no error)"=w1670, "Duration"=w1636, "Emergency Stop"=w1649, "VISA resource name in"=w1671) -> ("error out"=w1647:errorcluster, "VISA Resource Name out"=w1645:refnum<visa-resource-name>)
        n401 = VISA Write(VISA resource name=w1645, write buffer=":DISP ON" ("write buffer (\"\")"), error in (no error)=w1647) -> (VISA resource name out=w1644:refnum<visa-resource-name>, error out=w1646:errorcluster)  [unwired: 1 out]
        n402 = call <vilib>:"compatOverwrite.vi"("overwrite (F)"=TRUE) -> ("overwrite?"=w1633:T8)
        n403 = Open/Create/Replace File(file path (use dialog)=w1654, error in=w1646, operation (0:open)=w1633) -> (refnum out=w1657:refnum<file>, error out=w1656:errorcluster)  [unwired: 3 in, 1 out]
        n404 = call "4155C Write array to file.vi"("Byte Stream File Refnum"=w1657, "Header"=string[] ["I stress completed successfully", ""], "error in (no error)"=w1656) -> ("dup refnum"=w1659:refnum<file>, "error out"=w1658:errorcluster)  [unwired: 2 in]
        n405 = Close File(refnum=w1659, error in=w1658) -> (error out=w1652:errorcluster)  [unwired: 1 out]
      }
      frame "vsu2pulse" {
        n406 = Number To Decimal String(number=w1692) -> (decimal integer string=w1727:string)  [unwired: 1 in]
        n407 = Concatenate Strings(w1712, "-vsu2-" ("Substring"), w1727, w1691, ".txt" ("Substring")) -> (w1725:string)
        n408 = Fract/Exp String To Number(string=w1724) -> (number=w1700:dbl[])  [unwired: 3 in, 1 out]
        n409 = String To Path(string=w1725) -> (path=w1716:path)
        n410 = Index Array(array=w1700, index=1 ("Index")) -> (element=w1699:dbl)
        n411 = Index Array(array=w1700, index=0 ("Index")) -> (element=w1697:dbl)
        n412 = call "4155C Config VSU2 Stress.vi"("error in (no error)"=w1729, "VSU2"=w1697, "Display on/off"=TRUE, "VISA session"=w1730) -> ("error out"=w1731:errorcluster, "dup VISA resource name"=w1732:refnum<visa-resource-name>)
        n413 = call "4155C Apply Stress.vi"("error in (no error)"=w1731, "Duration"=w1699, "Emergency Stop"=w1711, "VISA resource name in"=w1732) -> ("error out"=w1709:errorcluster, "VISA Resource Name out"=w1707:refnum<visa-resource-name>)
        n414 = VISA Write(VISA resource name=w1707, write buffer=":DISP ON" ("write buffer (\"\")"), error in (no error)=w1709) -> (VISA resource name out=w1706:refnum<visa-resource-name>, error out=w1708:errorcluster)  [unwired: 1 out]
        n415 = call <vilib>:"compatOverwrite.vi"("overwrite (F)"=TRUE) -> ("overwrite?"=w1696:T8)
        n416 = Open/Create/Replace File(file path (use dialog)=w1716, error in=w1708, operation (0:open)=w1696) -> (refnum out=w1719:refnum<file>, error out=w1718:errorcluster)  [unwired: 3 in, 1 out]
        n417 = call "4155C Write array to file.vi"("Byte Stream File Refnum"=w1719, "Header"=string[] ["VSU2 pulse completed successfully", ""], "error in (no error)"=w1718) -> ("dup refnum"=w1721:refnum<file>, "error out"=w1720:errorcluster)  [unwired: 2 in]
        n418 = Close File(refnum=w1721, error in=w1720) -> (error out=w1714:errorcluster)  [unwired: 1 out]
      }
      frame "sample-fpp" {
        w1764 = string[] ["Time /s", "Id VgVd /A", "Ig VgVd /A", "Vp1 VgVd /V", "Vp2 VgVd /V"] ("Header")
        w1768 = "%d" ("format string")
        n419 = Number To Decimal String(number=w1753) -> (decimal integer string=w1816:string)  [unwired: 1 in]
        n420 = Fract/Exp String To Number(string=w1813) -> (number=w1801:dbl[])  [unwired: 3 in, 1 out]
        n421 = Concatenate Strings(w1807, "-samplefpp-" ("Substring"), w1816, w1752, ".txt" ("Substring")) -> (w1814:string)
        n422 = String To Path(string=w1814) -> (path=w1776:path)
        n423 = Index Array(array=w1801, index=0 ("Index")) -> (element=w1762:dbl)
        n424 = Index Array(array=w1801, index=1 ("Index")) -> (element=w1761:dbl)
        n425 = Index Array(array=w1801, index=2 ("Index")) -> (element=w1809:dbl)
        n426 = Index Array(array=w1801, index=3 ("Index")) -> (element=w1799:dbl)
        n427 = call "4155C Config Sampling Measurements FPP.vi"("VISA session"=w1819, "Num Points"=w1809, "Vg"=w1762, "Display on/off"=TRUE, "Gate Compliance"=w1808, "Drain Compliance"=w1817, "Standby"="Standby", "error in (no error)"=w1818, "Timings"=w1806, "Vd"=w1761, "Sample time"=w1799) -> ("dup VISA resource name"=w1778:refnum<visa-resource-name>, "error out"=w1777:errorcluster)  [unwired: 3 in]
        n428 = Number To Decimal String(number=w1762) -> (decimal integer string=w1788:string)  [unwired: 1 in]
        n429 = call "4155C Take Sample FPP.vi"("VISA resource name in"=w1778, "error in (no error)"=w1777, "Emergency Stop"=w1779) -> ("Time"=w1783:dbl[], "Vp1"=w1793:dbl[], "VISA Resource Name out"=w1759:refnum<visa-resource-name>, "Ig"=w1781:dbl[], "Id"=w1782:dbl[], "Vp2"=w1791:dbl[], "error out"=w1780:errorcluster)  [unwired: 10 in]
        n430 = Insert Into Array(array=dbl[][] [] ("Input Array"), new element=w1783) -> (w1797:dbl[][])  [unwired: 2 in]
        n431 = Number To Decimal String(number=w1761) -> (decimal integer string=w1786:string)  [unwired: 1 in]
        n432 = Insert Into Array(array=w1797, new element=w1782) -> (w1796:dbl[][])  [unwired: 2 in]
        n433 = Concatenate Strings("(Vg = " ("Substring"), w1788, "V, Vd = " ("Substring"), w1786, "V)" ("Substring")) -> (w1784:string)
        n434 = Insert Into Array(array=w1796, new element=w1781) -> (w1795:dbl[][])  [unwired: 2 in]
        n435 = Insert Into Array(array=w1795, new element=w1793) -> (w1792:dbl[][])  [unwired: 2 in]
        n436 = Insert Into Array(array=w1792, new element=w1791) -> (w1760:dbl[][])  [unwired: 2 in]
        n437 = Transpose 2D Array(2D array=w1760) -> (transposed array=w1790:dbl[][])
        n438 = call <vilib>:"compatOverwrite.vi"("overwrite (F)"=TRUE) -> ("overwrite?"=w1757:T8)
        n439 = Open/Create/Replace File(file path (use dialog)=w1776, error in=w1780, operation (0:open)=w1757) -> (refnum out=w1773:refnum<file>, error out=w1774:errorcluster)  [unwired: 3 in, 1 out]
        n440 = Array To Spreadsheet String(array=w1764, 3:w1768) -> (spreadsheet string=w1770:string)  [unwired: 1 in]
        n441 = Search and Replace String(replace all?=TRUE ("replace all? (F)"), input string=w1770, search string="VgVd", replace string=w1784) -> (result string=w1766:string)  [unwired: 4 in, 3 out]
        n442 = Spreadsheet String To Array(format string=w1768, spreadsheet string=w1766, array type (2D Dbl)=w1764) -> (array=w1765:string[])  [unwired: 1 in]
        n443 = call "4155C Write array to file.vi"("Byte Stream File Refnum"=w1773, "Header"=w1765, "Data Array"=w1790, "error in (no error)"=w1774) -> ("dup refnum"=w1771:refnum<file>, "error out"=w1772:errorcluster)  [unwired: 1 in]
        n444 = Close File(refnum=w1771, error in=w1772) -> (error out=w1758:errorcluster)  [unwired: 1 out]
      }
      frame "resample-fpp" {
        w1853 = string[] ["Time /s", "Id VgVd /A", "Ig VgVd /A", "Vp1 VgVd /V", "Vp2 VgVd /V"] ("Header")
        w1857 = "%d" ("format string")
        n445 = Number To Decimal String(number=w1839) -> (decimal integer string=w1897:string)  [unwired: 1 in]
        n446 = Fract/Exp String To Number(string=w1894) -> (number=w1846:dbl[])  [unwired: 3 in, 1 out]
        n447 = Concatenate Strings(w1890, "-resamplefpp-" ("Substring"), w1897, w1840, ".txt" ("Substring")) -> (w1895:string)
        n448 = String To Path(string=w1895) -> (path=w1865:path)
        n449 = Index Array(array=w1846, index=0 ("Index")) -> (element=w1852:dbl)
        n450 = Index Array(array=w1846, index=1 ("Index")) -> (element=w1851:dbl)
        n451 = Number To Decimal String(number=w1852) -> (decimal integer string=w1875:string)  [unwired: 1 in]
        n452 = call "4155C Take Sample FPP.vi"("VISA resource name in"=w1848, "error in (no error)"=w1847, "Emergency Stop"=w1866) -> ("Time"=w1870:dbl[], "Vp1"=w1880:dbl[], "VISA Resource Name out"=w1850:refnum<visa-resource-name>, "Ig"=w1868:dbl[], "Id"=w1869:dbl[], "Vp2"=w1878:dbl[], "error out"=w1867:errorcluster)  [unwired: 10 in]
        n453 = Insert Into Array(array=dbl[][] [] ("Input Array"), new element=w1870) -> (w1884:dbl[][])  [unwired: 2 in]
        n454 = Number To Decimal String(number=w1851) -> (decimal integer string=w1873:string)  [unwired: 1 in]
        n455 = Insert Into Array(array=w1884, new element=w1869) -> (w1883:dbl[][])  [unwired: 2 in]
        n456 = Concatenate Strings("(Vg = " ("Substring"), w1875, "V, Vd = " ("Substring"), w1873, "V)" ("Substring")) -> (w1871:string)
        n457 = Insert Into Array(array=w1883, new element=w1868) -> (w1882:dbl[][])  [unwired: 2 in]
        n458 = Insert Into Array(array=w1882, new element=w1880) -> (w1879:dbl[][])  [unwired: 2 in]
        n459 = Insert Into Array(array=w1879, new element=w1878) -> (w1845:dbl[][])  [unwired: 2 in]
        n460 = call <vilib>:"compatOverwrite.vi"("overwrite (F)"=TRUE) -> ("overwrite?"=w1844:T8)
        n461 = Open/Create/Replace File(file path (use dialog)=w1865, error in=w1867, operation (0:open)=w1844) -> (refnum out=w1862:refnum<file>, error out=w1863:errorcluster)  [unwired: 3 in, 1 out]
        n462 = Array To Spreadsheet String(array=w1853, 3:w1857) -> (spreadsheet string=w1859:string)  [unwired: 1 in]
        n463 = Transpose 2D Array(2D array=w1845) -> (transposed array=w1877:dbl[][])
        n464 = Search and Replace String(replace all?=TRUE ("replace all? (F)"), input string=w1859, search string="VgVd", replace string=w1871) -> (result string=w1855:string)  [unwired: 4 in, 3 out]
        n465 = Spreadsheet String To Array(format string=w1857, spreadsheet string=w1855, array type (2D Dbl)=w1853) -> (array=w1854:string[])  [unwired: 1 in]
        n466 = call "4155C Write array to file.vi"("Byte Stream File Refnum"=w1862, "Header"=w1854, "Data Array"=w1877, "error in (no error)"=w1863) -> ("dup refnum"=w1860:refnum<file>, "error out"=w1861:errorcluster)  [unwired: 1 in]
        n467 = Close File(refnum=w1860, error in=w1861) -> (error out=w1849:errorcluster)  [unwired: 1 out]
      }
      frame "serial" {
        n468 = local read "Termination char\n(0xA = '\\n' = LF)\n(0xD = '\\r' = CR)"() -> (w1925:u8)
        n469 = local read "Enable Termination\nChar (T)"() -> (w1926:bool)
        n470 = Index Array(array=w1933, index=0 ("Index")) -> (element=w1932:string)
        n471 = local read "parity"() -> (w1916:u16)
        n472 = local read "Delay before read (ms)"() -> (w1927:u32)
        n473 = local read "byte count"() -> (w1924:u32)
        n474 = local read "Timeout (ms)"() -> (w1923:u32)
        n475 = local read "VISA resource name"() -> (w1920:refnum<visa-resource-name>)
        n476 = local read "baud rate"() -> (w1919:u32)
        n477 = local read "Serial End Mode for Reads"() -> (w1918:u16)
        n478 = local read "data bits"() -> (w1917:u16)
        n479 = local read "stop bits"() -> (w1922:u16)
        n480 = local read "flow control"() -> (w1921:u16)
        n481 = call "Serial write and read v0.5.vi"("Delay before read (ms)"=w1927, "Termination char\n(0xA = '\\n' = LF)\n(0xD = '\\r' = CR)"=w1925, "Enable Termination\nChar (T)"=w1926, "parity"=w1916, "stop bits"=w1922, "string to write"=w1932, "flow control"=w1921, "byte count"=w1924, "Serial Settings:Serial End Mode for Reads"=w1918, "Timeout (ms)"=w1923, "error in (no error)"=w1938, "VISA resource name"=w1920, "baud rate"=w1919, "data bits"=w1917) -> ("Serial port output"=w1928:string, "error out"=w1937:errorcluster)
        n482 = Build Array (concatenate)(w1928, w1929) -> (w1930:string[])
      }
      frame "pump" {
        # "Time array for valve position"
        # "Time array for absolute plunger position"
        # "Valve position"
        # "Absolute plunger position"
        # "Remove \"_\""
        # "Check if hard stop is pressed."
        # "Check if halt is pressed."
        # "Check if pump is idle. Else halt."
        n483 = Index Array(array=w2003, index=0 ("Index")) -> (element=w1980:string)
        n484 = case shown="\"No error\", Default" w1978 {
          tunnel: w1980 -> [w2039 _ w2041 w2042 w2043 w2044 _ _ w2047 w2048 _]
          tunnel: [w2039 "/1H" w2041 w2042 w2043 w2044 "/1H" "/1H" w2047 w2048 "/1H"] -> w1979
          frame "No error", Default {
          }
          frame "Initialization" {
          }
          frame "Invalid command" {
          }
          frame "Invalid operand" {
          }
          frame "Device not initialized" {
          }
          frame "Internal failure" {
          }
          frame "Plunger overload" {
          }
          frame "Valve overload" {
          }
          frame "Plunger move not allowed" {
          }
          frame "A/D converter failure" {
          }
          frame "Command overflow" {
          }
        }
        n485 = local read "Hard stop pump"() -> (w1982:bool)
        n486 = local read "Halt pump"() -> (w1985:bool)
        n487 = local read "Serial End Mode for Reads"() -> (w1991:u16)
        n488 = local read "flow control"() -> (w1994:u16)
        n489 = local read "stop bits"() -> (w1995:u16)
        n490 = local read "parity"() -> (w1989:u16)
        n491 = local read "Delay before read (ms)"() -> (w2000:u32)
        n492 = local read "byte count"() -> (w1997:u32)
        n493 = local read "Timeout (ms)"() -> (w1996:u32)
        n494 = local read "VISA resource name"() -> (w1993:refnum<visa-resource-name>)
        n495 = local read "baud rate"() -> (w1992:u32)
        n496 = local read "Enable Termination\nChar (T)"() -> (w1999:bool)
        n497 = local read "Termination char\n(0xA = '\\n' = LF)\n(0xD = '\\r' = CR)"() -> (w1998:u8)
        n498 = case shown="True" w1985 {
          tunnel: [w2053 "/1H"] -> w1984
          tunnel: w1979 -> [w2053 _]
          frame False {
          }
          frame True {
            n499 = local write "Halt pump"(FALSE) -> ()
          }
        }
        n500 = case shown="True" w1982 {
          tunnel: [w2050 "/1T"] -> w1983
          tunnel: w1984 -> [w2050 _]
          frame False {
          }
          frame True {
            n501 = local write "Hard stop pump"(FALSE) -> ()
          }
        }
        n502 = local read "data bits"() -> (w1990:u16)
        n503 = String Subset(string=w1974, offset (0)=1) -> (substring=w1972:string)  [unwired: 1 in]
        n504 = call "SPM Pump v0.6.vi"("Termination char\n(0xA = '\\n' = LF)\n(0xD = '\\r' = CR)"=w1998, "Enable Termination\nChar (T)"=w1999, "Timeout (ms)"=w1996, "Serial Settings:Serial End Mode for Reads"=w1991, "byte count"=w1997, "Delay before read (ms)"=w2000, "Time <input>"=w1977, "error in (no error)"=w2008, "Serial port input"=w1983, "VISA resource name"=w1993, "parity"=w1989, "baud rate"=w1992, "stop bits"=w1995, "data bits"=w1990, "flow control"=w1994, "Time units <input>"=w1972) -> ("Input command"=w1971:string, "Serial port data"=w1961:string[], "Pump status"=w1967:string, "Valve position"=w1969:i32, "Absolute plunger position"=w1981:i32, "Serial port"=w1976:string, "error out"=w2007:errorcluster)  [unwired: 1 in, 4 out]
        n505 = case shown="\"?6\"" w1971 {
          tunnel: [w2020 w2028 w2034] -> w1988
          tunnel: w1987 -> [w2020 w2027 w2034]
          tunnel: w1981 -> [_ w2026 _]
          tunnel: w1968 -> [w2019 w2025 w2035]
          tunnel: [w2019 w2025 w2037] -> w1970
          tunnel: w1969 -> [_ _ w2036]
          tunnel: w1966 -> [_ w2024 w2032]
          tunnel: w1965 -> [w2018 w2023 w2033]
          tunnel: [w2018 w2022 w2033] -> w1964
          tunnel: [w2017 w2021 w2031] -> w1963
          tunnel: w1962 -> [w2017 w2021 w2030]
          frame "Q", Default {
          }
          frame "?" {
            n506 = Build Array (concatenate)(w2027, w2026) -> (w2028:i32[])
            n507 = Build Array (concatenate)(w2023, w2024) -> (w2022:i32[])
            n508 = call "4155C Split array.vi"("X data in"=w2022, "Y1 data in"=w2028) -> ("Array of clusters"=w2029:cluster{"Y data in":dbl[], "X data in":dbl[]}[])  [unwired: 5 in, 1 out]
            n509 = local write "Absolute plunger position vs time"(w2029) -> ()
          }
          frame "?6" {
            n510 = Build Array (concatenate)(w2035, w2036) -> (w2037:i32[])
            n511 = Build Array (concatenate)(w2030, w2032) -> (w2031:i32[])
            n512 = call "4155C Split array.vi"("X data in"=w2031, "Y1 data in"=w2037) -> ("Array of clusters"=w2038:cluster{"Y data in":dbl[], "X data in":dbl[]}[])  [unwired: 5 in, 1 out]
            n513 = local write "Valve position vs time"(w2038) -> ()
          }
        }
        n514 = Build Array (concatenate)(w1959, w1961) -> (w1960:string[][])
        n515 = Build Array (concatenate)(w1975, w1976) -> (w2001:string[])
      }
      frame "filename" {
        n516 = Index Array(array=w2057, index=0 ("Index")) -> (element=w2056:string)
      }
    }
    n517 = local read "Time Units"() -> (w69:u16)
    n518 = case shown="2" w69 {
      tunnel: ["Time (Seconds)" ("element") "Time (Minutes)" ("element") "Time (Hours)" ("element")] -> w109
      frame 0 {
      }
      frame 1, Default {
      }
      frame 2 {
      }
    }
    n519 = Build Array(w148, w77, w87, w86, w85, w84, w83, w82, w81, w80, w79, w78, w76) -> (w187:dbl[][])
    n520 = Transpose 2D Array(2D array=w187) -> (transposed array=w186:dbl[][])
    n521 = Concatenate Strings(w128, w71, "Imax_Imin_Ion_Ioff_vs_time.txt" ("Suffix (Imax,Imin,Ion,Ioff)")) -> (w197:string)
    n522 = Build Array(w109, "Is max (A)" ("VAR2 Name"), "Is min (A)" ("VAR2 Name"), "Id max (A)" ("VAR2 Name"), "Id min (A)" ("VAR2 Name"), "Ig max (A)" ("VAR2 Name"), "Ig min (A)" ("VAR2 Name"), "Is on (A)" ("VAR2 Name"), "Is off (A)" ("VAR2 Name"), "Id on (A)" ("VAR2 Name"), "Id off (A)" ("VAR2 Name"), "Ig on (A)" ("VAR2 Name"), "Ig off (A)" ("VAR2 Name")) -> (w192:string[])
    n523 = Array To Spreadsheet String(array=w186, 3:"%e" ("format string")) -> (spreadsheet string=w190:string)  [unwired: 1 in]
    n524 = Array To Spreadsheet String(array=w192, 3:"" ("format string")) -> (spreadsheet string=w191:string)  [unwired: 1 in]
    n525 = String To Path(string=w197) -> (path=w196:path)
    n526 = Build Array(w191, w190) -> (w189:string[])
    n527 = Write to Text File(file (use dialog)=w196, text=w189, error in=w144) -> (refnum out=w198:refnum<file>, error out=w188:errorcluster)  [unwired: 1 in, 1 out]
    n528 = Close File(refnum=w198, error in=w188) -> (error out=w127:errorcluster)  [unwired: 1 out]
    n529 = Build Array(w123, w149) -> (w154:i32[][])
    n530 = Build Array(w109, "Absolute plunger position" ("VAR2 Name")) -> (w157:string[])
    n531 = Transpose 2D Array(2D array=w154) -> (transposed array=w147:i32[][])
    n532 = Array To Spreadsheet String(array=w157, 3:"" ("format string")) -> (spreadsheet string=w156:string)  [unwired: 1 in]
    n533 = Array To Spreadsheet String(array=w147, 3:"%e" ("format string")) -> (spreadsheet string=w153:string)  [unwired: 1 in]
    n534 = Build Array(w156, w153) -> (w159:string[])
    n535 = Concatenate Strings(w128, w71, "plunger_vs_time.txt" ("Suffix (plunger)")) -> (w151:string)
    n536 = String To Path(string=w151) -> (path=w150:path)
    n537 = Write to Text File(file (use dialog)=w150, text=w159, error in=w127) -> (refnum out=w152:refnum<file>, error out=w161:errorcluster)  [unwired: 1 in, 1 out]
    n538 = Close File(refnum=w152, error in=w161) -> (error out=w126:errorcluster)  [unwired: 1 out]
    n539 = Concatenate Strings(w128, w71, "serial_port_output.txt" ("Suffix (serial port log)")) -> (w167:string)
    n540 = String To Path(string=w167) -> (path=w166:path)
    n541 = Build Array(w109, "Serial port input" ("VAR2 Name"), "Pump status" ("VAR2 Name"), "Serial port output: ") -> (w113:string[])
    n542 = Array To Spreadsheet String(array=w119, 3:"" ("format string")) -> (spreadsheet string=w110:string)  [unwired: 1 in]
    n543 = Array To Spreadsheet String(array=w113, 3:"" ("format string")) -> (spreadsheet string=w111:string)  [unwired: 1 in]
    n544 = Build Array(w111, w110) -> (w112:string[])
    n545 = Array To Spreadsheet String(array=w118, 3:"" ("format string")) -> (spreadsheet string=w172:string)  [unwired: 1 in]
    n546 = Write to Text File(file (use dialog)=w166, text=w112, error in=w126) -> (refnum out=w168:refnum<file>, error out=w169:errorcluster)  [unwired: 1 in, 1 out]
    n547 = Close File(refnum=w168, error in=w169) -> (error out=w125:errorcluster)  [unwired: 1 out]
    n548 = local write "Serial port data"(w172) -> ()
    n549 = Build Array(w122, w130) -> (w136:i32[][])
    n550 = Build Array(w109, "Valve port" ("VAR2 Name")) -> (w139:string[])
    n551 = Transpose 2D Array(2D array=w136) -> (transposed array=w131:i32[][])
    n552 = Array To Spreadsheet String(array=w139, 3:"" ("format string")) -> (spreadsheet string=w138:string)  [unwired: 1 in]
    n553 = Array To Spreadsheet String(array=w131, 3:"%e" ("format string")) -> (spreadsheet string=w135:string)  [unwired: 1 in]
    n554 = Build Array(w138, w135) -> (w141:string[])
    n555 = Concatenate Strings(w128, w71, "valve_port_vs_time.txt" ("Suffix (valve)")) -> (w133:string)
    n556 = String To Path(string=w133) -> (path=w132:path)
    n557 = Write to Text File(file (use dialog)=w132, text=w141, error in=w125) -> (refnum out=w134:refnum<file>, error out=w143:errorcluster)  [unwired: 1 in, 1 out]
    n558 = Close File(refnum=w134, error in=w143) -> (error out=w124:errorcluster)  [unwired: 1 out]
  }
  "error out" <- w31
  "Timings Indicator" <- w15
  "Is max" <- w13
  "Id max" <- w13
  "Ig max" <- w13
  "Imax vs time" <- w9
  "I vs Vg" <- w9
  "Imin vs time" <- w9
  "I vs Vd" <- w9
  "Serial port data" <- "" ("Serial port data")
  "Valve position vs time" <- cluster{"Y data in":dbl[], "X data in":dbl[]}[] [] ("Valve position vs time")
  "Is min" <- w12
  "Id min" <- w12
  "Ig min" <- w12
  "Ion vs time" <- w9
  "Ioff vs time" <- w9
  "Is on" <- w11
  "Id on" <- w11
  "Ig on" <- w11
  "Is off" <- w10
  "Id off" <- w10
  "Ig off" <- w10
